vi "ADQUIRI_adq.vi"() -> ()   [LabVIEW 2019]
doc: "Programa que faz a leitura e a gravação em arquivo TXT de 13 canais provenientes da placa da National Instruments."
uses:
  <vilib>/Analysis/baseanly.llb/Mean (DBL).vi
  <vilib>/DAQmx/read.llb/DAQmx Read (Analog 2D DBL NChan NSamp).vi
  formato_aquisicao_global_adq.vi
  comunicacao.vi
  Aplicacao_atual_global_adq.vi
  <vilib>/DAQmx/configure/timing.llb/DAQmx Timing (Sample Clock).vi
  <vilib>/DAQmx/miscellaneous.llb/DAQmx Fill In Error Info.vi
  <vilib>/Utility/file.llb/Read Delimited Spreadsheet (string).vi
  <vilib>/Utility/file.llb/Write Delimited Spreadsheet (string).vi
  <vilib>/Analysis/NI_AALBase.lvlib
panel:
  in  "ValoresEnviados":cluster{"Pfundo[kPa]":dbl}
  out "SKS-NC-CV-006":bool
  out "comunica funcionando":bool
  in  "Valores":T1
  in  "Calibração":bool
  in  "COMUNICA":bool
  in  "data":dbl[][](array[numeric])
  out "DAQmx Task Name":refnum<k21>
  in  "Visualizar":bool
  out "led viewing":bool
  out "Configuração":string
  in  "Pontos No Gráfico":dbl(knob) scale=0.0..3000.0
  in  "Frequência":dbl=3000.0
  out "Ok":bool
  out "OK2":bool
  out "Ok R":bool
  out "OK2 R":bool
  out "P1-P2 RED":bool
  out "P2-P3 RED":bool
  out "P3-P4 RED":bool
  out "P34/L [Pa/m]":dbl
  out "P23/L [Pa/m]":dbl
  out "P12/L [Pa/m]":dbl
  out "Valor Teórico[Pa/m]":dbl
  out "P3-P4 VERDE":bool
  out "P2-P3 VERDE":bool
  out "P1-P2 VERDE":bool
  out "SKM-AI-KF-COR":dbl
  out "SKM-FI-WF":dbl format="%#.2g"
  out "SKM-FIC-KF-COR":dbl format="%#.2g"
  out "Valvulas":T2
  out "VALORES UDP":string[](array[string])
  in  "SAIR":bool
  out "reference out":refnum<vi>
  out "JG(m/s)":dbl
  in  "TempoAquisicao":dbl
  out "JW(m/s)":dbl format="%#.6g"
  out "JK(m/s)":dbl format="%#.6g"
  out "Timer":i32 caption="Elapsed Time (s)"
  in  "STOP":bool
  in  "COMEÇAR":bool
  out "Quantidade de\narquivos adquiridos":i64
  out "LED adquiri":bool
  out "Aquisição Automática":bool
  out "Linha de Teste":bool
  out "Matriz 2":dbl[][](array[numeric])
  out "error out":errorcluster
  in  "SKM-AI-KF_CORIOLI [kg/m³]":dbl
  in  "SKM-FIC-KF_CORIOLI [kg/s]":dbl
  in  "SIW-CV-001":bool
  in  "SIK-CV-001":bool
  in  "Entrada - SKM-FI-WF [CLP]":dbl
  in  "Escala de Calibracao - SKM-FI-WF":cluster{"Escala Max":dbl, "Escala Min":dbl}
  in  "Tab Control":enum32{"Gráfico", "Matriz"}(tab)
  out "Aplicação":string
  in  "Help":bool
  out "Gráfico":dbl[][](graph)
  in  "formato de aquisicao":bool
  out "C1-M corrente":dbl format="%#_4g"
  out "C1-J corrente":dbl format="%#_4g"
  out "C2-M corrente":dbl format="%#_4g"
  out "C2-J corrente":dbl format="%#_4g"
  out "C3-M corrente":dbl format="%#_4g"
  out "C3-J corrente":dbl format="%#_4g"
  out "C4-M corrente":dbl format="%#_4g"
  out "C4-J corrente":dbl format="%#_4g"
  out "P1 corrente":dbl format="%#_4g"
  out "P2 corrente":dbl format="%#_4g"
  out "P3 corrente":dbl format="%#_4g"
  out "P4 corrente":dbl format="%#_4g"
  out "Pfundo corrente":dbl format="%#_4g"
  out "P4(kPa)":dbl format="%#.2g"
  out "P3(kPa)":dbl format="%#.2g"
  out "P2(kPa)":dbl format="%#.2g"
  out "P1(kPa)":dbl format="%#.2g"
  out "Pfundo(kPa)":dbl format="%#.2g"
  out "P4":dbl format="%#_2g"
  out "C4-J":dbl format="%#_2g"
  out "C4-M":dbl format="%#_2g"
  out "C3-J":dbl format="%#_2g"
  out "P3":dbl format="%#_2g"
  out "C3-M":dbl format="%#_2g"
  out "Pfundo":dbl format="%#_2g"
  out "C2-J":dbl format="%#_2g"
  out "P2":dbl format="%#_2g"
  out "C2-M":dbl format="%#_2g"
  out "P1":dbl format="%#_2g"
  out "C1-M":dbl format="%#_2g"
  out "C1-J":dbl format="%#_2g"
  out "Matriz":dbl[][](array[numeric])
  # "[Hz]"
  # "Aquisição"
  # "[s]"
  # "m/s"
  # "m³/s"
  # "CHECK-UP"
  # "m/s"
  # "kg/s"
  # "P1, P3 & P4"
  # "[s]"
  # "m/s"
  # "kg/m³"
  # "P2"
  # "MIN"
  # "MAX"
  # "P1"
  # "kPa"
  # "P2"
  # "kPa"
  # "P3"
  # "kPa"
  # "P4"
  # "kPa"
  # "Pfundo"
  # "kPa"
  # "Variáveis Selecionadas Para Aquisição"
  # "[mA]"
  # "[V]"
  # "[mA]"
  # "[V]"
  # "[mA]"
  # "[V]"
  # "[kPa]"
  # "[mA]"
  # "[V]"
  # "[mA]"
  # "[V]"
  # "[mA]"
  # "[V]"
  # "[kPa]"
  # "[mA]"
  # "[V]"
  # "[mA]"
  # "[V]"
  # "[mA]"
  # "[V]"
  # "[kPa]"
  # "[mA]"
  # "[V]"
  # "[mA]"
  # "[V]"
  # "[mA]"
  # "[V]"
  # "[kPa]"
  # "[mA]"
  # "[V]"
  # "[kPa]"
  # "WIRELESS"
  # "NATIONAL"
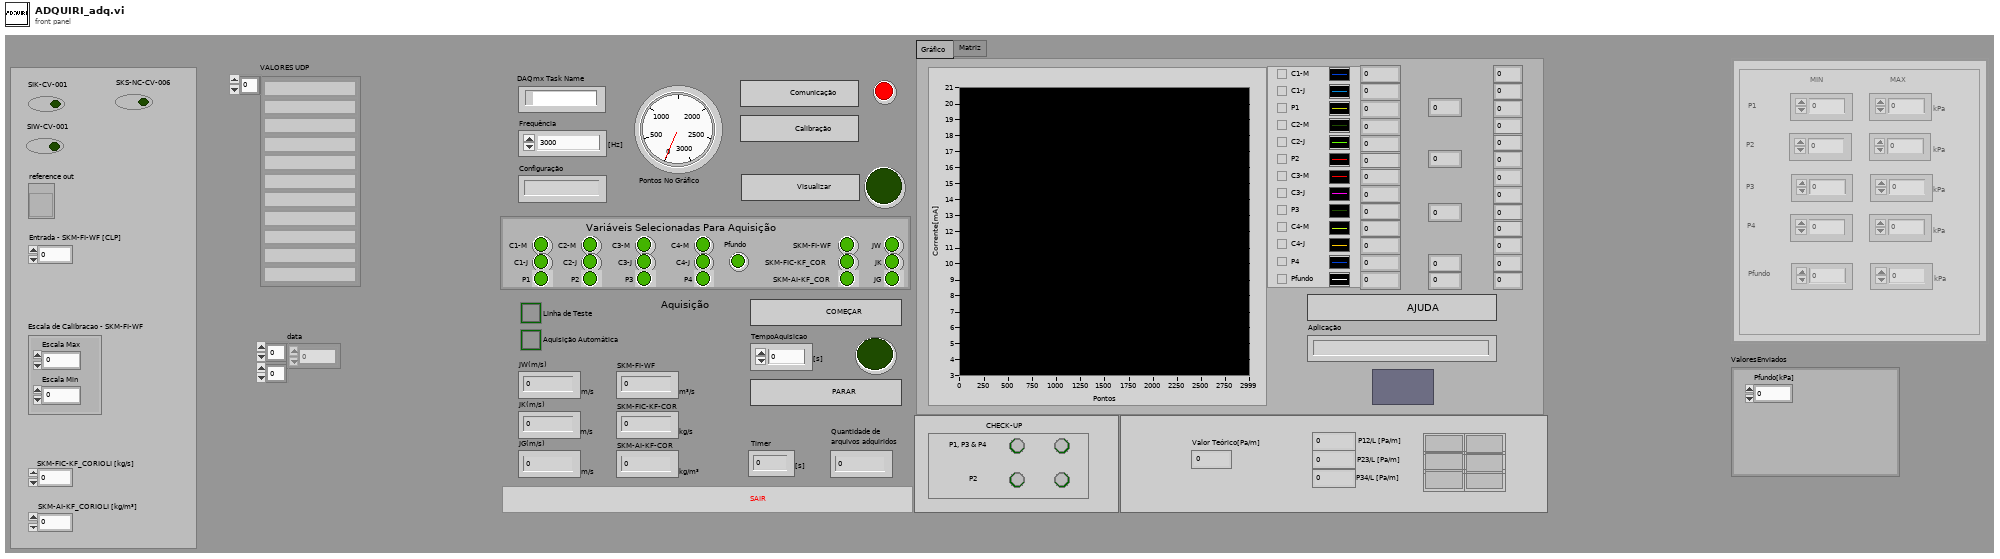
[diagram p1: front panel]
types:
  T1 = cluster{"P1 MIN":i32, "P1 MAX":i32, "P2 MIN":i32, "P2 MAX":i32, "P3 MIN":i32, "P3 MAX":i32, "P4 MIN":i32, "P4 MAX":i32, "Pfu MIN":i32, "Pfu MAX":i32}
  T2 = cluster{"C1-M":bool, "C1-J":bool, "P1":bool, "C2-M":bool, "C2-J":bool, "P2":bool, "C3-M":bool, "C3-J":bool, "P3":bool, "C4-M":bool, "C4-J":bool, "P4":bool, "Pfundo":bool, "JW":bool, "JK":bool, "JG":bool, "SKM-FI-WF":bool, "SKM-FIC-KF_COR":bool, "SKM-AI-KF_COR":bool}
  T3 = enum8{"Enabled", "Disabled", "Disabled and Grayed Out"}
  T4 = enum32{"Invalid", "Standard", "Closed", "Hidden", "Minimized", "Maximized"}
  T5 = enum32{"Bad", "Idle", "Run top level", "Running"}
  T6 = typedef "NI_Matrix.lvlib/RealMatrix.ctl" = dbl[][]
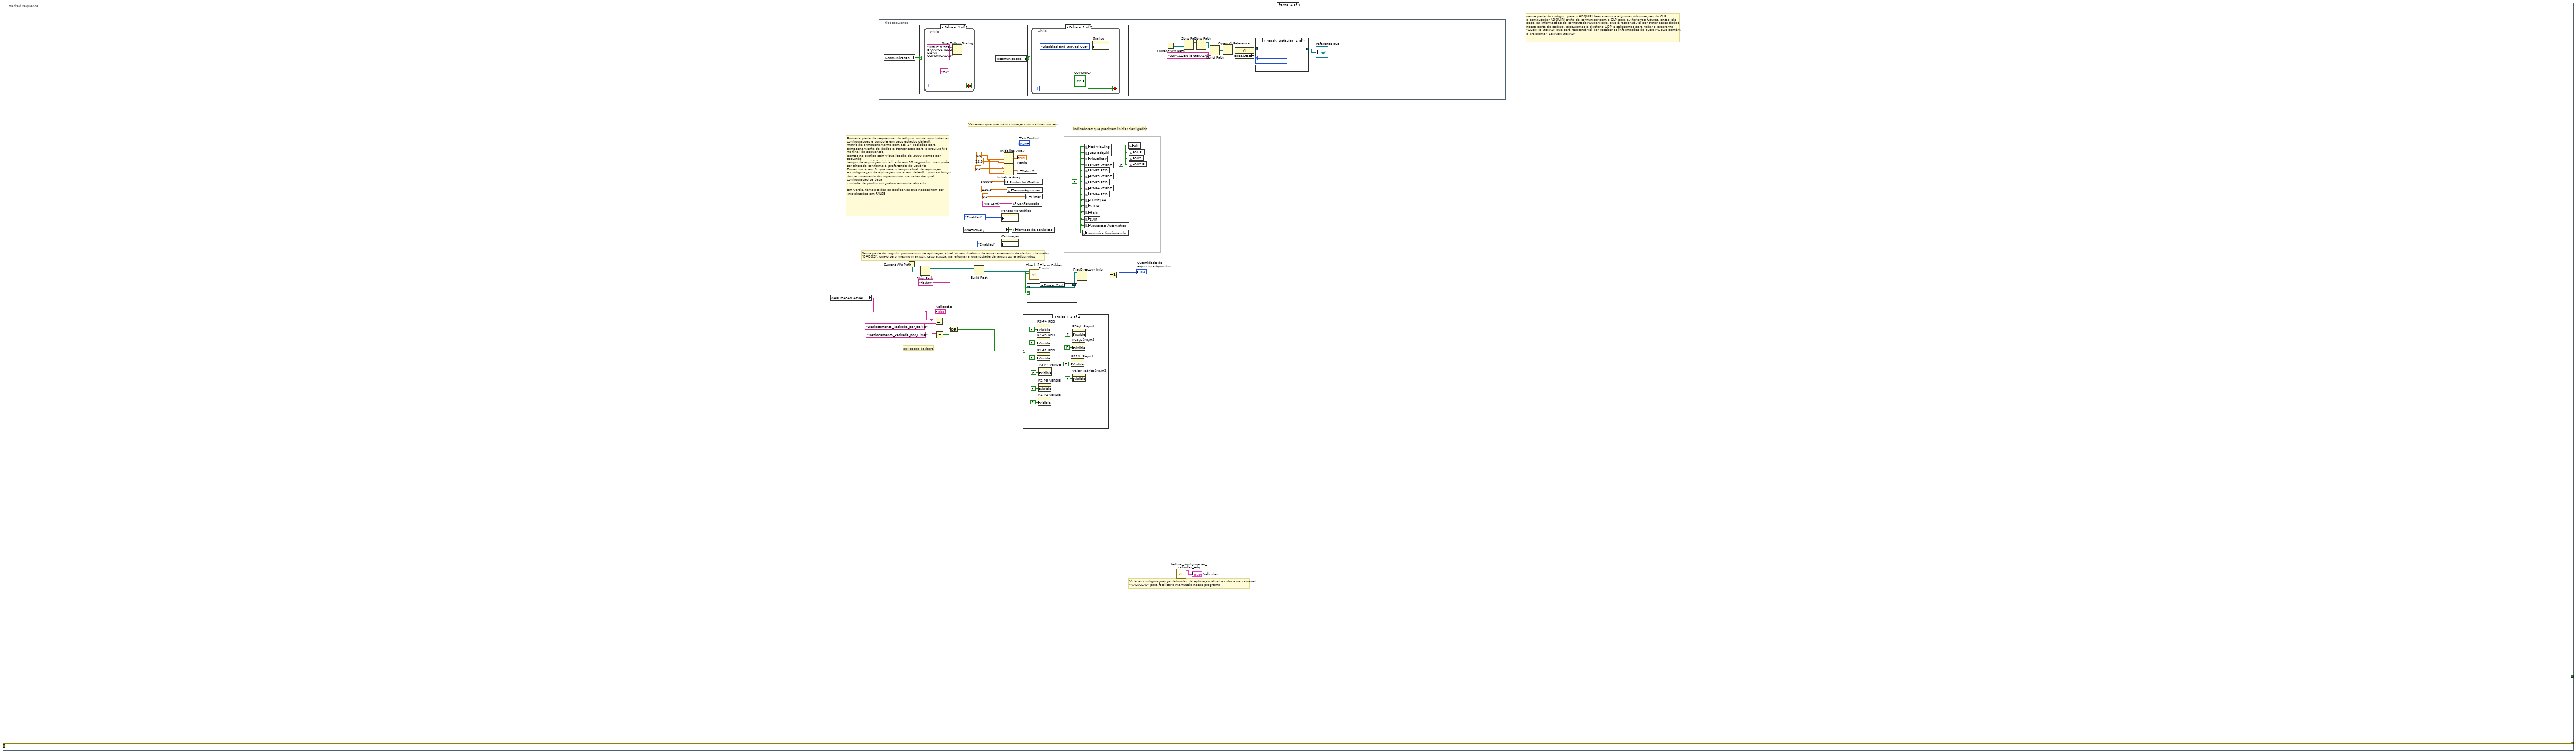
[diagram p2: hidden frame]
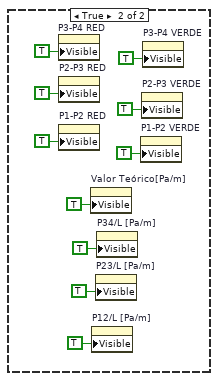
[diagram p3: hidden frame]
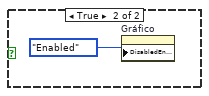
[diagram p5: hidden frame]
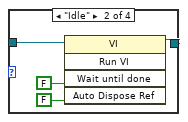
[diagram p6: hidden frame]
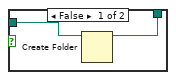
[diagram p9: hidden frame]
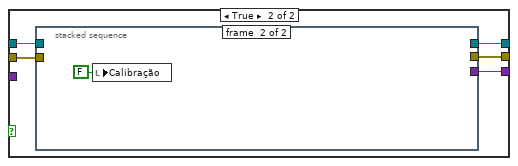
[diagram p10: hidden frame]
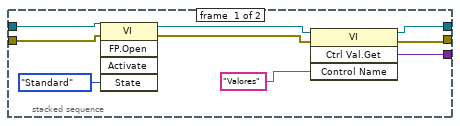
[diagram p11: hidden frame]
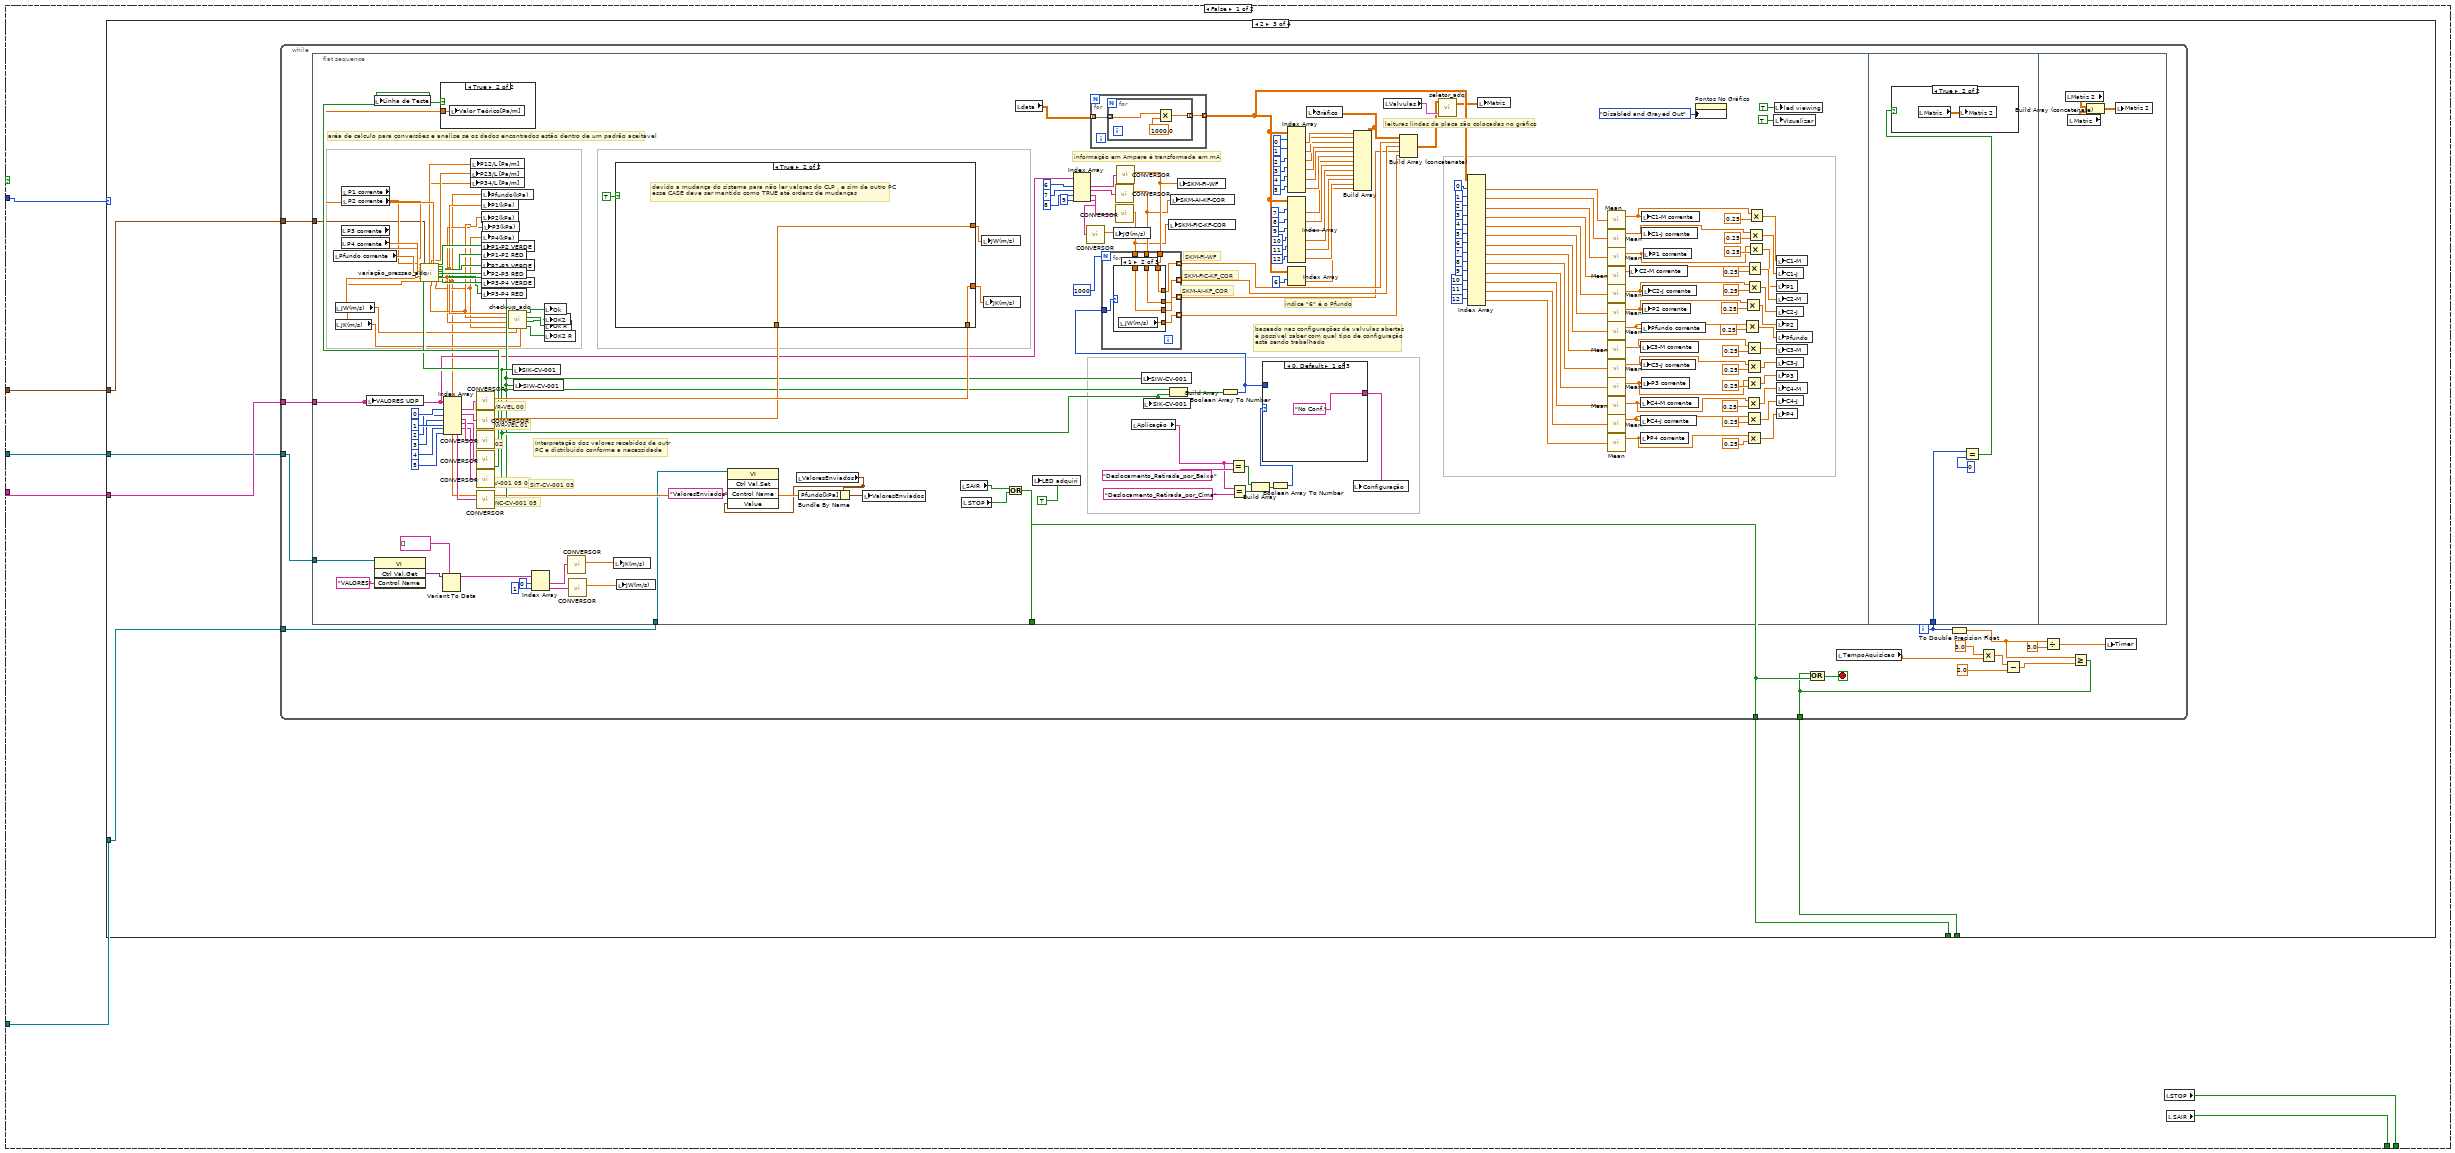
[diagram p12: hidden frame]
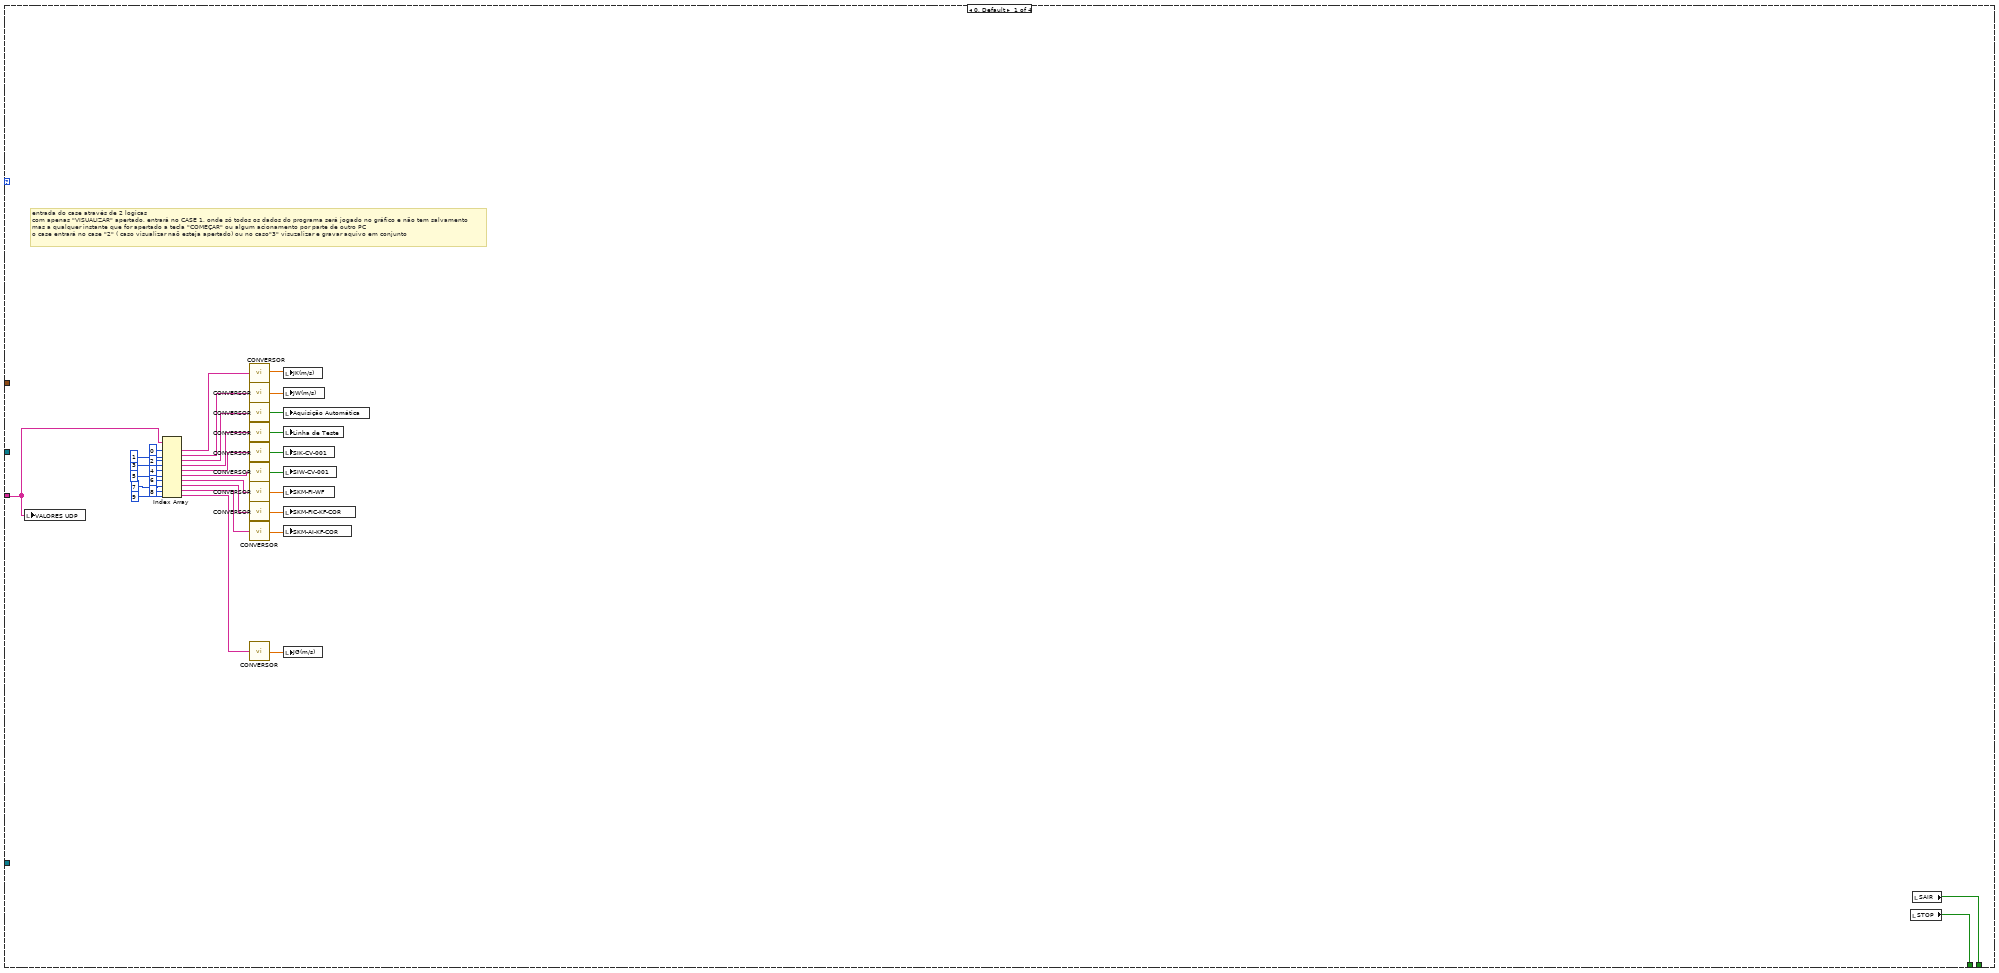
[diagram p13: hidden frame]
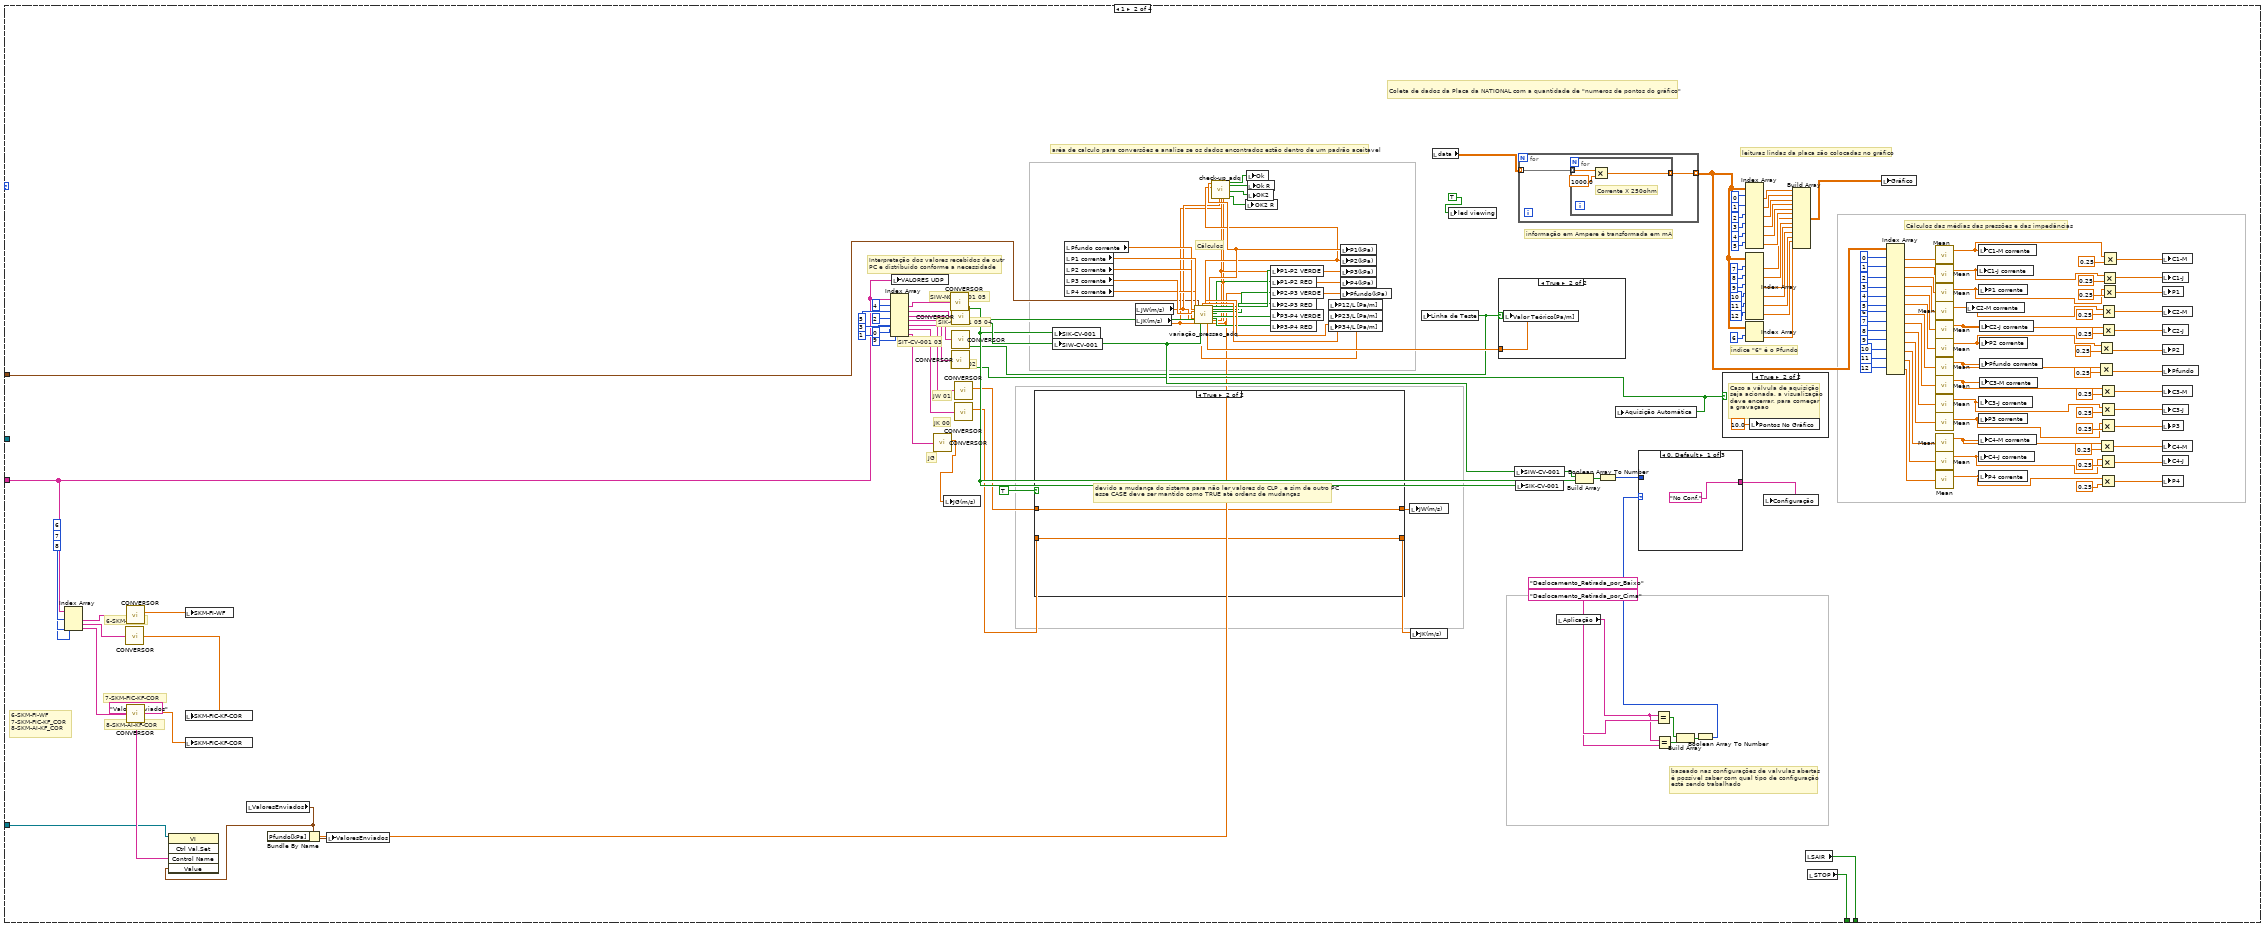
[diagram p14: hidden frame]
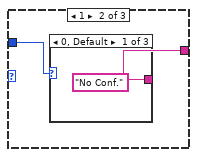
[diagram p15: hidden frame]
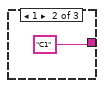
[diagram p16: hidden frame]
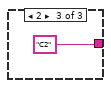
[diagram p17: hidden frame]
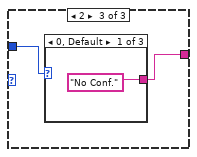
[diagram p18: hidden frame]
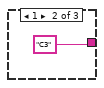
[diagram p19: hidden frame]
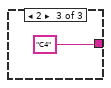
[diagram p20: hidden frame]
diagram:
  # "Abre a VI"
  n1 = property class="VI"("Front Panel.Open"=TRUE ("Front Panel Window:Open")) -> (error out=w1:errorcluster)  [unwired: 2 in, 1 out]
  n2 = flat-sequence {
    tunnel: [w5] -> w3
    tunnel: w1 -> [w4]
    tunnel: w3 -> [w1971]
    frame #0 {
      n3 = while {
        shift-right: [w8] -> w5
        shift-left: w4 -> [w7]
        stop <- w6 stop-if-true
        # "Loop responsável\npor manter o \nadquiri rodando\n\nmesmo após uma \naquisição ou \nvisualização dos \ndados\no adquiri não irá\nfechar, e irá \naguardar um novo\ncomando"
        n4 = stacked-sequence {
          tunnel: [w30 _ _ _] -> w8
          tunnel: w7 -> [w30 _ _ _]
          tunnel: [_ _ _ w1964] -> w6
          frame #0 {
            w20 = FALSE ("Visualisa")
            w36 = 0.0 ("element")
            w13 = FALSE ("Visualisa")
            w31 = 16.0 ("element")
            w37 = 0.0 ("element")
            # "aplicação barbara"
            # "Nessa parte do cógido, procuramos na aplicação atual, o seu diretório de armazenamento de dados, chamado\n\"DADOS\", cria-o se o mesmo n existir, caso exista, irá retornar a quantidade de arquivos ja adquiridos"
            # "Vi lê as configurações já definidas da aplicação atual e coloca na vairável\n\"VALVULAS\" para facilitar o manuzeio nesse programa"
            # "nessa parte do código , para o ADQUIRI teer acesso a algumas informações do CLP\no computador ADQUIRI evita de comunicar com o CLP para evitar erros futuros, então ele\npega as informações do computador SuperTorre, que é responsável por tratar esses dados\nnessa parte do código, procuramos o diretório UDP e colocamos para rodar o programa\n\"CLIENTE GERAL\" que será responsável por receber as informações do outro PC que contém\no programa\" SERVER GERAL\""
            # "Primeria parte da sequencia  do adquiri, inicia com todas as \nconfigurações e controle em seus estados default\nmatriz de armazenamento com até 17 posições para \narmazenamento de dados e transcrissão para o arquivo txt \nno final da sequencia\npontos no grafico com visualização de 3000 pontos por \nsegundo\ntempo de aquisição inicializado em 30 segundos, mas pode \nser alterado conforme a preferÊncia do usuário\nTimer inicia em 0, que será o tempo atual de aquisição\na configuração da aplicação inicia em default , pois ao longo \ndos acionamento do supervisório, irá saber de qual \nconfiguração se trata\ncontrole de pontos no gráfico encontra ativado\n\nem verde, temos todos os booleanos que necessitam ser\ninicializados em FALSE"
            # "Variáveis que precisam começar com valores iniciais"
            # "indicadores que precisam iniciar desligados"
            n5 = global read "Aplicacao_atual_global_adq.vi" "APLICACAO ATUAL"() -> (w9:string)
            "Aplicação" <- w9
            n6 = flat-sequence {
              frame #0 {
                n7 = global read "comunicacao.vi" "comunicacao"() -> (w60:bool)
                n8 = case shown="False" w60 {
                  frame False {
                    n9 = while {
                      stop <- w61 stop-if-true
                      n10 = One Button Dialog(message="LIGUE O SERVER E \nAPÓS ISSO,\n LIGAR COMUNICAÇÃO", button name ("OK")="OK") -> (true=w61:bool)
                    }
                  }
                  frame True {
                  }
                }
              }
              frame #1 {
                n11 = global read "comunicacao.vi" "comunicacao"() -> (w64:bool)
                n12 = case shown="False" w64 {
                  frame False {
                    n13 = while {
                      stop <- "COMUNICA" stop-if-true
                      n14 = property on="Gráfico" class="WFGraph (strict)"("DisabledEnum"=T3."Disabled and Grayed Out" ("Disabled")) -> ()  [unwired: 2 in, 2 out]
                    }
                  }
                  frame True {
                    n15 = property on="Gráfico" class="WFGraph (strict)"("DisabledEnum"=T3."Enabled" ("Disabled")) -> ()  [unwired: 2 in, 2 out]
                  }
                }
              }
              frame #2 {
                n16 = Current VI's Path() -> (path=w73:path)
                n17 = Strip Path(path=w73) -> (stripped path=w74:path)  [unwired: 1 out]
                n18 = Strip Path(path=w74) -> (stripped path=w75:path)  [unwired: 1 out]
                n19 = Build Path(base path=w75, name or relative path="UDP\\CLIENTE GERAL.vi") -> (appended path=w76:path)
                n20 = Open VI Reference(vi path=w76) -> (vi reference=w69:refnum<vi>)  [unwired: 5 in, 1 out]
                n21 = property class="VI"(reference=w69) -> (reference out=w70:refnum<vi>, "Exec.State"=w71:T5)  [unwired: 1 in, 1 out]
                n22 = case shown="\"Bad\", Default" w71 {
                  tunnel: w70 -> [w77 w79 w82 w83]
                  tunnel: [w77 w78 w82 w83] -> w68
                  frame "Bad", Default {
                  }
                  frame "Idle" {
                    n23 = invoke class="VI" method="Run VI"(reference=w79, "Wait until done"=FALSE ("Wait Until Done"), "Auto Dispose Ref"=FALSE ("Auto Dispose Reference")) -> (reference out=w78:refnum<vi>)  [unwired: 2 in, 4 out]
                  }
                  frame "Run top level" {
                  }
                  frame "Running" {
                  }
                }
                "reference out" <- w68
              }
            }
            n24 = Current VI's Path() -> (path=w29:path)
            n25 = Strip Path(path=w29) -> (stripped path=w28:path)  [unwired: 1 out]
            n26 = Equal?(x=w9, y="Deslocamento_Retirada_por_Baixo") -> (x = y?=w17:bool)
            n27 = Equal?(x=w9, y="Deslocamento_Retirada_por_Cima") -> (x = y?=w16:bool)
            n28 = Or(x=w17, y=w16) -> (x .or. y?=w15:bool)
            n29 = global read "formato_aquisicao_global_adq.vi" "NATIONAL/\nWIRELESS"() -> (w21:bool)
            n30 = Build Path(base path=w28, name or relative path="dados") -> (appended path=w24:path)
            n31 = property on="Pontos No Gráfico" class="Knob (strict)"("DisabledEnum"=T3."Enabled" ("Disabled")) -> ()  [unwired: 2 in, 2 out]
            n32 = property on="Calibração" class="Bool (strict)"("DisabledEnum"=T3."Enabled" ("Disabled")) -> ()  [unwired: 2 in, 2 out]
            n33 = Initialize Array(w37, w37, w31) -> (→"Matriz":dbl[][])
            n34 = Initialize Array(w36, w36, w31) -> (w35:dbl[][])
            n35 = local write "Pontos No Gráfico"(3000.0 ("Pontos no gráfico")) -> ()
            n36 = local write "TempoAquisicao"(120.0 ("Acquisition time")) -> ()
            n37 = local write "Configuração"("No Conf." ("Configuration")) -> ()
            n38 = local write "formato de aquisicao"(w21) -> ()
            n39 = local write "Matriz 2"(w35) -> ()
            n40 = case shown="False" w15 {
              frame False {
                n41 = property on="P3-P4 RED" class="Bool (strict)"("Visible"=FALSE) -> ()  [unwired: 2 in, 2 out]
                n42 = property on="P2-P3 RED" class="Bool (strict)"("Visible"=FALSE) -> ()  [unwired: 2 in, 2 out]
                n43 = property on="P1-P2 RED" class="Bool (strict)"("Visible"=FALSE) -> ()  [unwired: 2 in, 2 out]
                n44 = property on="P1-P2 VERDE" class="Bool (strict)"("Visible"=FALSE) -> ()  [unwired: 2 in, 2 out]
                n45 = property on="P2-P3 VERDE" class="Bool (strict)"("Visible"=FALSE) -> ()  [unwired: 2 in, 2 out]
                n46 = property on="P3-P4 VERDE" class="Bool (strict)"("Visible"=FALSE) -> ()  [unwired: 2 in, 2 out]
                n47 = property on="P12/L [Pa/m]" class="DigNum (strict)"("Visible"=FALSE) -> ()  [unwired: 2 in, 2 out]
                n48 = property on="P23/L [Pa/m]" class="DigNum (strict)"("Visible"=FALSE) -> ()  [unwired: 2 in, 2 out]
                n49 = property on="P34/L [Pa/m]" class="DigNum (strict)"("Visible"=FALSE) -> ()  [unwired: 2 in, 2 out]
                n50 = property on="Valor Teórico[Pa/m]" class="DigNum (strict)"("Visible"=FALSE) -> ()  [unwired: 2 in, 2 out]
              }
              frame True {
                n51 = property on="P3-P4 RED" class="Bool (strict)"("Visible"=TRUE) -> ()  [unwired: 2 in, 2 out]
                n52 = property on="P2-P3 RED" class="Bool (strict)"("Visible"=TRUE) -> ()  [unwired: 2 in, 2 out]
                n53 = property on="P1-P2 RED" class="Bool (strict)"("Visible"=TRUE) -> ()  [unwired: 2 in, 2 out]
                n54 = property on="Valor Teórico[Pa/m]" class="DigNum (strict)"("Visible"=TRUE) -> ()  [unwired: 2 in, 2 out]
                n55 = property on="P12/L [Pa/m]" class="DigNum (strict)"("Visible"=TRUE) -> ()  [unwired: 2 in, 2 out]
                n56 = property on="P23/L [Pa/m]" class="DigNum (strict)"("Visible"=TRUE) -> ()  [unwired: 2 in, 2 out]
                n57 = property on="P34/L [Pa/m]" class="DigNum (strict)"("Visible"=TRUE) -> ()  [unwired: 2 in, 2 out]
                n58 = property on="P1-P2 VERDE" class="Bool (strict)"("Visible"=TRUE) -> ()  [unwired: 2 in, 2 out]
                n59 = property on="P2-P3 VERDE" class="Bool (strict)"("Visible"=TRUE) -> ()  [unwired: 2 in, 2 out]
                n60 = property on="P3-P4 VERDE" class="Bool (strict)"("Visible"=TRUE) -> ()  [unwired: 2 in, 2 out]
              }
            }
            n61 = local write "Timer"(0.0 ("Timer")) -> ()
            n62 = call <vilib>:"Check if File or Folder Exists.vi"("path"=w24) -> ("file or folder exists?"=w27:bool, "dup path"=w26:path)  [unwired: 8 in, 1 out]
            n63 = case shown="True" w27 {
              tunnel: w26 -> [w85 w86]
              tunnel: [w84 w86] -> w25
              frame False {
                n64 = Create Folder(path (use dialog)=w85) -> (created path=w84:path)  [unwired: 2 in, 2 out]
              }
              frame True {
              }
            }
            n65 = File/Directory Info(path=w25) -> (size=w12:i64)  [unwired: 1 in, 6 out]
            n66 = local write "comunica funcionando"(w13) -> ()
            n67 = local write "led viewing"(w13) -> ()
            n68 = local write "LED adquiri"(w13) -> ()
            n69 = local write "Visualizar"(w13) -> ()
            n70 = local write "P1-P2 VERDE"(w13) -> ()
            n71 = local write "P1-P2 RED"(w13) -> ()
            n72 = local write "P2-P3 VERDE"(w13) -> ()
            n73 = local write "P2-P3 RED"(w13) -> ()
            n74 = local write "P3-P4 VERDE"(w13) -> ()
            n75 = local write "P3-P4 RED"(w13) -> ()
            n76 = local write "COMEÇAR"(w13) -> ()
            n77 = local write "STOP"(w13) -> ()
            n78 = local write "Help"(w13) -> ()
            n79 = local write "SAIR"(w13) -> ()
            n80 = local write "Aquisição Automática"(w13) -> ()
            n81 = Decrement(x=w12) -> (x-1=→"Quantidade de\narquivos adquiridos":i64)
            n82 = local write "Ok"(w20) -> ()
            n83 = local write "Ok R"(w20) -> ()
            n84 = local write "OK2"(w20) -> ()
            n85 = local write "OK2 R"(w20) -> ()
            n86 = call "leitura_configuracao_valvulas_adq.vi"() -> ("Valvulas"=→"Valvulas":T2)  [unwired: 6 in]
          }
          frame #1 {
            # "nessa etapa do programa, pegamos as referências dessas Vi\n\"LEITURA VALORES CLIENTE\" E \"CLIENTE GERAL\" que JÁ ESTÃO\nRODANDO EM OFF\ncom as refências em mãos, iremos jagá-las para dentro do loop"
            n87 = Current VI's Path() -> (path=w101:path)
            n88 = Current VI's Path() -> (path=w112:path)
            n89 = Strip Path(path=w112) -> (stripped path=w113:path)  [unwired: 1 out]
            n90 = Strip Path(path=w101) -> (stripped path=w95:path)  [unwired: 1 out]
            n91 = Strip Path(path=w113) -> (stripped path=w90:path)  [unwired: 1 out]
            n92 = Build Path(base path=w95, name or relative path="calibracao_adq.vi") -> (appended path=w99:path)
            n93 = Build Path(base path=w90, name or relative path="UDP\\ENVIA VALORES-CLIENTE.vi") -> (appended path=w89:path)
            n94 = Build Path(base path=w90, name or relative path="UDP\\LEITURA VALORES CLIENTE.vi") -> (appended path=w114:path)
            n95 = Build Path(base path=w90, name or relative path="UDP\\CLIENTE GERAL.vi") -> (appended path=w109:path)
            n96 = Open VI Reference(vi path=w89) -> (vi reference=w87:refnum<vi>)  [unwired: 5 in, 1 out]
            n97 = Open VI Reference(vi path=w99, error in (no error)=errorcluster {"status"=FALSE, "code"=0, "source"=""}) -> (vi reference=w98:refnum<vi>, error out=w97:errorcluster)  [unwired: 4 in]
            n98 = Open VI Reference(vi path=w114) -> (vi reference=w110:refnum<vi>)  [unwired: 5 in, 1 out]
            n99 = Open VI Reference(vi path=w109) -> (vi reference=w107:refnum<vi>)  [unwired: 5 in, 1 out]
            n100 = invoke class="VI" method="Run VI"(reference=w98, error in=w97, "Wait until done"=FALSE ("Wait Until Done"), "Auto Dispose Ref"=TRUE ("Auto Dispose Reference")) -> (reference out=w103:refnum<vi>, error out=w102:errorcluster)  [unwired: 1 in, 3 out]
            n101 = invoke class="VI" method="Ctrl Val.Get"(reference=w103, error in=w102, "Control Name"="Valores") -> (reference out=w93:refnum<vi>, error out=w92:errorcluster, "Get Control Value Variant"=w91:variant)  [unwired: 1 in, 1 out]
            n102 = while {
              tunnel: w110 -> [w115]
              tunnel: w107 -> [w141]
              shift-right: [w129] -> w94
              shift-left: w93 -> [w125]
              shift-right: [w128] -> _
              shift-left: w92 -> [w126]
              shift-right: [w124] -> _
              shift-left: w91 -> [w127]
              tunnel: w87 -> [w116]
              stop <- w156 stop-if-true
              w151 = FALSE ("visu led")
              # "10"
              # "national = TRUE"
              # "9"
              # "8"
              # "7"
              # "6"
              # "5"
              # "4"
              # "3"
              # "2"
              # "1"
              # "0"
              # "acionamento automático recebido de outro\nPC"
              # "Default dos botões"
              # "Caso as configurações não desejam\nincluir alguma velocidade na aquisição\na mesma será desabilitada"
              # "Coleta os valores das variáveis enviadas abaixo\nos valores são devolvidos na mesma ordem"
              # "Envia para o programa de comunicação com o outro computador\numa lista de nomes de variáveis que o ADQUIRE nessecita \nos nomes precisam ser enviados em array de STRING para o funcionamento\ndo programa de comunicação."
              # "ADQ 02"
              n103 = local read "Valvulas"() -> (w145:T2)
              n104 = local write "Ok R"(w151) -> ()
              n105 = local write "led viewing"(w151) -> ()
              n106 = local write "OK2"(w151) -> ()
              n107 = local write "OK2 R"(w151) -> ()
              n108 = local write "Ok"(w151) -> ()
              n109 = case shown="True" "Help" {
                frame False {
                  # "Botão Help destinado a abrir documentos e pesquisas relacionadas\nele também abre uma janela explicando sucintamente o objetivo do \nprograma ADQUIRE"
                }
                frame True {
                  n110 = stacked-sequence {
                    frame #0 {
                      n111 = Current VI's Path() -> (path=w1906:path)
                      n112 = Current VI's Path() -> (path=w1900:path)
                      n113 = Strip Path(path=w1906) -> (stripped path=w1905:path)  [unwired: 1 out]
                      n114 = Strip Path(path=w1900) -> (stripped path=w1899:path)  [unwired: 1 out]
                      n115 = Build Path(base path=w1905, name or relative path="Help_difinicao_adq.vi") -> (appended path=w1903:path)
                      n116 = Build Path(base path=w1899, name or relative path="help_pdfs_adq.vi") -> (appended path=w1897:path)
                      n117 = Open VI Reference(vi path=w1903) -> (vi reference=w1910:refnum<vi>, error out=w1909:errorcluster)  [unwired: 5 in]
                      n118 = Open VI Reference(vi path=w1897) -> (vi reference=w1908:refnum<vi>, error out=w1907:errorcluster)  [unwired: 5 in]
                      n119 = invoke class="VI" method="Run VI"(reference=w1910, error in=w1909, "Wait until done"=FALSE ("Wait Until Done"), "Auto Dispose Ref"=FALSE ("Auto Dispose Reference")) -> ()  [unwired: 1 in, 5 out]
                      n120 = invoke class="VI" method="Run VI"(reference=w1908, error in=w1907, "Wait until done"=FALSE ("Wait Until Done"), "Auto Dispose Ref"=FALSE ("Auto Dispose Reference")) -> ()  [unwired: 1 in, 5 out]
                    }
                    frame #1 {
                      n121 = local write "Help"(FALSE ("Help")) -> ()
                    }
                  }
                }
              }
              n122 = Unbundle By Name(w145) -> ("JW"=w146:bool, "JK"=w147:bool, "JG"=w148:bool)
              n123 = case shown="False" "Calibração" {
                tunnel: [w161 w169] -> w129
                tunnel: [w162 w168] -> w128
                tunnel: [w163 w167] -> w124
                tunnel: w125 -> [w160 w166]
                tunnel: w126 -> [w159 w165]
                tunnel: w127 -> [_ _]
                frame False {
                  n124 = invoke class="VI" method="Ctrl Val.Get"(reference=w160, error in=w159, "Control Name"="Valores") -> (reference out=w161:refnum<vi>, error out=w162:errorcluster, "Get Control Value Variant"=w163:variant)  [unwired: 1 in, 1 out]
                }
                frame True {
                  n125 = stacked-sequence {
                    tunnel: [w174 _] -> w169
                    tunnel: [w173 _] -> w168
                    tunnel: [w172 _] -> w167
                    tunnel: w166 -> [w171 _]
                    tunnel: w165 -> [w170 _]
                    frame #0 {
                      n126 = invoke class="VI" method="FP.Open"(reference=w171, error in=w170, "State"=T4."Standard") -> (reference out=w176:refnum<vi>, error out=w175:errorcluster)  [unwired: 2 in, 3 out]
                      n127 = invoke class="VI" method="Ctrl Val.Get"(reference=w176, error in=w175, "Control Name"="Valores") -> (reference out=w174:refnum<vi>, error out=w173:errorcluster, "Get Control Value Variant"=w172:variant)  [unwired: 1 in, 1 out]
                    }
                    frame #1 {
                      n128 = local write "Calibração"(FALSE ("Calibração")) -> ()
                    }
                  }
                }
              }
              n129 = case shown="True" w146 {
                frame False {
                  n130 = property on="JW(m/s)" class="DigNum (strict)"("DisabledEnum"=T3."Disabled and Grayed Out" ("Disabled")) -> ()  [unwired: 2 in, 2 out]
                }
                frame True {
                  n131 = property on="JW(m/s)" class="DigNum (strict)"("DisabledEnum"=T3."Enabled" ("Disabled")) -> ()  [unwired: 2 in, 2 out]
                }
              }
              n132 = case shown="True" w147 {
                frame False {
                  n133 = property on="JK(m/s)" class="DigNum (strict)"("DisabledEnum"=T3."Disabled and Grayed Out" ("Disabled")) -> ()  [unwired: 2 in, 2 out]
                }
                frame True {
                  n134 = property on="JK(m/s)" class="DigNum (strict)"("DisabledEnum"=T3."Enabled" ("Disabled")) -> ()  [unwired: 2 in, 2 out]
                }
              }
              n135 = case shown="True" w148 {
                frame False {
                  n136 = property on="JG(m/s)" class="DigNum (strict)"("DisabledEnum"=T3."Disabled and Grayed Out" ("Disabled")) -> ()  [unwired: 2 in, 2 out]
                }
                frame True {
                  n137 = property on="JG(m/s)" class="DigNum (strict)"("DisabledEnum"=T3."Enabled" ("Disabled")) -> ()  [unwired: 2 in, 2 out]
                }
              }
              n138 = invoke class="VI" method="Ctrl Val.Get"(reference=w115, "Control Name"="VALORES") -> ("Get Control Value Variant"=w144:variant)  [unwired: 2 in, 3 out]
              n139 = property on="Gráfico" class="WFGraph (strict)"("DisabledEnum"=T3."Enabled" ("Disabled")) -> ()  [unwired: 2 in, 2 out]
              n140 = Variant To Data(type=string[] [] ("Array"), Variant=w144) -> (data=w121:string[])  [unwired: 1 in, 1 out]
              n141 = To Variant(anything=string[] ["JK", "JW", "ADQ", "SIT-NC-CV-001", "SIK-NC-CV-001", "SIW-NC-CV-001", "SKM-FI-WF", "SKM-FIC-KF_COR", "SKM-AI-KF_COR", "JG", "SKS-NC-CV-006"] ("NOMES")) -> (Variant=w136:variant)
              n142 = invoke class="VI" method="Ctrl Val.Set"(reference=w141, "Control Name"="NOMES", "Value"=w136) -> ()  [unwired: 2 in, 5 out]
              n143 = Index Array(array=w121, index=2) -> (element=w139:string)
              n144 = call "CONVERSOR.vi"("String"=w139) -> ("boolean"=w138:bool)  [unwired: 6 in, 3 out]
              "Aquisição Automática" <- w138
              n145 = Not Equal?(x=w121, y="") -> (x != y?=w120:bool[])
              n146 = Get Variant Attribute(Variant=w124, name="Valores") -> ()  [unwired: 2 in, 4 out]
              n147 = Variant To Data(type="Valores", Variant=w124) -> (data=w122:T1)  [unwired: 1 in, 1 out]
              n148 = Index Array(array=w120, index=0) -> (element=→"comunica funcionando":bool)
              n149 = local write "Valores"(w122) -> ()
              n150 = global read "formato_aquisicao_global_adq.vi" "NATIONAL/\nWIRELESS"() -> (w135:bool)
              n151 = global write "formato_aquisicao_global_adq.vi" "NATIONAL/\nWIRELESS"("formato de aquisicao") -> ()
              n152 = Or(x="COMEÇAR", y=w138) -> (x .or. y?=w153:bool)
              n153 = Build Array("Visualizar", w153) -> (w158:bool[])
              n154 = Boolean Array To Number(Boolean array=w158) -> (number=w157:u32)
              n155 = case shown="True" w135 {
                tunnel: w157 -> [w183 w1004]
                tunnel: [w186 w1003] -> w155
                tunnel: [w185 w1002] -> w154
                tunnel: w121 -> [w184 w1001]
                tunnel: w122 -> [w182 w991]
                tunnel: w116 -> [w181 w990]
                tunnel: w115 -> [w180 w989]
                frame False {
                  n156 = case shown="2" w183 {
                    tunnel: [w219 w292 w438 w718] -> _
                    tunnel: [w218 w291 w437 w717] -> _
                    tunnel: w184 -> [w187 w316 w436 w716]
                    tunnel: w182 -> [_ w234 w435 w715]
                    tunnel: w181 -> [_ w222 w434 w714]
                    tunnel: w180 -> [_ _ w433 w713]
                    frame 0, Default {
                      # "entrada do case através de 2 logicas\ncom apenas \"VISUALIZAR\" apertado, entrará no CASE 1, onde só todos os dados do programa será jogado no gráfico e não tem salvamento\nmas a qualquer instante que for apertado a tecla \"COMEÇAR\" ou algum acionamento por parte de outro PC\no case entrará no case \"2\" ( caso visualizar naõ esteja apertado) ou no caso\"3\" visuzalizar e gravar aquivo em conjunto"
                      n157 = local write "VALORES UDP"(w187) -> ()
                      n158 = Index Array(array=w187, index #1=0 ("index"), index #2=1 ("index"), index #3=2 ("index"), index #4=3 ("index"), index #5=4 ("index"), index #6=5 ("index"), index #7=6 ("index"), index #8=7 ("index"), index #9=8 ("index"), index #10=9 ("index")) -> (element #1=w217:string, element #2=w216:string, element #3=w215:string, element #4=w214:string, element #5=w213:string, element #6=w212:string, element #7=w211:string, element #8=w210:string, element #9=w209:string, element #10=w208:string)
                      n159 = call "CONVERSOR.vi"("String"=w217) -> ("float"=w207:dbl)  [unwired: 6 in, 3 out]
                      n160 = call "CONVERSOR.vi"("String"=w216) -> ("float"=w206:dbl)  [unwired: 6 in, 3 out]
                      n161 = call "CONVERSOR.vi"("String"=w215) -> ("boolean"=w205:bool)  [unwired: 6 in, 3 out]
                      n162 = call "CONVERSOR.vi"("String"=w214) -> ("boolean"=w204:bool)  [unwired: 6 in, 3 out]
                      n163 = call "CONVERSOR.vi"("String"=w213) -> ("boolean"=w203:bool)  [unwired: 6 in, 3 out]
                      n164 = call "CONVERSOR.vi"("String"=w212) -> ("boolean"=w202:bool)  [unwired: 6 in, 3 out]
                      n165 = call "CONVERSOR.vi"("String"=w211) -> ("float"=w201:dbl)  [unwired: 6 in, 3 out]
                      n166 = call "CONVERSOR.vi"("String"=w210) -> ("float"=w200:dbl)  [unwired: 6 in, 3 out]
                      n167 = call "CONVERSOR.vi"("String"=w209) -> ("float"=w199:dbl)  [unwired: 6 in, 3 out]
                      n168 = call "CONVERSOR.vi"("String"=w208) -> ("float"=w198:dbl)  [unwired: 6 in, 3 out]
                      n169 = local write "JK(m/s)"(w207) -> ()
                      n170 = local write "JW(m/s)"(w206) -> ()
                      n171 = local write "Aquisição Automática"(w205) -> ()
                      n172 = local write "Linha de Teste"(w204) -> ()
                      n173 = local write "SIK-CV-001"(w203) -> ()
                      n174 = local write "SIW-CV-001"(w202) -> ()
                      n175 = local write "SKM-FI-WF"(w201) -> ()
                      n176 = local write "SKM-FIC-KF-COR"(w200) -> ()
                      n177 = local write "SKM-AI-KF-COR"(w199) -> ()
                      n178 = local write "JG(m/s)"(w198) -> ()
                      n179 = local read "STOP"() -> (w219:bool)
                      n180 = local read "SAIR"() -> (w218:bool)
                    }
                    frame 1 {
                      # "JG"
                      # "6-SKM-FI-WF"
                      # "7-SKM-FIC-KF-COR"
                      # "8-SKM-AI-KF-COR"
                      # "6-SKM-FI-WF\n7-SKM-FIC-KF_COR\n8-SKM-AI-KF_COR"
                      # "indice \"6\" é o Pfundo"
                      # "leituras lindas da placa são colocadas no gráfico"
                      # "baseado nas configurações de valvulas abertas\né possível saber com qual tipo de configuração \nestá sendo trabalhado"
                      # "aréa de calculo para conversões e analise se os dados encontrados estão dentro de um padrão aceitavel"
                      # "Interpretação dos valores recebidos de outr\nPC e distribuido conforme a necessidade"
                      # "informação em Ampere é transformada em mA"
                      # "Coleta de dados da Placa da NATIONAL com a quantidade de \"numeros de pontos do gráfico\""
                      # "ADQ 02"
                      # "SIW-NC-CV-001 05"
                      # "SIK-CV-001 05 04"
                      # "SIT-CV-001 03"
                      # "JW 01"
                      # "JK 00"
                      # "Cálculos das médias das pressões e das impedâncias"
                      # "Cálculos"
                      n181 = Index Array(array=w316, index #1=6 ("index"), index #2=7 ("index"), index #3=8 ("index")) -> (element #1=w312:string, element #2=w311:string, element #3=w310:string)
                      n182 = call "CONVERSOR.vi"("String"=w311) -> ("float"=w295:dbl)  [unwired: 6 in, 3 out]
                      n183 = call "CONVERSOR.vi"("String"=w312) -> ("float"=w296:dbl)  [unwired: 6 in, 3 out]
                      n184 = call "CONVERSOR.vi"("String"=w310) -> ("float"=w294:dbl)  [unwired: 6 in, 3 out]
                      n185 = local write "SKM-FI-WF"(w296) -> ()
                      n186 = local write "SKM-FIC-KF-COR"(w295) -> ()
                      n187 = local write "SKM-FIC-KF-COR"(w294) -> ()
                      n188 = local read "ValoresEnviados"() -> (w223:cluster{"Pfundo[kPa]":dbl})
                      n189 = invoke class="VI" method="Ctrl Val.Set"(reference=w222, "Control Name"="ValoresEnviados", "Value"=w223) -> ()  [unwired: 2 in, 5 out]
                      n190 = Index Array(array=w316, index #1=4 ("index"), index #2=5 ("index"), index #3=3 ("index"), index #4=2 ("index"), index #5=1 ("index"), index #6=0 ("index"), index #7=9 ("index")) -> (element #1=w332:string, element #2=w331:string, element #3=w328:string, element #4=w325:string, element #5=w321:string, element #6=w318:string, element #7=w308:string)
                      n191 = local write "VALORES UDP"(w316) -> ()
                      n192 = call "CONVERSOR.vi"("String"=w308) -> ("float"=w293:dbl)  [unwired: 6 in, 3 out]
                      n193 = local write "JG(m/s)"(w293) -> ()
                      n194 = call "CONVERSOR.vi"("String"=w332) -> ("boolean"=w327:bool)  [unwired: 6 in, 3 out]
                      n195 = call "CONVERSOR.vi"("String"=w325) -> ("boolean"=w324:bool)  [unwired: 6 in, 3 out]
                      n196 = call "CONVERSOR.vi"("String"=w331) -> ("boolean"=w330:bool)  [unwired: 6 in, 3 out]
                      n197 = call "CONVERSOR.vi"("String"=w328) -> ("boolean"=w306:bool)  [unwired: 6 in, 3 out]
                      n198 = call "CONVERSOR.vi"("String"=w321) -> ("float"=w320:dbl)  [unwired: 6 in, 3 out]
                      n199 = call "CONVERSOR.vi"("String"=w318) -> ("float"=w317:dbl)  [unwired: 6 in, 3 out]
                      n200 = case shown="True" TRUE {
                        tunnel: [w408 w423] -> w387
                        tunnel: [w407 w424] -> w386
                        tunnel: w320 -> [_ w424]
                        tunnel: w317 -> [_ w423]
                        frame False {
                          # "Cálculos de valores de velocidade utilizando informações do CLP"
                          # "área"
                          # "área"
                          n201 = local read "SKM-FIC-KF_CORIOLI [kg/s]"() -> (w404:dbl)
                          n202 = local read "SKM-AI-KF_CORIOLI [kg/m³]"() -> (w403:dbl)
                          n203 = local read "Escala de Calibracao - SKM-FI-WF"() -> (w406:cluster{"Escala Max":dbl, "Escala Min":dbl})
                          n204 = local read "Entrada - SKM-FI-WF [CLP]"() -> (w405:dbl)
                          n205 = local read "Escala de Calibracao - SKM-FI-WF"() -> (w414:cluster{"Escala Max":dbl, "Escala Min":dbl})
                          n206 = Unbundle By Name(w406) -> ("Escala Max"=w417:dbl, "Escala Min"=w416:dbl)
                          n207 = Bundle By Name(cluster=w414, "Escala Max"=0.001805556, "Escala Min"=0.0 ("Escala Max")) -> (w415:cluster{"Escala Max":dbl, "Escala Min":dbl})
                          n208 = Divide(x=w404, y=w403) -> (x/y=w422:dbl)
                          n209 = Divide(x=w422, y=0.0005107051557) -> (x/y=w408:dbl)
                          n210 = local write "Escala de Calibracao - SKM-FI-WF"(w415) -> ()
                          n211 = Subtract(x=w417, y=w416) -> (x-y=w418:dbl)
                          n212 = Divide(x=w418, y=4096.0) -> (x/y=w419:dbl)
                          n213 = Multiply(x=w419, y=w405) -> (x*y=w420:dbl)
                          n214 = Add(x=w420, y=w416) -> (x+y=w421:dbl)
                          n215 = Divide(x=w421, y=0.0005107051557) -> (x/y=w407:dbl)
                        }
                        frame True {
                          # "devido a mudança do sistema para não ler valores do CLP , e sim de outro PC\nesse CASE deve ser mantido como TRUE até ordens de mudanças"
                        }
                      }
                      n216 = local write "SIK-CV-001"(w327) -> ()
                      n217 = local write "SIW-CV-001"(w330) -> ()
                      n218 = local read "Pfundo corrente"() -> (w285:dbl)
                      n219 = local read "P1 corrente"() -> (w289:dbl)
                      n220 = local read "P2 corrente"() -> (w288:dbl)
                      n221 = local read "P3 corrente"() -> (w287:dbl)
                      n222 = local read "P4 corrente"() -> (w286:dbl)
                      n223 = local read "JW(m/s)"() -> (w236:dbl)
                      n224 = local read "JK(m/s)"() -> (w235:dbl)
                      n225 = call "variação_pressao_adq.vi"("P1(mA)"=w289, "P2(mA)"=w288, "P3(mA)"=w287, "P4(mA)"=w286, "PFUNDO(mA)"=w285, "JW(m/s)"=w236, "JK(m/s)"=w235, "Valores"=w234, "SIK-CV-001"=w327, "SIW-CV-001"=w330) -> ("P12/L12"=w305:dbl, "P34/L34"=w297:dbl, "P23/L23"=w304:dbl, "P2(kPa)"=w239:dbl, "VALOR TEORICO"=w389:dbl, "P3(kPa)"=w238:dbl, "P1(kPa)"=w240:dbl, "P4(kPa)"=w237:dbl, "P1-P2G"=w303:bool, "P2-P3R"=w302:bool, "P2-P3G"=w301:bool, "P1-P2R"=w300:bool, "P3-P4G"=w299:bool, "P3-P4R"=w298:bool, "PFUNDO(kPa)"=w221:dbl)  [unwired: 3 in]
                      n226 = Bundle By Name(cluster=w223, "Pfundo[kPa]"=w221) -> (w220:cluster{"Pfundo[kPa]":dbl})
                      n227 = local write "ValoresEnviados"(w220) -> ()
                      n228 = call "check-up_adq.vi"("JK(m/s)"=w235, "JW(m/s)"=w236, "P4(kPa)"=w237, "P3(kPa)"=w238, "P2(kPa)"=w239, "P1(kPa)"=w240) -> ("OK 2 R"=w241:bool, "OK 2 G"=w242:bool, "OK RED"=w243:bool, "OK G"=w244:bool)  [unwired: 2 in]
                      n229 = local write "OK2 R"(w241) -> ()
                      n230 = local write "Ok"(w244) -> ()
                      n231 = local write "Ok R"(w243) -> ()
                      n232 = local write "OK2"(w242) -> ()
                      n233 = local write "P1-P2 VERDE"(w303) -> ()
                      n234 = local write "P1-P2 RED"(w300) -> ()
                      n235 = local write "P2-P3 VERDE"(w301) -> ()
                      n236 = local write "P2-P3 RED"(w302) -> ()
                      n237 = local write "P3-P4 VERDE"(w299) -> ()
                      n238 = local write "P3-P4 RED"(w298) -> ()
                      n239 = local write "P12/L [Pa/m]"(w305) -> ()
                      n240 = local write "P23/L [Pa/m]"(w304) -> ()
                      n241 = local write "P34/L [Pa/m]"(w297) -> ()
                      n242 = local write "P1(kPa)"(w240) -> ()
                      n243 = local write "P2(kPa)"(w239) -> ()
                      n244 = local write "P3(kPa)"(w238) -> ()
                      n245 = local write "P4(kPa)"(w237) -> ()
                      n246 = local write "Pfundo(kPa)"(w221) -> ()
                      n247 = local write "JW(m/s)"(w386) -> ()
                      n248 = local write "JK(m/s)"(w387) -> ()
                      n249 = local write "Linha de Teste"(w306) -> ()
                      n250 = local read "data"() -> (w307:dbl[][])
                      n251 = local write "led viewing"(TRUE ("visu led")) -> ()
                      n252 = case shown="True" w306 {
                        tunnel: w389 -> [_ w427]
                        frame False {
                          n253 = local write "Valor Teórico[Pa/m]"(nan) -> ()
                        }
                        frame True {
                          n254 = local write "Valor Teórico[Pa/m]"(w427) -> ()
                        }
                      }
                      n255 = local write "SIW-CV-001"(w330) -> ()
                      n256 = local write "SIK-CV-001"(w327) -> ()
                      n257 = for {
                        tunnel: w307 -> [w428] mode=indexing
                        tunnel: [w429] -> w361 mode=indexing
                        n258 = for {
                          tunnel: w428 -> [w432] mode=indexing
                          tunnel: [w430] -> w429 mode=indexing
                          # "Corrente X 250ohm"
                          n259 = Multiply(x=w432, y=1000.0) -> (x*y=w430:dbl)
                        }
                      }
                      n260 = local read "Aplicação"() -> (w228:string)
                      n261 = Build Array(w330, w327) -> (w388:bool[])
                      n262 = Boolean Array To Number(Boolean array=w388) -> (number=w225:u32)
                      n263 = local write "Aquisição Automática"(w324) -> ()
                      n264 = Equal?(x=w228, y="Deslocamento_Retirada_por_Baixo") -> (x = y?=w230:bool)
                      n265 = Equal?(x=w228, y="Deslocamento_Retirada_por_Cima") -> (x = y?=w229:bool)
                      n266 = Build Array(w230, w229) -> (w231:bool[])
                      n267 = Boolean Array To Number(Boolean array=w231) -> (number=w226:u32)
                      n268 = case shown="0, Default" w226 {
                        tunnel: ["No Conf." w394 w399] -> w227
                        tunnel: w225 -> [_ w393 w398]
                        frame 0, Default {
                        }
                        frame 1 {
                          n269 = case shown="0, Default" w393 {
                            tunnel: ["No Conf." "C1" "C2"] -> w394
                            frame 0, Default {
                            }
                            frame 1 {
                            }
                            frame 2 {
                            }
                          }
                        }
                        frame 2 {
                          n270 = case shown="0, Default" w398 {
                            tunnel: ["No Conf." "C3" "C4"] -> w399
                            frame 0, Default {
                            }
                            frame 1 {
                            }
                            frame 2 {
                            }
                          }
                        }
                      }
                      n271 = case shown="True" w324 {
                        frame False {
                        }
                        frame True {
                          # "Caso a válvula de aquisição\nseja acionada, a visualização \ndeve encerrar, para começar\na gravaçaao"
                          n272 = local write "Pontos No Gráfico"(10.0 ("POINTS IN GRAPH")) -> ()
                        }
                      }
                      n273 = Index Array(array=w361, index (row) #1=0 ("index (row)"), index (row) #2=1 ("index (row)"), index (row) #3=2 ("index (row)"), index (row) #4=3 ("index (row)"), index (row) #5=4 ("index (row)"), index (row) #6=5 ("index (row)")) -> (element #1=w354:dbl[], element #2=w353:dbl[], element #3=w352:dbl[], element #4=w351:dbl[], element #5=w350:dbl[], element #6=w349:dbl[])  [unwired: 6 in]
                      n274 = Index Array(array=w361, index (row) #1=7 ("index (row)"), index (row) #2=8 ("index (row)"), index (row) #3=9 ("index (row)"), index (row) #4=10 ("index (row)"), index (row) #5=11 ("index (row)"), index (row) #6=12 ("index (row)")) -> (element #1=w342:dbl[], element #2=w341:dbl[], element #3=w340:dbl[], element #4=w339:dbl[], element #5=w338:dbl[], element #6=w337:dbl[])  [unwired: 6 in]
                      n275 = Index Array(array=w361, index (row)=6) -> (element=w335:dbl[])  [unwired: 1 in]
                      n276 = local write "Configuração"(w227) -> ()
                      n277 = Build Array(w354, w353, w352, w351, w350, w349, w342, w341, w340, w339, w338, w337, w335) -> (w290:dbl[][])
                      n278 = local read "SAIR"() -> (w291:bool)
                      n279 = local read "STOP"() -> (w292:bool)
                      n280 = local write "Gráfico"(w290) -> ()
                      n281 = Index Array(array=w361, index (row) #1=0 ("index (row)"), index (row) #2=1 ("index (row)"), index (row) #3=2 ("index (row)"), index (row) #4=3 ("index (row)"), index (row) #5=4 ("index (row)"), index (row) #6=5 ("index (row)"), index (row) #7=6 ("index (row)"), index (row) #8=7 ("index (row)"), index (row) #9=8 ("index (row)"), index (row) #10=9 ("index (row)"), index (row) #11=10 ("index (row)"), index (row) #12=11 ("index (row)"), index (row) #13=12 ("index (row)")) -> (element #1=w391:dbl[], element #2=w384:dbl[], element #3=w372:dbl[], element #4=w371:dbl[], element #5=w370:dbl[], element #6=w369:dbl[], element #7=w368:dbl[], element #8=w367:dbl[], element #9=w366:dbl[], element #10=w365:dbl[], element #11=w364:dbl[], element #12=w363:dbl[], element #13=w362:dbl[])  [unwired: 13 in]
                      n282 = call-poly <vilib>:"Mean.vi"("X"=w391) -> ("mean"=w270:dbl)  [unwired: 1 out]
                      n283 = call-poly <vilib>:"Mean.vi"("X"=w384) -> ("mean"=w269:dbl)  [unwired: 1 out]
                      n284 = call-poly <vilib>:"Mean.vi"("X"=w372) -> ("mean"=w268:dbl)  [unwired: 1 out]
                      n285 = call-poly <vilib>:"Mean.vi"("X"=w371) -> ("mean"=w267:dbl)  [unwired: 1 out]
                      n286 = call-poly <vilib>:"Mean.vi"("X"=w370) -> ("mean"=w266:dbl)  [unwired: 1 out]
                      n287 = call-poly <vilib>:"Mean.vi"("X"=w369) -> ("mean"=w265:dbl)  [unwired: 1 out]
                      n288 = call-poly <vilib>:"Mean.vi"("X"=w368) -> ("mean"=w264:dbl)  [unwired: 1 out]
                      n289 = call-poly <vilib>:"Mean.vi"("X"=w367) -> ("mean"=w263:dbl)  [unwired: 1 out]
                      n290 = call-poly <vilib>:"Mean.vi"("X"=w366) -> ("mean"=w262:dbl)  [unwired: 1 out]
                      n291 = call-poly <vilib>:"Mean.vi"("X"=w365) -> ("mean"=w261:dbl)  [unwired: 1 out]
                      n292 = call-poly <vilib>:"Mean.vi"("X"=w364) -> ("mean"=w260:dbl)  [unwired: 1 out]
                      n293 = call-poly <vilib>:"Mean.vi"("X"=w363) -> ("mean"=w259:dbl)  [unwired: 1 out]
                      n294 = call-poly <vilib>:"Mean.vi"("X"=w362) -> ("mean"=w258:dbl)  [unwired: 1 out]
                      n295 = local write "C2-M corrente"(w267) -> ()
                      n296 = local write "C1-J corrente"(w269) -> ()
                      n297 = local write "C1-M corrente"(w270) -> ()
                      n298 = local write "C4-J corrente"(w259) -> ()
                      n299 = local write "P1 corrente"(w268) -> ()
                      n300 = local write "C3-J corrente"(w262) -> ()
                      n301 = local write "P3 corrente"(w261) -> ()
                      n302 = local write "C4-M corrente"(w260) -> ()
                      n303 = local write "P4 corrente"(w258) -> ()
                      n304 = local write "C2-J corrente"(w266) -> ()
                      n305 = local write "P2 corrente"(w265) -> ()
                      n306 = local write "Pfundo corrente"(w264) -> ()
                      n307 = local write "C3-M corrente"(w263) -> ()
                      n308 = Multiply(x=w264, y=0.25) -> (x*y=w248:dbl)
                      n309 = Multiply(x=w265, y=0.25) -> (x*y=w249:dbl)
                      n310 = Multiply(x=w260, y=0.25) -> (x*y=w255:dbl)
                      n311 = Multiply(x=w263, y=0.25) -> (x*y=w247:dbl)
                      n312 = Multiply(x=w262, y=0.25) -> (x*y=w246:dbl)
                      n313 = Multiply(x=w261, y=0.25) -> (x*y=w245:dbl)
                      n314 = Multiply(x=w259, y=0.25) -> (x*y=w256:dbl)
                      n315 = Multiply(x=w258, y=0.25) -> (x*y=w257:dbl)
                      n316 = Multiply(x=w267, y=0.25) -> (x*y=w251:dbl)
                      n317 = Multiply(x=w266, y=0.25) -> (x*y=w250:dbl)
                      n318 = Multiply(x=w269, y=0.25) -> (x*y=w253:dbl)
                      n319 = Multiply(x=w268, y=0.25) -> (x*y=w252:dbl)
                      n320 = Multiply(x=w270, y=0.25) -> (x*y=w254:dbl)
                      n321 = local write "C1-M"(w254) -> ()
                      n322 = local write "C1-J"(w253) -> ()
                      n323 = local write "P1"(w252) -> ()
                      n324 = local write "C2-M"(w251) -> ()
                      n325 = local write "C2-J"(w250) -> ()
                      n326 = local write "P2"(w249) -> ()
                      n327 = local write "Pfundo"(w248) -> ()
                      n328 = local write "C3-M"(w247) -> ()
                      n329 = local write "C3-J"(w246) -> ()
                      n330 = local write "P3"(w245) -> ()
                      n331 = local write "C4-M"(w255) -> ()
                      n332 = local write "C4-J"(w256) -> ()
                      n333 = local write "P4"(w257) -> ()
                    }
                    frame 2 {
                      n334 = while {
                        tunnel: [w454] -> w438
                        tunnel: [w443] -> w437
                        tunnel: w436 -> [w452]
                        tunnel: w435 -> [w441]
                        tunnel: w434 -> [w440]
                        tunnel: w433 -> [w439]
                        i -> [w445]
                        stop <- w453 stop-if-true
                        n335 = flat-sequence {
                          tunnel: [w617] -> w454
                          tunnel: w452 -> [w570]
                          tunnel: w441 -> [w480]
                          tunnel: w440 -> [w467]
                          tunnel: w439 -> [w456]
                          tunnel: w445 -> [w708]
                          frame #0 {
                            # "Interpretação dos valores recebidos de outr\nPC e distribuido conforme a necessidade"
                            # "aréa de calculo para conversões e analise se os dados encontrados estão dentro de um padrão aceitavel"
                            # "baseado nas configurações de valvulas abertas\né possível saber com qual tipo de configuração \nestá sendo trabalhado"
                            # "informação em Ampere é transformada em mA"
                            # "indice \"6\" é o Pfundo"
                            # "leituras lindas da placa são colocadas no gráfico"
                            # "SIW-NC-CV-001 05"
                            # "SIK-CV-001 05 04"
                            # "SIT-CV-001 03"
                            # "ADQ 02"
                            # "SPW-WR-VEL 01"
                            # "SPK-WR-VEL 00"
                            # "SKM-FI-WF"
                            # "SKM-FIC-KF_COR"
                            # "SKM-AI-KF_COR"
                            n336 = local read "Pfundo corrente"() -> (w537:dbl)
                            n337 = local read "JW(m/s)"() -> (w482:dbl)
                            n338 = local read "JK(m/s)"() -> (w481:dbl)
                            n339 = local read "P3 corrente"() -> (w535:dbl)
                            n340 = local read "P4 corrente"() -> (w536:dbl)
                            n341 = local read "P1 corrente"() -> (w533:dbl)
                            n342 = local read "P2 corrente"() -> (w534:dbl)
                            n343 = local write "VALORES UDP"(w570) -> ()
                            n344 = invoke class="VI" method="Ctrl Val.Get"(reference=w456, "Control Name"="VALORES") -> ("Get Control Value Variant"=w460:variant)  [unwired: 2 in, 3 out]
                            n345 = Variant To Data(type=string[] [] ("Array"), Variant=w460) -> (data=w461:string[])  [unwired: 1 in, 1 out]
                            n346 = Index Array(array=w570, index #1=0 ("index"), index #2=1 ("index"), index #3=2 ("index"), index #4=3 ("index"), index #5=4 ("index"), index #6=5 ("index")) -> (element #1=w582:string, element #2=w581:string, element #3=w580:string, element #4=w579:string, element #5=w578:string, element #6=w577:string)
                            n347 = call "CONVERSOR.vi"("String"=w581) -> ("float"=w574:dbl)  [unwired: 6 in, 3 out]
                            n348 = call "CONVERSOR.vi"("String"=w580) -> ()  [unwired: 6 in, 4 out]
                            n349 = call "CONVERSOR.vi"("String"=w578) -> ("boolean"=w572:bool)  [unwired: 6 in, 3 out]
                            n350 = call "CONVERSOR.vi"("String"=w577) -> ("boolean"=w571:bool)  [unwired: 6 in, 3 out]
                            n351 = call "variação_pressao_adq.vi"("P1(mA)"=w533, "P2(mA)"=w534, "P3(mA)"=w535, "P4(mA)"=w536, "PFUNDO(mA)"=w537, "JW(m/s)"=w482, "JK(m/s)"=w481, "Valores"=w480, "SIK-CV-001"=w572, "SIW-CV-001"=w571) -> ("P12/L12"=w540:dbl, "P34/L34"=w538:dbl, "P23/L23"=w539:dbl, "P2(kPa)"=w485:dbl, "VALOR TEORICO"=w547:dbl, "P3(kPa)"=w484:dbl, "P1(kPa)"=w486:dbl, "P4(kPa)"=w483:dbl, "P1-P2G"=w546:bool, "P2-P3R"=w545:bool, "P2-P3G"=w544:bool, "P1-P2R"=w543:bool, "P3-P4G"=w542:bool, "P3-P4R"=w541:bool, "PFUNDO(kPa)"=w469:dbl)  [unwired: 3 in]
                            n352 = local write "P23/L [Pa/m]"(w539) -> ()
                            n353 = local write "P34/L [Pa/m]"(w538) -> ()
                            n354 = local write "P12/L [Pa/m]"(w540) -> ()
                            n355 = call "CONVERSOR.vi"("String"=w582) -> ("float"=w575:dbl)  [unwired: 6 in, 3 out]
                            n356 = call "CONVERSOR.vi"("String"=w579) -> ("boolean"=w573:bool)  [unwired: 6 in, 3 out]
                            n357 = local write "Linha de Teste"(w573) -> ()
                            n358 = case shown="True" w573 {
                              tunnel: w547 -> [_ w683]
                              frame False {
                                n359 = local write "Valor Teórico[Pa/m]"(nan) -> ()
                              }
                              frame True {
                                n360 = local write "Valor Teórico[Pa/m]"(w683) -> ()
                              }
                            }
                            n361 = local write "P1-P2 VERDE"(w546) -> ()
                            n362 = local write "P1-P2 RED"(w543) -> ()
                            n363 = local write "P2-P3 VERDE"(w544) -> ()
                            n364 = local write "P2-P3 RED"(w545) -> ()
                            n365 = local write "P3-P4 VERDE"(w542) -> ()
                            n366 = local write "P3-P4 RED"(w541) -> ()
                            n367 = local write "Pfundo(kPa)"(w469) -> ()
                            n368 = local write "P1(kPa)"(w486) -> ()
                            n369 = local write "P2(kPa)"(w485) -> ()
                            n370 = local write "P4(kPa)"(w483) -> ()
                            n371 = local write "P3(kPa)"(w484) -> ()
                            n372 = call "check-up_adq.vi"("JK(m/s)"=w481, "JW(m/s)"=w482, "P4(kPa)"=w483, "P3(kPa)"=w484, "P2(kPa)"=w485, "P1(kPa)"=w486) -> ("OK 2 R"=w487:bool, "OK 2 G"=w488:bool, "OK RED"=w489:bool, "OK G"=w490:bool)  [unwired: 2 in]
                            n373 = local write "SIK-CV-001"(w572) -> ()
                            n374 = local write "SIW-CV-001"(w571) -> ()
                            n375 = Index Array(array=w461, index #1=0 ("index"), index #2=1 ("index")) -> (element #1=w462:string, element #2=w463:string)
                            n376 = local write "Ok"(w490) -> ()
                            n377 = local write "OK2"(w488) -> ()
                            n378 = local write "Ok R"(w489) -> ()
                            n379 = local write "OK2 R"(w487) -> ()
                            n380 = call "CONVERSOR.vi"("String"=w462) -> ("float"=w464:dbl)  [unwired: 6 in, 3 out]
                            n381 = call "CONVERSOR.vi"("String"=w463) -> ("float"=w465:dbl)  [unwired: 6 in, 3 out]
                            n382 = local write "JK(m/s)"(w464) -> ()
                            n383 = case shown="True" TRUE {
                              tunnel: [w679 w681] -> w530
                              tunnel: [w672 w680] -> w531
                              tunnel: w575 -> [_ w681]
                              tunnel: w574 -> [_ w680]
                              frame False {
                                n384 = local read "Escala de Calibracao - SKM-FI-WF"() -> (w668:cluster{"Escala Max":dbl, "Escala Min":dbl})
                                n385 = local read "Entrada - SKM-FI-WF [CLP]"() -> (w666:dbl)
                                n386 = local read "Escala de Calibracao - SKM-FI-WF"() -> (w673:cluster{"Escala Max":dbl, "Escala Min":dbl})
                                n387 = Bundle By Name(cluster=w673, "Escala Max"=0.001805556, "Escala Min"=0.0 ("Escala Max")) -> (w674:cluster{"Escala Max":dbl, "Escala Min":dbl})
                                n388 = local write "Escala de Calibracao - SKM-FI-WF"(w674) -> ()
                                n389 = Unbundle By Name(w668) -> ("Escala Max"=w662:dbl, "Escala Min"=w667:dbl)
                                n390 = local read "SKM-AI-KF_CORIOLI [kg/m³]"() -> (w676:dbl)
                                n391 = local read "SKM-FIC-KF_CORIOLI [kg/s]"() -> (w677:dbl)
                                n392 = Subtract(x=w662, y=w667) -> (x-y=w660:dbl)
                                n393 = Divide(x=w660, y=4096.0) -> (x/y=w669:dbl)
                                n394 = Multiply(x=w669, y=w666) -> (x*y=w670:dbl)
                                n395 = Add(x=w670, y=w667) -> (x+y=w671:dbl)
                                n396 = Divide(x=w677, y=w676) -> (x/y=w678:dbl)
                                n397 = Divide(x=w671, y=0.0005107051557) -> (x/y=w672:dbl)
                                n398 = Divide(x=w678, y=0.0005107051557) -> (x/y=w679:dbl)
                              }
                              frame True {
                                # "devido a mudança do sistema para não ler valores do CLP , e sim de outro PC\nesse CASE deve ser mantido como TRUE até ordens de mudanças"
                              }
                            }
                            n399 = local write "JW(m/s)"(w465) -> ()
                            n400 = local read "ValoresEnviados"() -> (w468:cluster{"Pfundo[kPa]":dbl})
                            n401 = invoke class="VI" method="Ctrl Val.Set"(reference=w467, "Control Name"="ValoresEnviados", "Value"=w468) -> ()  [unwired: 2 in, 5 out]
                            n402 = Bundle By Name(cluster=w468, "Pfundo[kPa]"=w469) -> (w466:cluster{"Pfundo[kPa]":dbl})
                            n403 = local write "ValoresEnviados"(w466) -> ()
                            n404 = local read "SAIR"() -> (w615:bool)
                            n405 = local read "STOP"() -> (w616:bool)
                            n406 = local write "JW(m/s)"(w531) -> ()
                            n407 = local write "JK(m/s)"(w530) -> ()
                            n408 = Or(x=w615, y=w616) -> (x .or. y?=w617:bool)
                            n409 = local read "data"() -> (w549:dbl[][])
                            n410 = local write "LED adquiri"(TRUE ("Adquire")) -> ()
                            n411 = Index Array(array=w570, index #1=6 ("index"), index #2=7 ("index"), index #3=8 ("index"), index #4=9 ("index")) -> (element #1=w566:string, element #2=w565:string, element #3=w564:string, element #4=w551:string)
                            n412 = call "CONVERSOR.vi"("String"=w551) -> ("float"=w550:dbl)  [unwired: 6 in, 3 out]
                            n413 = for {
                              tunnel: [w702] -> w618 mode=indexing
                              tunnel: w549 -> [w701] mode=indexing
                              n414 = for {
                                tunnel: w701 -> [w705] mode=indexing
                                tunnel: [w703] -> w702 mode=indexing
                                n415 = Multiply(x=w705, y=1000.0) -> (x*y=w703:dbl)
                              }
                            }
                            n416 = local write "JG(m/s)"(w550) -> ()
                            n417 = call "CONVERSOR.vi"("String"=w565) -> ("float"=w554:dbl)  [unwired: 6 in, 3 out]
                            n418 = call "CONVERSOR.vi"("String"=w564) -> ("float"=w553:dbl)  [unwired: 6 in, 3 out]
                            n419 = call "CONVERSOR.vi"("String"=w566) -> ("float"=w555:dbl)  [unwired: 6 in, 3 out]
                            n420 = local read "Aplicação"() -> (w474:string)
                            n421 = local write "SIW-CV-001"(w571) -> ()
                            n422 = local write "SIK-CV-001"(w572) -> ()
                            n423 = local write "SKM-FIC-KF-COR"(w553) -> ()
                            n424 = Build Array(w571, w572) -> (w646:bool[])
                            n425 = local write "SKM-AI-KF-COR"(w554) -> ()
                            n426 = local write "SKM-FI-WF"(w555) -> ()
                            n427 = Boolean Array To Number(Boolean array=w646) -> (number=w471:u32)
                            n428 = for {
                              N: 1000 -> [_]
                              tunnel: [w690] -> w557 mode=indexing
                              tunnel: w471 -> [w691]
                              tunnel: w553 -> [w686]
                              tunnel: w554 -> [w685]
                              tunnel: w555 -> [w684]
                              tunnel: [w689] -> w558 mode=indexing
                              tunnel: [w688] -> w559 mode=indexing
                              tunnel: [w687] -> w560 mode=indexing
                              n429 = case shown="1" w691 {
                                tunnel: [w692 w696 w700] -> w690
                                tunnel: [w692 w695 w699] -> w689
                                tunnel: [w692 w694 w698] -> w688
                                tunnel: [w692 w693 w697] -> w687
                                tunnel: w686 -> [_ w695 w699]
                                tunnel: w685 -> [_ w694 w698]
                                tunnel: w684 -> [_ w693 w697]
                                frame 0, Default {
                                w692 = nan
                                }
                                frame 1 {
                                n430 = local read "JW(m/s)"() -> (w696:dbl)
                                }
                                frame 2 {
                                n431 = local read "JK(m/s)"() -> (w700:dbl)
                                }
                              }
                            }
                            n432 = Equal?(x=w474, y="Deslocamento_Retirada_por_Baixo") -> (x = y?=w476:bool)
                            n433 = Equal?(x=w474, y="Deslocamento_Retirada_por_Cima") -> (x = y?=w475:bool)
                            n434 = Build Array(w476, w475) -> (w477:bool[])
                            n435 = Boolean Array To Number(Boolean array=w477) -> (number=w473:u32)
                            n436 = case shown="0, Default" w473 {
                              tunnel: ["No Conf." w651 w656] -> w472
                              tunnel: w471 -> [_ w650 w655]
                              frame 0, Default {
                              }
                              frame 1 {
                                n437 = case shown="0, Default" w650 {
                                tunnel: ["No Conf." "C1" "C2"] -> w651
                                frame 0, Default {
                                }
                                frame 1 {
                                }
                                frame 2 {
                                }
                                }
                              }
                              frame 2 {
                                n438 = case shown="0, Default" w655 {
                                tunnel: ["No Conf." "C3" "C4"] -> w656
                                frame 0, Default {
                                }
                                frame 1 {
                                }
                                frame 2 {
                                }
                                }
                              }
                            }
                            n439 = Index Array(array=w618, index (row) #1=0 ("index (row)"), index (row) #2=1 ("index (row)"), index (row) #3=2 ("index (row)"), index (row) #4=3 ("index (row)"), index (row) #5=4 ("index (row)"), index (row) #6=5 ("index (row)")) -> (element #1=w608:dbl[], element #2=w607:dbl[], element #3=w606:dbl[], element #4=w605:dbl[], element #5=w604:dbl[], element #6=w603:dbl[])  [unwired: 6 in]
                            n440 = Index Array(array=w618, index (row) #1=7 ("index (row)"), index (row) #2=8 ("index (row)"), index (row) #3=9 ("index (row)"), index (row) #4=10 ("index (row)"), index (row) #5=11 ("index (row)"), index (row) #6=12 ("index (row)")) -> (element #1=w596:dbl[], element #2=w595:dbl[], element #3=w594:dbl[], element #4=w593:dbl[], element #5=w592:dbl[], element #6=w591:dbl[])  [unwired: 6 in]
                            n441 = Index Array(array=w618, index (row)=6) -> (element=w589:dbl[])  [unwired: 1 in]
                            n442 = local write "Configuração"(w472) -> ()
                            n443 = Build Array(w608, w607, w606, w605, w604, w603, w596, w595, w594, w593, w592, w591, w589) -> (w561:dbl[][])
                            n444 = local write "Gráfico"(w561) -> ()
                            n445 = local read "Valvulas"() -> (w563:T2)
                            n446 = Build Array (concatenate)(w561, w560, w559, w558, w557) -> (w556:dbl[][])
                            n447 = call "seletor_adq.vi"("Valvulas"=w563, "Matriz entrada"=w556) -> ("matriz saída"=w562:dbl[][])  [unwired: 3 in]
                            n448 = Index Array(array=w618, index (row) #1=0 ("index (row)"), index (row) #2=1 ("index (row)"), index (row) #3=2 ("index (row)"), index (row) #4=3 ("index (row)"), index (row) #5=4 ("index (row)"), index (row) #6=5 ("index (row)"), index (row) #7=6 ("index (row)"), index (row) #8=7 ("index (row)"), index (row) #9=8 ("index (row)"), index (row) #10=9 ("index (row)"), index (row) #11=10 ("index (row)"), index (row) #12=11 ("index (row)"), index (row) #13=12 ("index (row)")) -> (element #1=w647:dbl[], element #2=w632:dbl[], element #3=w631:dbl[], element #4=w630:dbl[], element #5=w629:dbl[], element #6=w628:dbl[], element #7=w627:dbl[], element #8=w626:dbl[], element #9=w625:dbl[], element #10=w624:dbl[], element #11=w623:dbl[], element #12=w622:dbl[], element #13=w621:dbl[])  [unwired: 13 in]
                            n449 = local write "Matriz"(w562) -> ()
                            n450 = call-poly <vilib>:"Mean.vi"("X"=w647) -> ("mean"=w516:dbl)  [unwired: 1 out]
                            n451 = call-poly <vilib>:"Mean.vi"("X"=w632) -> ("mean"=w515:dbl)  [unwired: 1 out]
                            n452 = call-poly <vilib>:"Mean.vi"("X"=w631) -> ("mean"=w514:dbl)  [unwired: 1 out]
                            n453 = call-poly <vilib>:"Mean.vi"("X"=w630) -> ("mean"=w513:dbl)  [unwired: 1 out]
                            n454 = call-poly <vilib>:"Mean.vi"("X"=w629) -> ("mean"=w512:dbl)  [unwired: 1 out]
                            n455 = call-poly <vilib>:"Mean.vi"("X"=w628) -> ("mean"=w511:dbl)  [unwired: 1 out]
                            n456 = call-poly <vilib>:"Mean.vi"("X"=w627) -> ("mean"=w510:dbl)  [unwired: 1 out]
                            n457 = call-poly <vilib>:"Mean.vi"("X"=w626) -> ("mean"=w509:dbl)  [unwired: 1 out]
                            n458 = call-poly <vilib>:"Mean.vi"("X"=w625) -> ("mean"=w508:dbl)  [unwired: 1 out]
                            n459 = call-poly <vilib>:"Mean.vi"("X"=w624) -> ("mean"=w507:dbl)  [unwired: 1 out]
                            n460 = call-poly <vilib>:"Mean.vi"("X"=w623) -> ("mean"=w506:dbl)  [unwired: 1 out]
                            n461 = call-poly <vilib>:"Mean.vi"("X"=w622) -> ("mean"=w505:dbl)  [unwired: 1 out]
                            n462 = call-poly <vilib>:"Mean.vi"("X"=w621) -> ("mean"=w504:dbl)  [unwired: 1 out]
                            n463 = local write "C2-M corrente"(w513) -> ()
                            n464 = local write "C3-M corrente"(w509) -> ()
                            n465 = local write "C4-M corrente"(w506) -> ()
                            n466 = local write "C4-J corrente"(w505) -> ()
                            n467 = local write "P4 corrente"(w504) -> ()
                            n468 = local write "C1-M corrente"(w516) -> ()
                            n469 = local write "C3-J corrente"(w508) -> ()
                            n470 = local write "P3 corrente"(w507) -> ()
                            n471 = local write "C1-J corrente"(w515) -> ()
                            n472 = local write "Pfundo corrente"(w510) -> ()
                            n473 = local write "C2-J corrente"(w512) -> ()
                            n474 = local write "P2 corrente"(w511) -> ()
                            n475 = local write "P1 corrente"(w514) -> ()
                            n476 = property on="Pontos No Gráfico" class="Knob (strict)"("DisabledEnum"=T3."Disabled and Grayed Out" ("Disabled")) -> ()  [unwired: 2 in, 2 out]
                            n477 = Multiply(x=w510, y=0.25) -> (x*y=w497:dbl)
                            n478 = Multiply(x=w511, y=0.25) -> (x*y=w496:dbl)
                            n479 = Multiply(x=w506, y=0.25) -> (x*y=w501:dbl)
                            n480 = Multiply(x=w509, y=0.25) -> (x*y=w498:dbl)
                            n481 = Multiply(x=w508, y=0.25) -> (x*y=w499:dbl)
                            n482 = Multiply(x=w507, y=0.25) -> (x*y=w500:dbl)
                            n483 = Multiply(x=w505, y=0.25) -> (x*y=w502:dbl)
                            n484 = Multiply(x=w504, y=0.25) -> (x*y=w503:dbl)
                            n485 = Multiply(x=w513, y=0.25) -> (x*y=w494:dbl)
                            n486 = Multiply(x=w512, y=0.25) -> (x*y=w495:dbl)
                            n487 = Multiply(x=w515, y=0.25) -> (x*y=w492:dbl)
                            n488 = Multiply(x=w514, y=0.25) -> (x*y=w493:dbl)
                            n489 = Multiply(x=w516, y=0.25) -> (x*y=w491:dbl)
                            n490 = local write "Visualizar"(TRUE ("VIEW")) -> ()
                            n491 = local write "led viewing"(TRUE ("visu led")) -> ()
                            n492 = local write "C1-M"(w491) -> ()
                            n493 = local write "C1-J"(w492) -> ()
                            n494 = local write "P1"(w493) -> ()
                            n495 = local write "C2-M"(w494) -> ()
                            n496 = local write "C2-J"(w495) -> ()
                            n497 = local write "P2"(w496) -> ()
                            n498 = local write "Pfundo"(w497) -> ()
                            n499 = local write "C3-M"(w498) -> ()
                            n500 = local write "C3-J"(w499) -> ()
                            n501 = local write "P3"(w500) -> ()
                            n502 = local write "C4-M"(w501) -> ()
                            n503 = local write "C4-J"(w502) -> ()
                            n504 = local write "P4"(w503) -> ()
                          }
                          frame #1 {
                            n505 = Equal?(x=w708, y=0) -> (x = y?=w706:bool)
                            n506 = case shown="True" w706 {
                              frame False {
                              }
                              frame True {
                                n507 = local read "Matriz"() -> (w709:dbl[][])
                                n508 = local write "Matriz 2"(w709) -> ()
                              }
                            }
                          }
                          frame #2 {
                            n509 = local read "Matriz 2"() -> (w711:dbl[][])
                            n510 = local read "Matriz"() -> (w712:dbl[][])
                            n511 = Build Array (concatenate)(w711, w712) -> (w710:T6)
                            n512 = local write "Matriz 2"(w710) -> ()
                          }
                        }
                        n513 = local read "TempoAquisicao"() -> (w444:dbl)
                        n514 = To Double Precision Float(number=w445) -> (double precision float=w449:dbl)
                        n515 = Multiply(x=3.0 ("y"), y=w444) -> (x*y=w447:dbl)
                        n516 = Subtract(x=w447, y=2.0) -> (x-y=w446:dbl)
                        n517 = Divide(x=w449, y=3.0) -> (x/y=w442:dbl)
                        n518 = Greater Or Equal?(x=w449, y=w446) -> (x >= y?=w443:bool)
                        n519 = Compound Arithmetic op=OR(w443, w454) -> (w453:bool)
                        n520 = local write "Timer"(w442) -> ()
                      }
                    }
                    frame 3 {
                      n521 = while {
                        tunnel: [w735] -> w718
                        tunnel: [w722] -> w717
                        tunnel: w716 -> [w734]
                        tunnel: w715 -> [w721]
                        tunnel: w714 -> [w720]
                        tunnel: w713 -> [w719]
                        i -> [w726]
                        stop <- w736 stop-if-true
                        n522 = flat-sequence {
                          tunnel: w734 -> [w824]
                          tunnel: w721 -> [w763]
                          tunnel: w720 -> [w752]
                          tunnel: w719 -> [w738]
                          tunnel: w725 -> [w983]
                          frame #0 {
                            # "0-C1-M\n1-C1-J\n2-P1\n3-C2-M\n4-C2-J\n5-P2\n6-C3-M\n7-C3-J\n8-P3\n9-C4-M\n10-C4-J\n11-P4\n12-Pfundo\n13-SKM-WF\n14-FIC-COR\n15-AI-COR\n16-VEL"
                            # "aréa de calculo para conversões e analise se os dados encontrados estão dentro de um padrão aceitavel"
                            # "Interpretação dos valores recebidos de outr\nPC e distribuido conforme a necessidade"
                            # "baseado nas configurações de valvulas abertas\né possível saber com qual tipo de configuração \nestá sendo trabalhado"
                            # "informação em Ampere para mA"
                            # "indice \"6\" é o Pfundo"
                            # "leituras lindas da placa são colocadas no gráfico"
                            # "SIW-NC-CV-001 05"
                            # "SIK-CV-001 05 04"
                            # "SIT-CV-001 03"
                            # "ADQ 02"
                            # "SPW-WR-VEL 01"
                            # "SPK-WR-VEL 00"
                            n523 = local write "VALORES UDP"(w824) -> ()
                            n524 = Index Array(array=w824, index #1=0 ("index"), index #2=1 ("index"), index #3=2 ("index"), index #4=3 ("index"), index #5=4 ("index"), index #6=5 ("index")) -> (element #1=w853:string, element #2=w852:string, element #3=w851:string, element #4=w850:string, element #5=w849:string, element #6=w848:string)
                            n525 = local read "P2 corrente"() -> (w897:dbl)
                            n526 = local read "P3 corrente"() -> (w896:dbl)
                            n527 = local read "P1 corrente"() -> (w898:dbl)
                            n528 = local read "P4 corrente"() -> (w895:dbl)
                            n529 = local read "Pfundo corrente"() -> (w893:dbl)
                            n530 = invoke class="VI" method="Ctrl Val.Get"(reference=w738, "Control Name"="VALORES") -> ("Get Control Value Variant"=w748:variant)  [unwired: 2 in, 3 out]
                            n531 = call "CONVERSOR.vi"("String"=w853) -> ("float"=w764:dbl)  [unwired: 6 in, 3 out]
                            n532 = local write "JK(m/s)"(w764) -> ()
                            n533 = call "CONVERSOR.vi"("String"=w852) -> ("float"=w765:dbl)  [unwired: 6 in, 3 out]
                            n534 = local write "JW(m/s)"(w765) -> ()
                            n535 = call "CONVERSOR.vi"("String"=w851) -> ()  [unwired: 6 in, 4 out]
                            n536 = call "CONVERSOR.vi"("String"=w850) -> ("boolean"=w814:bool)  [unwired: 6 in, 3 out]
                            n537 = call "CONVERSOR.vi"("String"=w849) -> ("boolean"=w846:bool)  [unwired: 6 in, 3 out]
                            n538 = local write "SIK-CV-001"(w846) -> ()
                            n539 = call "CONVERSOR.vi"("String"=w848) -> ("boolean"=w845:bool)  [unwired: 6 in, 3 out]
                            n540 = local write "SIW-CV-001"(w845) -> ()
                            n541 = Variant To Data(type=string[] [] ("Array"), Variant=w748) -> (data=w747:string[])  [unwired: 1 in, 1 out]
                            n542 = call "variação_pressao_adq.vi"("P1(mA)"=w898, "P2(mA)"=w897, "P3(mA)"=w896, "P4(mA)"=w895, "PFUNDO(mA)"=w893, "JW(m/s)"=w765, "JK(m/s)"=w764, "Valores"=w763, "SIK-CV-001"=w846, "SIW-CV-001"=w845) -> ("P12/L12"=w815:dbl, "P34/L34"=w817:dbl, "P23/L23"=w816:dbl, "P2(kPa)"=w768:dbl, "VALOR TEORICO"=w899:dbl, "P3(kPa)"=w767:dbl, "P1(kPa)"=w769:dbl, "P4(kPa)"=w766:dbl, "P1-P2G"=w818:bool, "P2-P3R"=w821:bool, "P2-P3G"=w820:bool, "P1-P2R"=w819:bool, "P3-P4G"=w822:bool, "P3-P4R"=w823:bool, "PFUNDO(kPa)"=w750:dbl)  [unwired: 3 in]
                            n543 = Index Array(array=w747, index #1=0 ("index"), index #2=1 ("index")) -> (element #1=w746:string, element #2=w745:string)
                            n544 = call "CONVERSOR.vi"("String"=w746) -> ("float"=w740:dbl)  [unwired: 6 in, 3 out]
                            n545 = call "CONVERSOR.vi"("String"=w745) -> ("float"=w739:dbl)  [unwired: 6 in, 3 out]
                            n546 = local write "P23/L [Pa/m]"(w816) -> ()
                            n547 = local write "P34/L [Pa/m]"(w817) -> ()
                            n548 = local write "P12/L [Pa/m]"(w815) -> ()
                            n549 = local write "P3-P4 RED"(w823) -> ()
                            n550 = local write "P1-P2 VERDE"(w818) -> ()
                            n551 = local write "P1-P2 RED"(w819) -> ()
                            n552 = local write "P2-P3 VERDE"(w820) -> ()
                            n553 = local write "P2-P3 RED"(w821) -> ()
                            n554 = local write "P3-P4 VERDE"(w822) -> ()
                            n555 = local write "Pfundo(kPa)"(w750) -> ()
                            n556 = local write "P1(kPa)"(w769) -> ()
                            n557 = local write "P2(kPa)"(w768) -> ()
                            n558 = local write "P4(kPa)"(w766) -> ()
                            n559 = local write "P3(kPa)"(w767) -> ()
                            n560 = local read "ValoresEnviados"() -> (w751:cluster{"Pfundo[kPa]":dbl})
                            n561 = invoke class="VI" method="Ctrl Val.Set"(reference=w752, "Control Name"="ValoresEnviados", "Value"=w751) -> ()  [unwired: 2 in, 5 out]
                            n562 = Bundle By Name(cluster=w751, "Pfundo[kPa]"=w750) -> (w749:cluster{"Pfundo[kPa]":dbl})
                            n563 = local write "JK(m/s)"(w740) -> ()
                            n564 = local write "JW(m/s)"(w739) -> ()
                            n565 = local write "Linha de Teste"(w814) -> ()
                            n566 = call "check-up_adq.vi"("JK(m/s)"=w764, "JW(m/s)"=w765, "P4(kPa)"=w766, "P3(kPa)"=w767, "P2(kPa)"=w768, "P1(kPa)"=w769) -> ("OK 2 R"=w770:bool, "OK 2 G"=w771:bool, "OK RED"=w772:bool, "OK G"=w773:bool)  [unwired: 2 in]
                            n567 = case shown="False" w814 {
                              tunnel: w899 -> [_ w959]
                              frame False {
                                n568 = local write "Valor Teórico[Pa/m]"(nan) -> ()
                              }
                              frame True {
                                n569 = local write "Valor Teórico[Pa/m]"(w959) -> ()
                              }
                            }
                            n570 = local write "ValoresEnviados"(w749) -> ()
                            n571 = local write "Ok"(w773) -> ()
                            n572 = local write "OK2"(w771) -> ()
                            n573 = local write "Ok R"(w772) -> ()
                            n574 = local write "OK2 R"(w770) -> ()
                            n575 = case shown="True" TRUE {
                              tunnel: [w955 w957] -> w889
                              tunnel: [w940 w956] -> w888
                              tunnel: w765 -> [_ w957]
                              tunnel: w764 -> [_ w956]
                              frame False {
                                n576 = local read "Escala de Calibracao - SKM-FI-WF"() -> (w949:cluster{"Escala Max":dbl, "Escala Min":dbl})
                                n577 = local read "Entrada - SKM-FI-WF [CLP]"() -> (w947:dbl)
                                n578 = local read "SKM-FIC-KF_CORIOLI [kg/s]"() -> (w938:dbl)
                                n579 = local read "SKM-AI-KF_CORIOLI [kg/m³]"() -> (w937:dbl)
                                n580 = local read "Escala de Calibracao - SKM-FI-WF"() -> (w943:cluster{"Escala Max":dbl, "Escala Min":dbl})
                                n581 = Bundle By Name(cluster=w943, "Escala Max"=0.001805556, "Escala Min"=0.0 ("Escala Max")) -> (w944:cluster{"Escala Max":dbl, "Escala Min":dbl})
                                n582 = local write "Escala de Calibracao - SKM-FI-WF"(w944) -> ()
                                n583 = Unbundle By Name(w949) -> ("Escala Max"=w950:dbl, "Escala Min"=w948:dbl)
                                n584 = Divide(x=w938, y=w937) -> (x/y=w939:dbl)
                                n585 = Divide(x=w939, y=0.0005107051557) -> (x/y=w940:dbl)
                                n586 = Subtract(x=w950, y=w948) -> (x-y=w951:dbl)
                                n587 = Divide(x=w951, y=4096.0) -> (x/y=w952:dbl)
                                n588 = Multiply(x=w952, y=w947) -> (x*y=w953:dbl)
                                n589 = Add(x=w953, y=w948) -> (x+y=w954:dbl)
                                n590 = Divide(x=w954, y=0.0005107051557) -> (x/y=w955:dbl)
                              }
                              frame True {
                                # "devido a mudança do sistema para não ler valores do CLP , e sim de outro PC\nesse CASE deve ser mantido como TRUE até ordens de mudanças"
                              }
                            }
                            n591 = local write "SIW-CV-001"(w845) -> ()
                            n592 = local write "SIK-CV-001"(w846) -> ()
                            n593 = Build Array(w845, w846) -> (w892:bool[])
                            n594 = local read "Aplicação"() -> (w759:string)
                            n595 = Boolean Array To Number(Boolean array=w892) -> (number=w754:u32)
                            n596 = Equal?(x=w759, y="Deslocamento_Retirada_por_Baixo") -> (x = y?=w761:bool)
                            n597 = Equal?(x=w759, y="Deslocamento_Retirada_por_Cima") -> (x = y?=w760:bool)
                            n598 = local write "JW(m/s)"(w889) -> ()
                            n599 = local write "JK(m/s)"(w888) -> ()
                            n600 = Build Array(w761, w760) -> (w762:bool[])
                            n601 = Boolean Array To Number(Boolean array=w762) -> (number=w755:u32)
                            n602 = case shown="0, Default" w755 {
                              tunnel: ["No Conf." w927 w932] -> w756
                              tunnel: w754 -> [_ w926 w931]
                              frame 0, Default {
                              }
                              frame 1 {
                                n603 = case shown="0, Default" w926 {
                                tunnel: ["No Conf." "C1" "C2"] -> w927
                                frame 0, Default {
                                }
                                frame 1 {
                                }
                                frame 2 {
                                }
                                }
                              }
                              frame 2 {
                                n604 = case shown="0, Default" w931 {
                                tunnel: ["No Conf." "C3" "C4"] -> w932
                                frame 0, Default {
                                }
                                frame 1 {
                                }
                                frame 2 {
                                }
                                }
                              }
                            }
                            n605 = Index Array(array=w824, index #1=6 ("index"), index #2=7 ("index"), index #3=8 ("index"), index #4=9 ("index")) -> (element #1=w841:string, element #2=w840:string, element #3=w839:string, element #4=w827:string)
                            n606 = call "CONVERSOR.vi"("String"=w841) -> ("float"=w829:dbl)  [unwired: 6 in, 3 out]
                            n607 = call "CONVERSOR.vi"("String"=w840) -> ("float"=w830:dbl)  [unwired: 6 in, 3 out]
                            n608 = call "CONVERSOR.vi"("String"=w839) -> ("float"=w831:dbl)  [unwired: 6 in, 3 out]
                            n609 = call "CONVERSOR.vi"("String"=w827) -> ("float"=w826:dbl)  [unwired: 6 in, 3 out]
                            n610 = for {
                              N: 1000 -> [_]
                              tunnel: [w966] -> w838 mode=indexing
                              tunnel: w754 -> [w967]
                              tunnel: w829 -> [w962]
                              tunnel: w830 -> [w961]
                              tunnel: w831 -> [w960]
                              tunnel: [w965] -> w837 mode=indexing
                              tunnel: [w964] -> w836 mode=indexing
                              tunnel: [w963] -> w835 mode=indexing
                              n611 = case shown="1" w967 {
                                tunnel: [w968 w972 w976] -> w966
                                tunnel: [w968 w971 w975] -> w965
                                tunnel: [w968 w970 w974] -> w964
                                tunnel: [w968 w969 w973] -> w963
                                tunnel: w962 -> [_ w971 w975]
                                tunnel: w961 -> [_ w970 w974]
                                tunnel: w960 -> [_ w969 w973]
                                frame 0, Default {
                                w968 = nan
                                }
                                frame 1 {
                                n612 = local read "JW(m/s)"() -> (w972:dbl)
                                }
                                frame 2 {
                                n613 = local read "JK(m/s)"() -> (w976:dbl)
                                }
                              }
                            }
                            n614 = local write "JG(m/s)"(w826) -> ()
                            n615 = local write "Configuração"(w756) -> ()
                            n616 = local write "SKM-FIC-KF-COR"(w830) -> ()
                            n617 = local write "SKM-AI-KF-COR"(w831) -> ()
                            n618 = local write "SKM-FI-WF"(w829) -> ()
                            n619 = for {
                              tunnel: "data" -> [w978] mode=indexing
                              tunnel: [w977] -> w887 mode=indexing
                              n620 = for {
                                tunnel: w978 -> [w981] mode=indexing
                                tunnel: [w979] -> w977 mode=indexing
                                n621 = Multiply(x=w981, y=1000.0) -> (x*y=w979:dbl)
                              }
                            }
                            n622 = Index Array(array=w887, index (row)=0) -> (element=w918:dbl[])  [unwired: 1 in]
                            n623 = Index Array(array=w887, index (row)=1) -> (element=w924:dbl[])  [unwired: 1 in]
                            n624 = Index Array(array=w887, index (row)=2) -> (element=w923:dbl[])  [unwired: 1 in]
                            n625 = Index Array(array=w887, index (row)=3) -> (element=w922:dbl[])  [unwired: 1 in]
                            n626 = Index Array(array=w887, index (row)=4) -> (element=w921:dbl[])  [unwired: 1 in]
                            n627 = Index Array(array=w887, index (row)=5) -> (element=w920:dbl[])  [unwired: 1 in]
                            n628 = Index Array(array=w887, index (row)=6) -> (element=w919:dbl[])  [unwired: 1 in]
                            n629 = Index Array(array=w887, index (row)=7) -> (element=w917:dbl[])  [unwired: 1 in]
                            n630 = Index Array(array=w887, index (row)=8) -> (element=w916:dbl[])  [unwired: 1 in]
                            n631 = Index Array(array=w887, index (row)=9) -> (element=w915:dbl[])  [unwired: 1 in]
                            n632 = Index Array(array=w887, index (row)=10) -> (element=w914:dbl[])  [unwired: 1 in]
                            n633 = Index Array(array=w887, index (row)=11) -> (element=w913:dbl[])  [unwired: 1 in]
                            n634 = Index Array(array=w887, index (row)=12) -> (element=w912:dbl[])  [unwired: 1 in]
                            n635 = call-poly <vilib>:"Mean.vi"("X"=w918) -> ("mean"=w799:dbl)  [unwired: 1 out]
                            n636 = call-poly <vilib>:"Mean.vi"("X"=w924) -> ("mean"=w798:dbl)  [unwired: 1 out]
                            n637 = call-poly <vilib>:"Mean.vi"("X"=w923) -> ("mean"=w797:dbl)  [unwired: 1 out]
                            n638 = call-poly <vilib>:"Mean.vi"("X"=w922) -> ("mean"=w796:dbl)  [unwired: 1 out]
                            n639 = call-poly <vilib>:"Mean.vi"("X"=w921) -> ("mean"=w795:dbl)  [unwired: 1 out]
                            n640 = call-poly <vilib>:"Mean.vi"("X"=w920) -> ("mean"=w794:dbl)  [unwired: 1 out]
                            n641 = call-poly <vilib>:"Mean.vi"("X"=w919) -> ("mean"=w793:dbl)  [unwired: 1 out]
                            n642 = call-poly <vilib>:"Mean.vi"("X"=w917) -> ("mean"=w792:dbl)  [unwired: 1 out]
                            n643 = call-poly <vilib>:"Mean.vi"("X"=w916) -> ("mean"=w791:dbl)  [unwired: 1 out]
                            n644 = call-poly <vilib>:"Mean.vi"("X"=w915) -> ("mean"=w790:dbl)  [unwired: 1 out]
                            n645 = call-poly <vilib>:"Mean.vi"("X"=w914) -> ("mean"=w789:dbl)  [unwired: 1 out]
                            n646 = call-poly <vilib>:"Mean.vi"("X"=w913) -> ("mean"=w788:dbl)  [unwired: 1 out]
                            n647 = call-poly <vilib>:"Mean.vi"("X"=w912) -> ("mean"=w787:dbl)  [unwired: 1 out]
                            n648 = local write "C1-M corrente"(w799) -> ()
                            n649 = local write "C1-J corrente"(w798) -> ()
                            n650 = local write "C2-M corrente"(w796) -> ()
                            n651 = local write "C3-J corrente"(w791) -> ()
                            n652 = local write "P3 corrente"(w790) -> ()
                            n653 = local write "P2 corrente"(w794) -> ()
                            n654 = local write "Pfundo corrente"(w793) -> ()
                            n655 = local write "C3-M corrente"(w792) -> ()
                            n656 = local write "C4-M corrente"(w789) -> ()
                            n657 = local write "C4-J corrente"(w788) -> ()
                            n658 = local write "P1 corrente"(w797) -> ()
                            n659 = local write "C2-J corrente"(w795) -> ()
                            n660 = local write "P4 corrente"(w787) -> ()
                            n661 = Multiply(x=w793, y=0.25) -> (x*y=w780:dbl)
                            n662 = Multiply(x=w794, y=0.25) -> (x*y=w779:dbl)
                            n663 = Multiply(x=w789, y=0.25) -> (x*y=w784:dbl)
                            n664 = Multiply(x=w792, y=0.25) -> (x*y=w781:dbl)
                            n665 = Multiply(x=w791, y=0.25) -> (x*y=w782:dbl)
                            n666 = Multiply(x=w790, y=0.25) -> (x*y=w783:dbl)
                            n667 = Multiply(x=w788, y=0.25) -> (x*y=w785:dbl)
                            n668 = Multiply(x=w787, y=0.25) -> (x*y=w786:dbl)
                            n669 = Multiply(x=w796, y=0.25) -> (x*y=w777:dbl)
                            n670 = Multiply(x=w795, y=0.25) -> (x*y=w778:dbl)
                            n671 = Multiply(x=w798, y=0.25) -> (x*y=w775:dbl)
                            n672 = Multiply(x=w797, y=0.25) -> (x*y=w776:dbl)
                            n673 = Multiply(x=w799, y=0.25) -> (x*y=w774:dbl)
                            n674 = local write "C1-M"(w774) -> ()
                            n675 = local write "C1-J"(w775) -> ()
                            n676 = local write "P1"(w776) -> ()
                            n677 = local write "C2-M"(w777) -> ()
                            n678 = local write "C2-J"(w778) -> ()
                            n679 = local write "P2"(w779) -> ()
                            n680 = local write "Pfundo"(w780) -> ()
                            n681 = local write "C3-M"(w781) -> ()
                            n682 = local write "C3-J"(w782) -> ()
                            n683 = local write "P3"(w783) -> ()
                            n684 = local write "C4-M"(w784) -> ()
                            n685 = local write "C4-J"(w785) -> ()
                            n686 = local write "P4"(w786) -> ()
                            n687 = Index Array(array=w887, index (row) #1=0 ("index (row)"), index (row) #2=1 ("index (row)"), index (row) #3=2 ("index (row)"), index (row) #4=3 ("index (row)"), index (row) #5=4 ("index (row)"), index (row) #6=5 ("index (row)")) -> (element #1=w879:dbl[], element #2=w878:dbl[], element #3=w877:dbl[], element #4=w876:dbl[], element #5=w875:dbl[], element #6=w874:dbl[])  [unwired: 6 in]
                            n688 = Index Array(array=w887, index (row) #1=7 ("index (row)"), index (row) #2=8 ("index (row)"), index (row) #3=9 ("index (row)"), index (row) #4=10 ("index (row)"), index (row) #5=11 ("index (row)"), index (row) #6=12 ("index (row)")) -> (element #1=w867:dbl[], element #2=w866:dbl[], element #3=w865:dbl[], element #4=w864:dbl[], element #5=w863:dbl[], element #6=w862:dbl[])  [unwired: 6 in]
                            n689 = Index Array(array=w887, index (row)=6) -> (element=w860:dbl[])  [unwired: 1 in]
                            n690 = local read "Valvulas"() -> (w886:T2)
                            n691 = property on="Pontos No Gráfico" class="Knob (strict)"("DisabledEnum"=T3."Disabled and Grayed Out" ("Disabled")) -> ()  [unwired: 2 in, 2 out]
                            n692 = Build Array(w879, w878, w877, w876, w875, w874, w867, w866, w865, w864, w863, w862, w860) -> (w832:dbl[][])
                            n693 = local write "led viewing"(TRUE ("visu led")) -> ()
                            n694 = Build Array (concatenate)(w832, w837, w836, w835, w838) -> (w833:dbl[][])
                            n695 = call "seletor_adq.vi"("Valvulas"=w886, "Matriz entrada"=w833) -> ("matriz saída"=w834:dbl[][])  [unwired: 3 in]
                            n696 = local write "Gráfico"(w832) -> ()
                            n697 = local write "Matriz"(w834) -> ()
                          }
                          frame #1 {
                            n698 = Equal?(x=w983, y=0.0) -> (x = y?=w982:bool)
                            n699 = case shown="True" w982 {
                              frame False {
                              }
                              frame True {
                                n700 = local read "Matriz"() -> (w985:dbl[][])
                                n701 = local write "Matriz 2"(w985) -> ()
                              }
                            }
                          }
                          frame #2 {
                            n702 = local read "Matriz 2"() -> (w988:dbl[][])
                            n703 = local read "Matriz"() -> (w987:dbl[][])
                            n704 = Build Array (concatenate)(w988, w987) -> (w986:T6)
                            n705 = local write "Matriz 2"(w986) -> ()
                          }
                        }
                        n706 = local read "STOP"() -> (w732:bool)
                        n707 = local read "SAIR"() -> (w733:bool)
                        n708 = Or(x=w733, y=w732) -> (x .or. y?=w735:bool)
                        n709 = local read "TempoAquisicao"() -> (w723:dbl)
                        n710 = To Double Precision Float(number=w726) -> (double precision float=w725:dbl)
                        n711 = Multiply(x=3.0 ("y"), y=w723) -> (x*y=w728:dbl)
                        n712 = Subtract(x=w728, y=2.0) -> (x-y=w727:dbl)
                        n713 = Divide(x=w725, y=3.0) -> (x/y=w724:dbl)
                        n714 = local write "Timer"(w724) -> ()
                        n715 = Greater Or Equal?(x=w725, y=w727) -> (x >= y?=w722:bool)
                        n716 = local write "LED adquiri"(TRUE ("adq")) -> ()
                        n717 = Compound Arithmetic op=OR(w722, w735) -> (w736:bool)
                      }
                    }
                  }
                  n718 = local read "STOP"() -> (w185:bool)
                  n719 = local read "SAIR"() -> (w186:bool)
                }
                frame True {
                  w1000 = refnum<k21> "ADQUIRE" ("DAQmx Task Name")
                  w999 = 10123 items=["Finite Samples"=10178, "Continuous Samples"=10123, "Hardware Timed Single Point"=12522] ("sample mode")
                  # "Parte de comunicação com a placa da NATIONAL\nINSTRUMENTS\nno módulo de comunicação chamado DAQmx\nselecionamos o tipo \"continuous SAMPLES\" para a\ncoleta de amostras contínuas\ntambém entramos com o nome de TASK chamado\nADQUIRE, que já contém informações de leitura \njá pré programadas\nFrequência padrão de 3000Hz"
                  n720 = call-poly <vilib>:"DAQmx Timing.vi"("task/channels in"=w1000, "sample mode"=w999, "rate"="Frequência", "source"=tag "OnboardClock") -> ("task out"=w997:refnum<k21>, "error out"=w996:errorcluster)  [unwired: 10 in]
                  n721 = case shown="2" w1004 {
                    tunnel: [w1041 w1171 w1277 w1591] -> w1003
                    tunnel: [w1042 w1170 w1276 w1590] -> w1002
                    tunnel: w1001 -> [w1038 w1124 w1275 w1589]
                    tunnel: w997 -> [w1040 w1114 w1274 w1588]
                    tunnel: w996 -> [w1039 w1113 w1273 w1587]
                    tunnel: [w1040 w1112 w1272 w1586] -> w994
                    tunnel: [w1039 w1111 w1271 w1585] -> w993
                    tunnel: w991 -> [_ w1058 w1270 w1584]
                    tunnel: w990 -> [_ w1045 w1269 w1583]
                    tunnel: w989 -> [_ _ w1268 w1582]
                    frame 0, Default {
                      # "entrada do case através de 2 logicas\ncom apenas \"VISUALIZAR\" apertado, entrará no CASE 1, onde só todos os dados do programa será jogado no gráfico e não tem salvamento\nmas a qualquer instante que for apertado a tecla \"COMEÇAR\" ou algum acionamento por parte de outro PC\no case entrará no case \"2\" ( caso visualizar naõ esteja apertado) ou no caso\"3\" visuzalizar e gravar aquivo em conjunto"
                      n722 = Index Array(array=w1038, index #1=0 ("index"), index #2=1 ("index"), index #3=2 ("index"), index #4=3 ("index"), index #5=4 ("index"), index #6=5 ("index"), index #7=6 ("index"), index #8=7 ("index"), index #9=8 ("index"), index #10=9 ("index"), index #11=10 ("index")) -> (element #1=w1027:string, element #2=w1026:string, element #3=w1025:string, element #4=w1024:string, element #5=w1023:string, element #6=w1022:string, element #7=w1021:string, element #8=w1020:string, element #9=w1019:string, element #10=w1018:string, element #11=w1007:string)
                      n723 = call "CONVERSOR.vi"("String"=w1027) -> ("float"=w1017:dbl)  [unwired: 6 in, 3 out]
                      n724 = call "CONVERSOR.vi"("String"=w1026) -> ("float"=w1016:dbl)  [unwired: 6 in, 3 out]
                      n725 = call "CONVERSOR.vi"("String"=w1025) -> ("boolean"=w1015:bool)  [unwired: 6 in, 3 out]
                      n726 = call "CONVERSOR.vi"("String"=w1024) -> ("boolean"=w1014:bool)  [unwired: 6 in, 3 out]
                      n727 = call "CONVERSOR.vi"("String"=w1023) -> ("boolean"=w1013:bool)  [unwired: 6 in, 3 out]
                      n728 = call "CONVERSOR.vi"("String"=w1022) -> ("boolean"=w1012:bool)  [unwired: 6 in, 3 out]
                      n729 = call "CONVERSOR.vi"("String"=w1021) -> ("float"=w1011:dbl)  [unwired: 6 in, 3 out]
                      n730 = call "CONVERSOR.vi"("String"=w1020) -> ("float"=w1010:dbl)  [unwired: 6 in, 3 out]
                      n731 = call "CONVERSOR.vi"("String"=w1019) -> ("float"=w1009:dbl)  [unwired: 6 in, 3 out]
                      n732 = call "CONVERSOR.vi"("String"=w1018) -> ("float"=w1008:dbl)  [unwired: 6 in, 3 out]
                      n733 = call "CONVERSOR.vi"("String"=w1007) -> ("boolean"=→"SKS-NC-CV-006":bool)  [unwired: 6 in, 3 out]
                      n734 = local write "Aquisição Automática"(w1015) -> ()
                      n735 = local write "SKM-AI-KF-COR"(w1009) -> ()
                      n736 = local write "Linha de Teste"(w1014) -> ()
                      n737 = local write "SKM-FI-WF"(w1011) -> ()
                      n738 = local write "SIK-CV-001"(w1013) -> ()
                      n739 = local write "SIW-CV-001"(w1012) -> ()
                      n740 = local write "SKM-FIC-KF-COR"(w1010) -> ()
                      n741 = local write "JW(m/s)"(w1016) -> ()
                      n742 = local write "JG(m/s)"(w1008) -> ()
                      n743 = local write "JK(m/s)"(w1017) -> ()
                      n744 = local read "STOP"() -> (w1042:bool)
                      n745 = local read "SAIR"() -> (w1041:bool)
                      "VALORES UDP" <- w1038
                    }
                    frame 1 {
                      # "aplicação barbara"
                      # "JG_AR"
                      # "6-SKM-FI-WF"
                      # "7-SKM-FIC-KF-COR"
                      # "8-SKM-AI-KF-COR"
                      # "6-SKM-FI-WF\n7-SKM-FIC-KF_COR\n8-SKM-AI-KF_COR"
                      # "indice \"6\" é o Pfundo"
                      # "leituras lindas da placa são colocadas no gráfico"
                      # "baseado nas configurações de valvulas abertas\né possível saber com qual tipo de configuração \nestá sendo trabalhado"
                      # "aréa de calculo para conversões e analise se os dados encontrados estão dentro de um padrão aceitavel"
                      # "Interpretação dos valores recebidos de outr\nPC e distribuido conforme a necessidade"
                      # "informação em Ampere é transformada em mA"
                      # "Coleta de dados da Placa da NATIONAL com a quantidade de \"numeros de pontos do gráfico\""
                      # "ADQ 02"
                      # "SIW-NC-CV-001 05"
                      # "SIK-CV-001 05 04"
                      # "SIT-CV-001 03"
                      # "SPW-WR-VEL 01"
                      # "SPK-WR-VEL 00"
                      # "Cálculos das médias das pressões e das impedâncias"
                      # "Cálculos"
                      n746 = invoke class="VI" method="Ctrl Val.Set"(reference=w1045, "Control Name"="ValoresEnviados", "Value"="ValoresEnviados") -> ()  [unwired: 2 in, 5 out]
                      n747 = Index Array(array=w1124, index #1=6 ("index"), index #2=7 ("index"), index #3=8 ("index"), index #4=10 ("index")) -> (element #1=w1120:string, element #2=w1119:string, element #3=w1118:string, element #4=w1056:string)
                      n748 = call "CONVERSOR.vi"("String"=w1056) -> ("boolean"=w1055:bool)  [unwired: 6 in, 3 out]
                      n749 = call "CONVERSOR.vi"("String"=w1119) -> ("float"=→"SKM-FIC-KF-COR":dbl)  [unwired: 6 in, 3 out]
                      n750 = call "CONVERSOR.vi"("String"=w1120) -> ("float"=→"SKM-FI-WF":dbl)  [unwired: 6 in, 3 out]
                      n751 = call "CONVERSOR.vi"("String"=w1118) -> ("float"=→"SKM-AI-KF-COR":dbl)  [unwired: 6 in, 3 out]
                      n752 = local write "SKS-NC-CV-006"(w1055) -> ()
                      n753 = Index Array(array=w1124, index #1=4 ("index"), index #2=5 ("index"), index #3=3 ("index"), index #4=2 ("index"), index #5=1 ("index"), index #6=0 ("index"), index #7=9 ("index")) -> (element #1=w1141:string, element #2=w1140:string, element #3=w1137:string, element #4=w1133:string, element #5=w1129:string, element #6=w1126:string, element #7=w1109:string)
                      n754 = local write "VALORES UDP"(w1124) -> ()
                      n755 = call "CONVERSOR.vi"("String"=w1109) -> ("float"=→"JG(m/s)":dbl)  [unwired: 6 in, 3 out]
                      n756 = call "CONVERSOR.vi"("String"=w1141) -> ("boolean"=w1135:bool)  [unwired: 6 in, 3 out]
                      n757 = call "CONVERSOR.vi"("String"=w1133) -> ("boolean"=w1132:bool)  [unwired: 6 in, 3 out]
                      n758 = call "CONVERSOR.vi"("String"=w1140) -> ("boolean"=w1139:bool)  [unwired: 6 in, 3 out]
                      n759 = call "CONVERSOR.vi"("String"=w1137) -> ("boolean"=w1136:bool)  [unwired: 6 in, 3 out]
                      n760 = call "CONVERSOR.vi"("String"=w1129) -> ("float"=w1128:dbl)  [unwired: 6 in, 3 out]
                      n761 = call "CONVERSOR.vi"("String"=w1126) -> ("float"=w1125:dbl)  [unwired: 6 in, 3 out]
                      n762 = local write "SIK-CV-001"(w1135) -> ()
                      n763 = local write "SIW-CV-001"(w1139) -> ()
                      n764 = case shown="True" TRUE {
                        tunnel: [w1239 w1258] -> w1201
                        tunnel: [w1238 w1259] -> w1200
                        tunnel: w1128 -> [_ w1259]
                        tunnel: w1125 -> [_ w1258]
                        frame False {
                          # "Cálculos de valores de velocidade utilizando informações do CLP"
                          # "área"
                          # "área"
                          n765 = local read "Escala de Calibracao - SKM-FI-WF"() -> (w1245:cluster{"Escala Max":dbl, "Escala Min":dbl})
                          n766 = Unbundle By Name("Escala de Calibracao - SKM-FI-WF") -> ("Escala Max"=w1248:dbl, "Escala Min"=w1247:dbl)
                          n767 = Bundle By Name(cluster=w1245, "Escala Max"=0.001805556, "Escala Min"=0.0 ("Escala Max")) -> (w1246:cluster{"Escala Max":dbl, "Escala Min":dbl})
                          n768 = Divide(x="SKM-FIC-KF_CORIOLI [kg/s]", y="SKM-AI-KF_CORIOLI [kg/m³]") -> (x/y=w1257:dbl)
                          n769 = Divide(x=w1257, y=0.0005107051557) -> (x/y=w1239:dbl)
                          n770 = local write "Escala de Calibracao - SKM-FI-WF"(w1246) -> ()
                          n771 = Subtract(x=w1248, y=w1247) -> (x-y=w1249:dbl)
                          n772 = Divide(x=w1249, y=4096.0) -> (x/y=w1250:dbl)
                          n773 = Multiply(x=w1250, y="Entrada - SKM-FI-WF [CLP]") -> (x*y=w1251:dbl)
                          n774 = Add(x=w1251, y=w1247) -> (x+y=w1254:dbl)
                          n775 = Divide(x=w1254, y=0.0005107051557) -> (x/y=w1238:dbl)
                        }
                        frame True {
                          # "devido a mudança do sistema para não ler valores do CLP , e sim de outro PC\nesse CASE deve ser mantido como TRUE até ordens de mudanças"
                        }
                      }
                      n776 = local read "Pfundo corrente"() -> (w1205:dbl)
                      n777 = local read "P1 corrente"() -> (w1219:dbl)
                      n778 = local read "P2 corrente"() -> (w1218:dbl)
                      n779 = local read "P3 corrente"() -> (w1217:dbl)
                      n780 = local read "P4 corrente"() -> (w1209:dbl)
                      n781 = local read "JW(m/s)"() -> (w1060:dbl)
                      n782 = local read "JK(m/s)"() -> (w1059:dbl)
                      n783 = call "variação_pressao_adq.vi"("P1(mA)"=w1219, "P2(mA)"=w1218, "P3(mA)"=w1217, "P4(mA)"=w1209, "PFUNDO(mA)"=w1205, "JW(m/s)"=w1060, "JK(m/s)"=w1059, "Valores"=w1058, "SIK-CV-001"=w1135, "SIW-CV-001"=w1139) -> ("P12/L12"=w1210:dbl, "P34/L34"=w1212:dbl, "P23/L23"=w1211:dbl, "P2(kPa)"=w1063:dbl, "VALOR TEORICO"=w1213:dbl, "P3(kPa)"=w1062:dbl, "P1(kPa)"=w1064:dbl, "P4(kPa)"=w1061:dbl, "P1-P2G"=w1216:bool, "P2-P3R"=w1206:bool, "P2-P3G"=w1215:bool, "P1-P2R"=w1208:bool, "P3-P4G"=w1214:bool, "P3-P4R"=w1207:bool, "PFUNDO(kPa)"=w1046:dbl)  [unwired: 3 in]
                      n784 = Bundle By Name(cluster="ValoresEnviados", "Pfundo[kPa]"=w1046) -> (w1047:cluster{"Pfundo[kPa]":dbl})
                      n785 = local write "ValoresEnviados"(w1047) -> ()
                      n786 = local write "P1-P2 VERDE"(w1216) -> ()
                      n787 = local write "P1-P2 RED"(w1208) -> ()
                      n788 = local write "P2-P3 VERDE"(w1215) -> ()
                      n789 = local write "P2-P3 RED"(w1206) -> ()
                      n790 = local write "P3-P4 VERDE"(w1214) -> ()
                      n791 = local write "P3-P4 RED"(w1207) -> ()
                      n792 = local write "Pfundo(kPa)"(w1046) -> ()
                      n793 = local write "P12/L [Pa/m]"(w1210) -> ()
                      n794 = local write "P23/L [Pa/m]"(w1211) -> ()
                      n795 = local write "P34/L [Pa/m]"(w1212) -> ()
                      n796 = local write "P1(kPa)"(w1064) -> ()
                      n797 = local write "P2(kPa)"(w1063) -> ()
                      n798 = local write "P3(kPa)"(w1062) -> ()
                      n799 = local write "P4(kPa)"(w1061) -> ()
                      n800 = call "check-up_adq.vi"("JK(m/s)"=w1059, "JW(m/s)"=w1060, "P4(kPa)"=w1061, "P3(kPa)"=w1062, "P2(kPa)"=w1063, "P1(kPa)"=w1064) -> ("OK 2 R"=w1065:bool, "OK 2 G"=w1066:bool, "OK RED"=w1067:bool, "OK G"=w1068:bool)  [unwired: 2 in]
                      n801 = local write "OK2 R"(w1065) -> ()
                      n802 = local write "Ok"(w1068) -> ()
                      n803 = local write "Ok R"(w1067) -> ()
                      n804 = local write "OK2"(w1066) -> ()
                      n805 = call <vilib>:"DAQmx Start Task.vi"("task/channels in"=w1114, "error in"=w1113) -> ("task out"=w1226:refnum<k21>, "error out"=w1225:errorcluster)  [unwired: 12 in]
                      n806 = local write "JW(m/s)"(w1200) -> ()
                      n807 = local write "JK(m/s)"(w1201) -> ()
                      n808 = local write "Linha de Teste"(w1136) -> ()
                      n809 = call-poly <vilib>:"DAQmx Read.vi"("task/channels in"=w1226, "number of samples per channel"="Pontos No Gráfico", "error in"=w1225) -> ("task out"=w1224:refnum<k21>, "data"=w1222:dbl[][], "error out"=w1223:errorcluster)  [unwired: 10 in]
                      n810 = case shown="True" w1136 {
                        tunnel: w1213 -> [_ w1262]
                        frame False {
                          n811 = local write "Valor Teórico[Pa/m]"(nan) -> ()
                        }
                        frame True {
                          n812 = local write "Valor Teórico[Pa/m]"(w1262) -> ()
                        }
                      }
                      n813 = call <vilib>:"DAQmx Stop Task.vi"("task/channels in"=w1224, "error in"=w1223) -> ("task out"=w1112:refnum<k21>, "error out"=w1111:errorcluster)  [unwired: 12 in]
                      n814 = for {
                        tunnel: w1222 -> [w1263] mode=indexing
                        tunnel: [w1264] -> w1173 mode=indexing
                        n815 = for {
                          tunnel: w1263 -> [w1267] mode=indexing
                          tunnel: [w1265] -> w1264 mode=indexing
                          n816 = Multiply(x=w1267, y=1000.0) -> (x*y=w1265:dbl)
                        }
                      }
                      n817 = local write "SIW-CV-001"(w1139) -> ()
                      n818 = local write "SIK-CV-001"(w1135) -> ()
                      n819 = local read "Aplicação"() -> (w1054:string)
                      n820 = Build Array(w1139, w1135) -> (w1202:bool[])
                      n821 = Boolean Array To Number(Boolean array=w1202) -> (number=w1204:u32)
                      n822 = local write "Aquisição Automática"(w1132) -> ()
                      n823 = Equal?(x=w1054, y="Deslocamento_Retirada_por_Baixo") -> (x = y?=w1050:bool)
                      n824 = Equal?(x=w1054, y="Deslocamento_Retirada_por_Cima") -> (x = y?=w1049:bool)
                      n825 = Build Array(w1050, w1049) -> (w1051:bool[])
                      n826 = Boolean Array To Number(Boolean array=w1051) -> (number=w1048:u32)
                      n827 = case shown="0, Default" w1048 {
                        tunnel: w1204 -> [_ w1228 w1234]
                        tunnel: ["No Conf." w1229 w1233] -> w1203
                        frame 0, Default {
                        }
                        frame 1 {
                          n828 = case shown="0, Default" w1228 {
                            tunnel: ["No Conf." "C1" "C2"] -> w1229
                            frame 0, Default {
                            }
                            frame 1 {
                            }
                            frame 2 {
                            }
                          }
                        }
                        frame 2 {
                          n829 = case shown="0, Default" w1234 {
                            tunnel: ["No Conf." "C3" "C4"] -> w1233
                            frame 0, Default {
                            }
                            frame 1 {
                            }
                            frame 2 {
                            }
                          }
                        }
                      }
                      "Configuração" <- w1203
                      n830 = case shown="True" w1132 {
                        frame False {
                        }
                        frame True {
                          # "Caso a válvula de aquisição\nseja acionada, a visualização \ndeve encerrar, para começar\na gravaçaao"
                          n831 = local write "Pontos No Gráfico"(10.0 ("POINTS IN GRAPH")) -> ()
                        }
                      }
                      n832 = Index Array(array=w1173, index (row) #1=0 ("index (row)"), index (row) #2=1 ("index (row)"), index (row) #3=2 ("index (row)"), index (row) #4=3 ("index (row)"), index (row) #5=4 ("index (row)"), index (row) #6=5 ("index (row)")) -> (element #1=w1163:dbl[], element #2=w1162:dbl[], element #3=w1161:dbl[], element #4=w1160:dbl[], element #5=w1159:dbl[], element #6=w1158:dbl[])  [unwired: 6 in]
                      n833 = Index Array(array=w1173, index (row) #1=7 ("index (row)"), index (row) #2=8 ("index (row)"), index (row) #3=9 ("index (row)"), index (row) #4=10 ("index (row)"), index (row) #5=11 ("index (row)"), index (row) #6=12 ("index (row)")) -> (element #1=w1151:dbl[], element #2=w1150:dbl[], element #3=w1149:dbl[], element #4=w1148:dbl[], element #5=w1147:dbl[], element #6=w1146:dbl[])  [unwired: 6 in]
                      n834 = Index Array(array=w1173, index (row)=6) -> (element=w1144:dbl[])  [unwired: 1 in]
                      n835 = Build Array(w1163, w1162, w1161, w1160, w1159, w1158, w1151, w1150, w1149, w1148, w1147, w1146, w1144) -> (→"Gráfico":dbl[][])
                      n836 = local read "SAIR"() -> (w1170:bool)
                      n837 = local read "STOP"() -> (w1171:bool)
                      n838 = Index Array(array=w1173, index (row) #1=0 ("index (row)"), index (row) #2=1 ("index (row)"), index (row) #3=2 ("index (row)"), index (row) #4=3 ("index (row)"), index (row) #5=4 ("index (row)"), index (row) #6=5 ("index (row)"), index (row) #7=6 ("index (row)"), index (row) #8=7 ("index (row)"), index (row) #9=8 ("index (row)"), index (row) #10=9 ("index (row)"), index (row) #11=10 ("index (row)"), index (row) #12=11 ("index (row)"), index (row) #13=12 ("index (row)")) -> (element #1=w1221:dbl[], element #2=w1197:dbl[], element #3=w1185:dbl[], element #4=w1184:dbl[], element #5=w1183:dbl[], element #6=w1182:dbl[], element #7=w1181:dbl[], element #8=w1180:dbl[], element #9=w1179:dbl[], element #10=w1178:dbl[], element #11=w1177:dbl[], element #12=w1176:dbl[], element #13=w1175:dbl[])  [unwired: 13 in]
                      n839 = call-poly <vilib>:"Mean.vi"("X"=w1221) -> ("mean"=w1069:dbl)  [unwired: 1 out]
                      n840 = call-poly <vilib>:"Mean.vi"("X"=w1197) -> ("mean"=w1070:dbl)  [unwired: 1 out]
                      n841 = call-poly <vilib>:"Mean.vi"("X"=w1185) -> ("mean"=w1071:dbl)  [unwired: 1 out]
                      n842 = call-poly <vilib>:"Mean.vi"("X"=w1184) -> ("mean"=w1072:dbl)  [unwired: 1 out]
                      n843 = call-poly <vilib>:"Mean.vi"("X"=w1183) -> ("mean"=w1073:dbl)  [unwired: 1 out]
                      n844 = call-poly <vilib>:"Mean.vi"("X"=w1182) -> ("mean"=w1074:dbl)  [unwired: 1 out]
                      n845 = call-poly <vilib>:"Mean.vi"("X"=w1181) -> ("mean"=w1075:dbl)  [unwired: 1 out]
                      n846 = call-poly <vilib>:"Mean.vi"("X"=w1180) -> ("mean"=w1076:dbl)  [unwired: 1 out]
                      n847 = call-poly <vilib>:"Mean.vi"("X"=w1179) -> ("mean"=w1077:dbl)  [unwired: 1 out]
                      n848 = call-poly <vilib>:"Mean.vi"("X"=w1178) -> ("mean"=w1078:dbl)  [unwired: 1 out]
                      n849 = call-poly <vilib>:"Mean.vi"("X"=w1177) -> ("mean"=w1079:dbl)  [unwired: 1 out]
                      n850 = call-poly <vilib>:"Mean.vi"("X"=w1176) -> ("mean"=w1080:dbl)  [unwired: 1 out]
                      n851 = call-poly <vilib>:"Mean.vi"("X"=w1175) -> ("mean"=w1081:dbl)  [unwired: 1 out]
                      n852 = local write "C2-M corrente"(w1072) -> ()
                      n853 = local write "C1-M corrente"(w1069) -> ()
                      n854 = local write "C1-J corrente"(w1070) -> ()
                      n855 = local write "P1 corrente"(w1071) -> ()
                      n856 = local write "C2-J corrente"(w1073) -> ()
                      n857 = local write "P2 corrente"(w1074) -> ()
                      n858 = local write "Pfundo corrente"(w1075) -> ()
                      n859 = local write "C3-M corrente"(w1076) -> ()
                      n860 = local write "C3-J corrente"(w1077) -> ()
                      n861 = local write "P3 corrente"(w1078) -> ()
                      n862 = local write "C4-M corrente"(w1079) -> ()
                      n863 = local write "C4-J corrente"(w1080) -> ()
                      n864 = local write "P4 corrente"(w1081) -> ()
                      n865 = Multiply(x=w1075, y=0.25) -> (x*y=w1088:dbl)
                      n866 = Multiply(x=w1074, y=0.25) -> (x*y=w1089:dbl)
                      n867 = Multiply(x=w1079, y=0.25) -> (x*y=w1084:dbl)
                      n868 = Multiply(x=w1076, y=0.25) -> (x*y=w1087:dbl)
                      n869 = Multiply(x=w1077, y=0.25) -> (x*y=w1086:dbl)
                      n870 = Multiply(x=w1078, y=0.25) -> (x*y=w1085:dbl)
                      n871 = Multiply(x=w1080, y=0.25) -> (x*y=w1083:dbl)
                      n872 = Multiply(x=w1081, y=0.25) -> (x*y=w1082:dbl)
                      n873 = Multiply(x=w1072, y=0.25) -> (x*y=w1091:dbl)
                      n874 = Multiply(x=w1073, y=0.25) -> (x*y=w1090:dbl)
                      n875 = Multiply(x=w1070, y=0.25) -> (x*y=w1093:dbl)
                      n876 = Multiply(x=w1071, y=0.25) -> (x*y=w1092:dbl)
                      n877 = Multiply(x=w1069, y=0.25) -> (x*y=w1094:dbl)
                      n878 = local write "C1-M"(w1094) -> ()
                      n879 = local write "C1-J"(w1093) -> ()
                      n880 = local write "P1"(w1092) -> ()
                      n881 = local write "C2-M"(w1091) -> ()
                      n882 = local write "C2-J"(w1090) -> ()
                      n883 = local write "P2"(w1089) -> ()
                      n884 = local write "Pfundo"(w1088) -> ()
                      n885 = local write "C3-M"(w1087) -> ()
                      n886 = local write "C3-J"(w1086) -> ()
                      n887 = local write "P3"(w1085) -> ()
                      n888 = local write "C4-M"(w1084) -> ()
                      n889 = local write "C4-J"(w1083) -> ()
                      n890 = local write "P4"(w1082) -> ()
                      "led viewing" <- TRUE ("visu led")
                    }
                    frame 2 {
                      n891 = while {
                        tunnel: [w1289] -> w1277
                        shift-right: [w1294] -> w1272
                        shift-left: w1274 -> [w1296]
                        shift-right: [w1295] -> w1271
                        shift-left: w1273 -> [w1297]
                        tunnel: [w1287] -> w1276
                        tunnel: w1275 -> [w1286]
                        tunnel: w1270 -> [w1280]
                        tunnel: w1269 -> [w1279]
                        tunnel: w1268 -> [w1278]
                        i -> [w1285]
                        stop <- w1288 stop-if-true
                        n892 = flat-sequence {
                          tunnel: w1297 -> [w1509]
                          tunnel: w1296 -> [w1508]
                          tunnel: [w1457] -> w1289
                          tunnel: [w1507] -> w1293
                          tunnel: [w1506] -> w1292
                          tunnel: w1286 -> [w1344]
                          tunnel: w1280 -> [w1345]
                          tunnel: w1279 -> [w1330]
                          tunnel: w1278 -> [w1314]
                          tunnel: w1293 -> [w1575]
                          tunnel: w1292 -> [w1574]
                          tunnel: [w1575] -> w1291
                          tunnel: [w1574] -> w1290
                          tunnel: w1282 -> [w1573]
                          tunnel: w1291 -> [w1581]
                          tunnel: w1290 -> [w1580]
                          tunnel: [w1581] -> w1295
                          tunnel: [w1580] -> w1294
                          frame #0 {
                            # "Interpretação dos valores recebidos de outr\nPC e distribuido conforme a necessidade"
                            # "aréa de calculo para conversões e analise se os dados encontrados estão dentro de um padrão aceitavel"
                            # "baseado nas configurações de valvulas abertas\né possível saber com qual tipo de configuração \nestá sendo trabalhado"
                            # "informação em Ampere é transformada em mA"
                            # "indice \"6\" é o Pfundo"
                            # "Coleta de dados da Placa da NATIONAL"
                            # "leituras lindas da placa são colocadas no gráfico"
                            # "SIW-NC-CV-001 05"
                            # "SIK-CV-001 05 04"
                            # "SIT-CV-001 03"
                            # "ADQ 02"
                            # "JW 01"
                            # "JK 00"
                            n893 = local read "JW(m/s)"() -> (w1347:dbl)
                            n894 = local read "JK(m/s)"() -> (w1346:dbl)
                            n895 = local read "Pfundo corrente"() -> (w1489:dbl)
                            n896 = local read "P1 corrente"() -> (w1503:dbl)
                            n897 = local read "P2 corrente"() -> (w1502:dbl)
                            n898 = local read "P3 corrente"() -> (w1501:dbl)
                            n899 = local read "P4 corrente"() -> (w1500:dbl)
                            n900 = local write "VALORES UDP"(w1344) -> ()
                            n901 = Index Array(array=w1344, index #1=0 ("index"), index #2=1 ("index"), index #3=2 ("index"), index #4=3 ("index"), index #5=4 ("index"), index #6=5 ("index")) -> (element #1=w1422:string, element #2=w1421:string, element #3=w1420:string, element #4=w1419:string, element #5=w1418:string, element #6=w1417:string)
                            n902 = call "CONVERSOR.vi"("String"=w1421) -> ("float"=w1414:dbl)  [unwired: 6 in, 3 out]
                            n903 = call "CONVERSOR.vi"("String"=w1420) -> ()  [unwired: 6 in, 4 out]
                            n904 = call "CONVERSOR.vi"("String"=w1418) -> ("boolean"=w1412:bool)  [unwired: 6 in, 3 out]
                            n905 = call "CONVERSOR.vi"("String"=w1417) -> ("boolean"=w1411:bool)  [unwired: 6 in, 3 out]
                            n906 = call "variação_pressao_adq.vi"("P1(mA)"=w1503, "P2(mA)"=w1502, "P3(mA)"=w1501, "P4(mA)"=w1500, "PFUNDO(mA)"=w1489, "JW(m/s)"=w1347, "JK(m/s)"=w1346, "Valores"=w1345, "SIK-CV-001"=w1412, "SIW-CV-001"=w1411) -> ("P12/L12"=w1497:dbl, "P34/L34"=w1499:dbl, "P23/L23"=w1498:dbl, "P2(kPa)"=w1350:dbl, "VALOR TEORICO"=w1496:dbl, "P3(kPa)"=w1349:dbl, "P1(kPa)"=w1351:dbl, "P4(kPa)"=w1348:dbl, "P1-P2G"=w1495:bool, "P2-P3R"=w1491:bool, "P2-P3G"=w1494:bool, "P1-P2R"=w1492:bool, "P3-P4G"=w1493:bool, "P3-P4R"=w1490:bool, "PFUNDO(kPa)"=w1328:dbl)  [unwired: 3 in]
                            n907 = local write "P12/L [Pa/m]"(w1497) -> ()
                            n908 = local write "P23/L [Pa/m]"(w1498) -> ()
                            n909 = local write "P34/L [Pa/m]"(w1499) -> ()
                            n910 = local write "P1-P2 VERDE"(w1495) -> ()
                            n911 = local write "P1-P2 RED"(w1492) -> ()
                            n912 = local write "P2-P3 VERDE"(w1494) -> ()
                            n913 = local write "P2-P3 RED"(w1491) -> ()
                            n914 = local write "P3-P4 VERDE"(w1493) -> ()
                            n915 = local write "P3-P4 RED"(w1490) -> ()
                            n916 = call "CONVERSOR.vi"("String"=w1422) -> ("float"=w1415:dbl)  [unwired: 6 in, 3 out]
                            n917 = call "CONVERSOR.vi"("String"=w1419) -> ("boolean"=w1413:bool)  [unwired: 6 in, 3 out]
                            n918 = local write "Linha de Teste"(w1413) -> ()
                            n919 = case shown="False" w1413 {
                              tunnel: w1496 -> [_ w1548]
                              frame False {
                                n920 = local write "Valor Teórico[Pa/m]"(nan) -> ()
                              }
                              frame True {
                                n921 = local write "Valor Teórico[Pa/m]"(w1548) -> ()
                              }
                            }
                            n922 = invoke class="VI" method="Ctrl Val.Get"(reference=w1314, "Control Name"="VALORES") -> ("Get Control Value Variant"=w1320:variant)  [unwired: 2 in, 3 out]
                            n923 = local write "SIK-CV-001"(w1412) -> ()
                            n924 = local write "SIW-CV-001"(w1411) -> ()
                            n925 = call "check-up_adq.vi"("JK(m/s)"=w1346, "JW(m/s)"=w1347, "P4(kPa)"=w1348, "P3(kPa)"=w1349, "P2(kPa)"=w1350, "P1(kPa)"=w1351) -> ("OK 2 R"=w1352:bool, "OK 2 G"=w1353:bool, "OK RED"=w1354:bool, "OK G"=w1355:bool)  [unwired: 2 in]
                            n926 = local write "P2(kPa)"(w1350) -> ()
                            n927 = local write "P3(kPa)"(w1349) -> ()
                            n928 = local write "P1(kPa)"(w1351) -> ()
                            n929 = local write "P4(kPa)"(w1348) -> ()
                            n930 = local write "Pfundo(kPa)"(w1328) -> ()
                            n931 = local write "OK2 R"(w1352) -> ()
                            n932 = local write "Ok R"(w1354) -> ()
                            n933 = local write "OK2"(w1353) -> ()
                            n934 = local write "Ok"(w1355) -> ()
                            n935 = Variant To Data(type=string[] [] ("Array"), Variant=w1320) -> (data=w1321:string[])  [unwired: 1 in, 1 out]
                            n936 = Index Array(array=w1321, index=1) -> (element=w1322:string)
                            n937 = case shown="True" TRUE {
                              tunnel: [w1544 w1546] -> w1486
                              tunnel: [w1537 w1545] -> w1485
                              tunnel: w1415 -> [_ w1546]
                              tunnel: w1414 -> [_ w1545]
                              frame False {
                                n938 = local read "Escala de Calibracao - SKM-FI-WF"() -> (w1533:cluster{"Escala Max":dbl, "Escala Min":dbl})
                                n939 = local read "Entrada - SKM-FI-WF [CLP]"() -> (w1531:dbl)
                                n940 = local read "Escala de Calibracao - SKM-FI-WF"() -> (w1538:cluster{"Escala Max":dbl, "Escala Min":dbl})
                                n941 = Bundle By Name(cluster=w1538, "Escala Max"=0.001805556, "Escala Min"=0.0 ("Escala Max")) -> (w1539:cluster{"Escala Max":dbl, "Escala Min":dbl})
                                n942 = local write "Escala de Calibracao - SKM-FI-WF"(w1539) -> ()
                                n943 = Unbundle By Name(w1533) -> ("Escala Max"=w1527:dbl, "Escala Min"=w1532:dbl)
                                n944 = local read "SKM-AI-KF_CORIOLI [kg/m³]"() -> (w1541:dbl)
                                n945 = local read "SKM-FIC-KF_CORIOLI [kg/s]"() -> (w1542:dbl)
                                n946 = Subtract(x=w1527, y=w1532) -> (x-y=w1525:dbl)
                                n947 = Divide(x=w1525, y=4096.0) -> (x/y=w1534:dbl)
                                n948 = Multiply(x=w1534, y=w1531) -> (x*y=w1535:dbl)
                                n949 = Add(x=w1535, y=w1532) -> (x+y=w1536:dbl)
                                n950 = Divide(x=w1542, y=w1541) -> (x/y=w1543:dbl)
                                n951 = Divide(x=w1536, y=0.0005107051557) -> (x/y=w1537:dbl)
                                n952 = Divide(x=w1543, y=0.0005107051557) -> (x/y=w1544:dbl)
                              }
                              frame True {
                                # "devido a mudança do sistema para não ler valores do CLP , e sim de outro PC\nesse CASE deve ser mantido como TRUE até ordens de mudanças"
                              }
                            }
                            "JK(m/s)" <- w1486
                            "JW(m/s)" <- w1485
                            n953 = call "CONVERSOR.vi"("String"=w1322) -> ("float"=w1315:dbl)  [unwired: 6 in, 3 out]
                            n954 = local write "JW(m/s)"(w1315) -> ()
                            n955 = call-poly <vilib>:"DAQmx Read.vi"("task/channels in"=w1508, "number of samples per channel"=3000, "timeout"=10.0, "error in"=w1509) -> ("task out"=w1506:refnum<k21>, "data"=w1513:dbl[][], "error out"=w1507:errorcluster)  [unwired: 9 in]
                            n956 = local read "ValoresEnviados"() -> (w1327:cluster{"Pfundo[kPa]":dbl})
                            n957 = invoke class="VI" method="Ctrl Val.Set"(reference=w1330, "Control Name"="ValoresEnviados", "Value"=w1327) -> ()  [unwired: 2 in, 5 out]
                            n958 = Bundle By Name(cluster=w1327, "Pfundo[kPa]"=w1328) -> (w1331:cluster{"Pfundo[kPa]":dbl})
                            n959 = Index Array(array=w1344, index=10) -> (element=w1342:string)
                            n960 = call "CONVERSOR.vi"("String"=w1342) -> ("boolean"=w1341:bool)  [unwired: 6 in, 3 out]
                            n961 = local write "ValoresEnviados"(w1331) -> ()
                            n962 = local write "SKS-NC-CV-006"(w1341) -> ()
                            n963 = local read "Aplicação"() -> (w1334:string)
                            n964 = Index Array(array=w1344, index #1=6 ("index"), index #2=7 ("index"), index #3=8 ("index"), index #4=9 ("index")) -> (element #1=w1407:string, element #2=w1406:string, element #3=w1405:string, element #4=w1396:string)
                            n965 = local write "SIW-CV-001"(w1411) -> ()
                            n966 = local write "SIK-CV-001"(w1412) -> ()
                            n967 = call "CONVERSOR.vi"("String"=w1396) -> ("float"=w1395:dbl)  [unwired: 6 in, 3 out]
                            n968 = Build Array(w1411, w1412) -> (w1488:bool[])
                            n969 = local write "JG(m/s)"(w1395) -> ()
                            n970 = call "CONVERSOR.vi"("String"=w1406) -> ("float"=w1325:dbl)  [unwired: 6 in, 3 out]
                            n971 = call "CONVERSOR.vi"("String"=w1405) -> ("float"=w1398:dbl)  [unwired: 6 in, 3 out]
                            n972 = call "CONVERSOR.vi"("String"=w1407) -> ("float"=w1326:dbl)  [unwired: 6 in, 3 out]
                            n973 = Equal?(x=w1334, y="Deslocamento_Retirada_por_Cima") -> (x = y?=w1336:bool)
                            n974 = for {
                              tunnel: w1513 -> [w1567] mode=indexing
                              tunnel: [w1566] -> w1458 mode=indexing
                              n975 = for {
                                tunnel: w1567 -> [w1570] mode=indexing
                                tunnel: [w1568] -> w1566 mode=indexing
                                n976 = Multiply(x=w1570, y=1000.0) -> (x*y=w1568:dbl)
                              }
                            }
                            n977 = Equal?(x=w1334, y="Deslocamento_Retirada_por_Baixo") -> (x = y?=w1337:bool)
                            n978 = Build Array(w1337, w1336) -> (w1338:bool[])
                            n979 = Boolean Array To Number(Boolean array=w1488) -> (number=w1332:u32)
                            n980 = for {
                              N: 3000 -> [_]
                              tunnel: w1332 -> [w1556]
                              tunnel: w1398 -> [w1554]
                              tunnel: [w1555] -> w1401 mode=indexing
                              tunnel: w1326 -> [w1553]
                              tunnel: w1325 -> [w1552]
                              tunnel: [w1551] -> w1324 mode=indexing
                              tunnel: [w1550] -> w1323 mode=indexing
                              tunnel: [w1549] -> w1316 mode=indexing
                              # "SKM-FI-WF"
                              # "SKM-FIC-KF_COR"
                              # "SKM-AI-KF_COR"
                              n981 = case shown="2" w1556 {
                                tunnel: [w1557 w1561 w1565] -> w1555
                                tunnel: [w1557 w1560 w1564] -> w1550
                                tunnel: [w1557 w1559 w1563] -> w1551
                                tunnel: w1554 -> [_ w1561 w1565]
                                tunnel: w1552 -> [_ w1560 w1564]
                                tunnel: w1553 -> [_ w1559 w1563]
                                tunnel: [w1557 w1558 w1562] -> w1549
                                frame 0, Default {
                                w1557 = nan
                                }
                                frame 1 {
                                n982 = local read "JW(m/s)"() -> (w1558:dbl)
                                }
                                frame 2 {
                                n983 = local read "JK(m/s)"() -> (w1562:dbl)
                                }
                              }
                            }
                            n984 = Boolean Array To Number(Boolean array=w1338) -> (number=w1333:u32)
                            n985 = local write "SKM-FIC-KF-COR"(w1398) -> ()
                            n986 = local write "SKM-AI-KF-COR"(w1325) -> ()
                            n987 = local write "SKM-FI-WF"(w1326) -> ()
                            n988 = case shown="0, Default" w1333 {
                              tunnel: ["No Conf." w1516 w1521] -> w1335
                              tunnel: w1332 -> [_ w1515 w1520]
                              frame 0, Default {
                              }
                              frame 1 {
                                n989 = case shown="0, Default" w1515 {
                                tunnel: ["No Conf." "C1" "C2"] -> w1516
                                frame 0, Default {
                                }
                                frame 1 {
                                }
                                frame 2 {
                                }
                                }
                              }
                              frame 2 {
                                n990 = case shown="0, Default" w1520 {
                                tunnel: ["No Conf." "C3" "C4"] -> w1521
                                frame 0, Default {
                                }
                                frame 1 {
                                }
                                frame 2 {
                                }
                                }
                              }
                            }
                            n991 = Index Array(array=w1458, index (row) #1=0 ("index (row)"), index (row) #2=1 ("index (row)"), index (row) #3=2 ("index (row)"), index (row) #4=3 ("index (row)"), index (row) #5=4 ("index (row)"), index (row) #6=5 ("index (row)")) -> (element #1=w1448:dbl[], element #2=w1447:dbl[], element #3=w1446:dbl[], element #4=w1445:dbl[], element #5=w1444:dbl[], element #6=w1443:dbl[])  [unwired: 6 in]
                            n992 = Index Array(array=w1458, index (row) #1=7 ("index (row)"), index (row) #2=8 ("index (row)"), index (row) #3=9 ("index (row)"), index (row) #4=10 ("index (row)"), index (row) #5=11 ("index (row)"), index (row) #6=12 ("index (row)")) -> (element #1=w1436:dbl[], element #2=w1435:dbl[], element #3=w1434:dbl[], element #4=w1433:dbl[], element #5=w1432:dbl[], element #6=w1431:dbl[])  [unwired: 6 in]
                            n993 = Index Array(array=w1458, index (row)=6) -> (element=w1429:dbl[])  [unwired: 1 in]
                            n994 = local write "Configuração"(w1335) -> ()
                            n995 = Build Array(w1448, w1447, w1446, w1445, w1444, w1443, w1436, w1435, w1434, w1433, w1432, w1431, w1429) -> (w1402:dbl[][])
                            n996 = local write "Gráfico"(w1402) -> ()
                            n997 = local read "Valvulas"() -> (w1404:T2)
                            n998 = Build Array (concatenate)(w1402, w1324, w1323, w1401, w1316) -> (w1400:dbl[][])
                            n999 = call "seletor_adq.vi"("Valvulas"=w1404, "Matriz entrada"=w1400) -> ("matriz saída"=w1403:dbl[][])  [unwired: 3 in]
                            n1000 = Index Array(array=w1458, index (row) #1=0 ("index (row)"), index (row) #2=1 ("index (row)"), index (row) #3=2 ("index (row)"), index (row) #4=3 ("index (row)"), index (row) #5=4 ("index (row)"), index (row) #6=5 ("index (row)"), index (row) #7=6 ("index (row)"), index (row) #8=7 ("index (row)"), index (row) #9=8 ("index (row)"), index (row) #10=9 ("index (row)"), index (row) #11=10 ("index (row)"), index (row) #12=11 ("index (row)"), index (row) #13=12 ("index (row)")) -> (element #1=w1510:dbl[], element #2=w1472:dbl[], element #3=w1471:dbl[], element #4=w1470:dbl[], element #5=w1469:dbl[], element #6=w1468:dbl[], element #7=w1467:dbl[], element #8=w1466:dbl[], element #9=w1465:dbl[], element #10=w1464:dbl[], element #11=w1463:dbl[], element #12=w1462:dbl[], element #13=w1461:dbl[])  [unwired: 13 in]
                            n1001 = local write "Matriz"(w1403) -> ()
                            n1002 = call-poly <vilib>:"Mean.vi"("X"=w1510) -> ("mean"=w1381:dbl)  [unwired: 1 out]
                            n1003 = call-poly <vilib>:"Mean.vi"("X"=w1472) -> ("mean"=w1380:dbl)  [unwired: 1 out]
                            n1004 = call-poly <vilib>:"Mean.vi"("X"=w1471) -> ("mean"=w1379:dbl)  [unwired: 1 out]
                            n1005 = call-poly <vilib>:"Mean.vi"("X"=w1470) -> ("mean"=w1378:dbl)  [unwired: 1 out]
                            n1006 = call-poly <vilib>:"Mean.vi"("X"=w1469) -> ("mean"=w1377:dbl)  [unwired: 1 out]
                            n1007 = call-poly <vilib>:"Mean.vi"("X"=w1468) -> ("mean"=w1376:dbl)  [unwired: 1 out]
                            n1008 = call-poly <vilib>:"Mean.vi"("X"=w1467) -> ("mean"=w1375:dbl)  [unwired: 1 out]
                            n1009 = call-poly <vilib>:"Mean.vi"("X"=w1466) -> ("mean"=w1374:dbl)  [unwired: 1 out]
                            n1010 = call-poly <vilib>:"Mean.vi"("X"=w1465) -> ("mean"=w1373:dbl)  [unwired: 1 out]
                            n1011 = call-poly <vilib>:"Mean.vi"("X"=w1464) -> ("mean"=w1372:dbl)  [unwired: 1 out]
                            n1012 = call-poly <vilib>:"Mean.vi"("X"=w1463) -> ("mean"=w1371:dbl)  [unwired: 1 out]
                            n1013 = call-poly <vilib>:"Mean.vi"("X"=w1462) -> ("mean"=w1370:dbl)  [unwired: 1 out]
                            n1014 = call-poly <vilib>:"Mean.vi"("X"=w1461) -> ("mean"=w1369:dbl)  [unwired: 1 out]
                            n1015 = local write "C2-M corrente"(w1378) -> ()
                            n1016 = local write "C1-M corrente"(w1381) -> ()
                            n1017 = local write "C1-J corrente"(w1380) -> ()
                            n1018 = local write "P1 corrente"(w1379) -> ()
                            n1019 = local write "C2-J corrente"(w1377) -> ()
                            n1020 = local write "P2 corrente"(w1376) -> ()
                            n1021 = local write "Pfundo corrente"(w1375) -> ()
                            n1022 = local write "C3-M corrente"(w1374) -> ()
                            n1023 = local write "C3-J corrente"(w1373) -> ()
                            n1024 = local write "P3 corrente"(w1372) -> ()
                            n1025 = local write "C4-M corrente"(w1371) -> ()
                            n1026 = local write "C4-J corrente"(w1370) -> ()
                            n1027 = local write "P4 corrente"(w1369) -> ()
                            n1028 = local read "SAIR"() -> (w1455:bool)
                            n1029 = local read "STOP"() -> (w1456:bool)
                            n1030 = property on="Pontos No Gráfico" class="Knob (strict)"("DisabledEnum"=T3."Disabled and Grayed Out" ("Disabled")) -> ()  [unwired: 2 in, 2 out]
                            n1031 = Or(x=w1455, y=w1456) -> (x .or. y?=w1457:bool)
                            n1032 = Multiply(x=w1375, y=0.25) -> (x*y=w1362:dbl)
                            n1033 = Multiply(x=w1376, y=0.25) -> (x*y=w1363:dbl)
                            n1034 = Multiply(x=w1371, y=0.25) -> (x*y=w1358:dbl)
                            n1035 = Multiply(x=w1374, y=0.25) -> (x*y=w1361:dbl)
                            n1036 = Multiply(x=w1373, y=0.25) -> (x*y=w1360:dbl)
                            n1037 = Multiply(x=w1372, y=0.25) -> (x*y=w1359:dbl)
                            n1038 = Multiply(x=w1370, y=0.25) -> (x*y=w1357:dbl)
                            n1039 = Multiply(x=w1369, y=0.25) -> (x*y=w1356:dbl)
                            n1040 = Multiply(x=w1378, y=0.25) -> (x*y=w1365:dbl)
                            n1041 = Multiply(x=w1377, y=0.25) -> (x*y=w1364:dbl)
                            n1042 = Multiply(x=w1380, y=0.25) -> (x*y=w1367:dbl)
                            n1043 = Multiply(x=w1379, y=0.25) -> (x*y=w1366:dbl)
                            n1044 = Multiply(x=w1381, y=0.25) -> (x*y=w1368:dbl)
                            n1045 = local write "Visualizar"(TRUE ("VIEW")) -> ()
                            n1046 = local write "led viewing"(TRUE ("visu led")) -> ()
                            n1047 = local write "C1-M"(w1368) -> ()
                            n1048 = local write "C1-J"(w1367) -> ()
                            n1049 = local write "P1"(w1366) -> ()
                            n1050 = local write "C2-M"(w1365) -> ()
                            n1051 = local write "C2-J"(w1364) -> ()
                            n1052 = local write "P2"(w1363) -> ()
                            n1053 = local write "Pfundo"(w1362) -> ()
                            n1054 = local write "C3-M"(w1361) -> ()
                            n1055 = local write "C3-J"(w1360) -> ()
                            n1056 = local write "P3"(w1359) -> ()
                            n1057 = local write "C4-M"(w1358) -> ()
                            n1058 = local write "C4-J"(w1357) -> ()
                            n1059 = local write "P4"(w1356) -> ()
                            "LED adquiri" <- TRUE ("Adquire")
                          }
                          frame #1 {
                            n1060 = Equal?(x=w1573, y=0.0) -> (x = y?=w1572:bool)
                            n1061 = case shown="True" w1572 {
                              frame False {
                              }
                              frame True {
                                n1062 = local read "Matriz"() -> (w1576:dbl[][])
                                n1063 = local write "Matriz 2"(w1576) -> ()
                              }
                            }
                          }
                          frame #2 {
                            n1064 = local read "Matriz 2"() -> (w1578:dbl[][])
                            n1065 = local read "Matriz"() -> (w1579:dbl[][])
                            n1066 = Build Array (concatenate)(w1578, w1579) -> (→"Matriz 2":T6)
                          }
                        }
                        n1067 = local read "TempoAquisicao"() -> (w1283:dbl)
                        n1068 = To Double Precision Float(number=w1285) -> (double precision float=w1282:dbl)
                        n1069 = case shown="True" FALSE {
                          tunnel: [w1303 w1313] -> w1287
                          tunnel: [w1298 w1312] -> w1284
                          tunnel: w1283 -> [w1304 w1311]
                          tunnel: w1282 -> [w1300 w1308]
                          frame False {
                            n1070 = Add(x=w1300, y=2.0) -> (x+y=w1301:dbl)
                            n1071 = Greater Or Equal?(x=w1301, y=w1304) -> (x >= y?=w1303:bool)
                            n1072 = Add(x=w1300, y=1.0) -> (x+y=w1298:dbl)
                          }
                          frame True {
                            n1073 = Multiply(x=3.0 ("y"), y=w1311) -> (x*y=w1306:dbl)
                            n1074 = Subtract(x=w1306, y=2.0) -> (x-y=w1305:dbl)
                            n1075 = Divide(x=w1308, y=3.0) -> (x/y=w1312:dbl)
                            n1076 = Greater Or Equal?(x=w1308, y=w1305) -> (x >= y?=w1313:bool)
                          }
                        }
                        "Timer" <- w1284
                        n1077 = Compound Arithmetic op=OR(w1287, w1289) -> (w1288:bool)
                      }
                    }
                    frame 3 {
                      n1078 = while {
                        tunnel: [w1603] -> w1591
                        shift-right: [w1611] -> w1586
                        shift-left: w1588 -> [w1614]
                        shift-right: [w1612] -> w1585
                        shift-left: w1587 -> [w1613]
                        tunnel: [w1604] -> w1590
                        tunnel: w1589 -> [w1600]
                        tunnel: w1584 -> [w1594]
                        tunnel: w1583 -> [w1593]
                        tunnel: w1582 -> [w1592]
                        i -> [w1598]
                        stop <- w1605 stop-if-true
                        n1079 = flat-sequence {
                          tunnel: w1614 -> [w1820]
                          tunnel: w1613 -> [w1819]
                          tunnel: [w1780] -> w1609
                          tunnel: [w1782] -> w1606
                          tunnel: w1600 -> [w1719]
                          tunnel: w1594 -> [w1652]
                          tunnel: w1593 -> [w1637]
                          tunnel: w1592 -> [w1632]
                          tunnel: w1609 -> [w1882]
                          tunnel: w1596 -> [w1879]
                          tunnel: [w1882] -> w1608
                          tunnel: [w1881] -> w1607
                          tunnel: w1606 -> [w1881]
                          tunnel: [w1887] -> w1611
                          tunnel: [w1888] -> w1612
                          tunnel: w1608 -> [w1888]
                          tunnel: w1607 -> [w1887]
                          frame #0 {
                            # "0-C1-M\n1-C1-J\n2-P1\n3-C2-M\n4-C2-J\n5-P2\n6-C3-M\n7-C3-J\n8-P3\n9-C4-M\n10-C4-J\n11-P4\n12-Pfundo\n13-SKM-WF\n14-FIC-COR\n15-AI-COR\n16-VEL"
                            # "aréa de calculo para conversões e analise se os dados encontrados estão dentro de um padrão aceitavel"
                            # "Interpretação dos valores recebidos de outr\nPC e distribuido conforme a necessidade"
                            # "baseado nas configurações de valvulas abertas\né possível saber com qual tipo de configuração \nestá sendo trabalhado"
                            # "informação em mA é transformada em Tensão"
                            # "indice \"6\" é o Pfundo"
                            # "Coleta de dados da Placa da NATIONAL"
                            # "leituras lindas da placa são colocadas no gráfico"
                            # "SIW-NC-CV-001 05"
                            # "SIK-CV-001 05 04"
                            # "SIT-CV-001 03"
                            # "ADQ 02"
                            # "SPW-WR-VEL 01"
                            # "SPK-WR-VEL 00"
                            n1080 = local write "VALORES UDP"(w1719) -> ()
                            n1081 = Index Array(array=w1719, index #1=0 ("index"), index #2=1 ("index"), index #3=2 ("index"), index #4=3 ("index"), index #5=4 ("index"), index #6=5 ("index"), index #7=10 ("index")) -> (element #1=w1729:string, element #2=w1728:string, element #3=w1727:string, element #4=w1726:string, element #5=w1725:string, element #6=w1724:string, element #7=w1650:string)
                            n1082 = local read "Pfundo corrente"() -> (w1775:dbl)
                            n1083 = local read "P1 corrente"() -> (w1790:dbl)
                            n1084 = local read "P2 corrente"() -> (w1789:dbl)
                            n1085 = local read "P3 corrente"() -> (w1788:dbl)
                            n1086 = local read "P4 corrente"() -> (w1778:dbl)
                            n1087 = call "CONVERSOR.vi"("String"=w1729) -> ("float"=w1653:dbl)  [unwired: 6 in, 3 out]
                            n1088 = local write "JK(m/s)"(w1653) -> ()
                            n1089 = call "CONVERSOR.vi"("String"=w1728) -> ("float"=w1654:dbl)  [unwired: 6 in, 3 out]
                            n1090 = local write "JW(m/s)"(w1654) -> ()
                            n1091 = call "CONVERSOR.vi"("String"=w1727) -> ()  [unwired: 6 in, 4 out]
                            n1092 = call "CONVERSOR.vi"("String"=w1726) -> ("boolean"=w1722:bool)  [unwired: 6 in, 3 out]
                            "Linha de Teste" <- w1722
                            n1093 = call "CONVERSOR.vi"("String"=w1725) -> ("boolean"=w1721:bool)  [unwired: 6 in, 3 out]
                            n1094 = local write "SIK-CV-001"(w1721) -> ()
                            n1095 = call "CONVERSOR.vi"("String"=w1724) -> ("boolean"=w1720:bool)  [unwired: 6 in, 3 out]
                            n1096 = local write "SIW-CV-001"(w1720) -> ()
                            n1097 = call "CONVERSOR.vi"("String"=w1650) -> ("boolean"=w1649:bool)  [unwired: 6 in, 3 out]
                            n1098 = local write "SKS-NC-CV-006"(w1649) -> ()
                            n1099 = call "variação_pressao_adq.vi"("P1(mA)"=w1790, "P2(mA)"=w1789, "P3(mA)"=w1788, "P4(mA)"=w1778, "PFUNDO(mA)"=w1775, "JW(m/s)"=w1654, "JK(m/s)"=w1653, "Valores"=w1652, "SIK-CV-001"=w1721, "SIW-CV-001"=w1720) -> ("P12/L12"=→"P12/L [Pa/m]":dbl, "P34/L34"=→"P34/L [Pa/m]":dbl, "P23/L23"=→"P23/L [Pa/m]":dbl, "P2(kPa)"=w1657:dbl, "VALOR TEORICO"=w1791:dbl, "P3(kPa)"=w1656:dbl, "P1(kPa)"=w1658:dbl, "P4(kPa)"=w1655:dbl, "P1-P2G"=→"P1-P2 VERDE":bool, "P2-P3R"=→"P2-P3 RED":bool, "P2-P3G"=→"P2-P3 VERDE":bool, "P1-P2R"=→"P1-P2 RED":bool, "P3-P4G"=→"P3-P4 VERDE":bool, "P3-P4R"=→"P3-P4 RED":bool, "PFUNDO(kPa)"=w1631:dbl)  [unwired: 3 in]
                            "P4(kPa)" <- w1655
                            "P3(kPa)" <- w1656
                            "P2(kPa)" <- w1657
                            "P1(kPa)" <- w1658
                            "Pfundo(kPa)" <- w1631
                            n1100 = local read "ValoresEnviados"() -> (w1636:cluster{"Pfundo[kPa]":dbl})
                            n1101 = call "check-up_adq.vi"("JK(m/s)"=w1653, "JW(m/s)"=w1654, "P4(kPa)"=w1655, "P3(kPa)"=w1656, "P2(kPa)"=w1657, "P1(kPa)"=w1658) -> ("OK 2 R"=→"OK2 R":bool, "OK 2 G"=→"OK2":bool, "OK RED"=→"Ok R":bool, "OK G"=→"Ok":bool)  [unwired: 2 in]
                            n1102 = Bundle By Name(cluster=w1636, "Pfundo[kPa]"=w1631) -> (w1638:cluster{"Pfundo[kPa]":dbl})
                            n1103 = case shown="False" w1722 {
                              tunnel: w1791 -> [_ w1855]
                              frame False {
                                n1104 = local write "Valor Teórico[Pa/m]"(nan) -> ()
                              }
                              frame True {
                                "Valor Teórico[Pa/m]" <- w1855
                              }
                            }
                            n1105 = invoke class="VI" method="Ctrl Val.Set"(reference=w1637, "Control Name"="ValoresEnviados", "Value"=w1636) -> ()  [unwired: 2 in, 5 out]
                            n1106 = local write "ValoresEnviados"(w1638) -> ()
                            n1107 = case shown="True" TRUE {
                              tunnel: [w1851 w1853] -> w1765
                              tunnel: [w1836 w1852] -> w1764
                              tunnel: w1654 -> [_ w1853]
                              tunnel: w1653 -> [_ w1852]
                              frame False {
                                n1108 = local read "Escala de Calibracao - SKM-FI-WF"() -> (w1845:cluster{"Escala Max":dbl, "Escala Min":dbl})
                                n1109 = local read "Entrada - SKM-FI-WF [CLP]"() -> (w1843:dbl)
                                n1110 = local read "SKM-FIC-KF_CORIOLI [kg/s]"() -> (w1834:dbl)
                                n1111 = local read "SKM-AI-KF_CORIOLI [kg/m³]"() -> (w1833:dbl)
                                n1112 = local read "Escala de Calibracao - SKM-FI-WF"() -> (w1839:cluster{"Escala Max":dbl, "Escala Min":dbl})
                                n1113 = Bundle By Name(cluster=w1839, "Escala Max"=0.001805556, "Escala Min"=0.0 ("Escala Max")) -> (w1840:cluster{"Escala Max":dbl, "Escala Min":dbl})
                                n1114 = local write "Escala de Calibracao - SKM-FI-WF"(w1840) -> ()
                                n1115 = Unbundle By Name(w1845) -> ("Escala Max"=w1846:dbl, "Escala Min"=w1844:dbl)
                                n1116 = Divide(x=w1834, y=w1833) -> (x/y=w1835:dbl)
                                n1117 = Divide(x=w1835, y=0.0005107051557) -> (x/y=w1836:dbl)
                                n1118 = Subtract(x=w1846, y=w1844) -> (x-y=w1847:dbl)
                                n1119 = Divide(x=w1847, y=4096.0) -> (x/y=w1848:dbl)
                                n1120 = Multiply(x=w1848, y=w1843) -> (x*y=w1849:dbl)
                                n1121 = Add(x=w1849, y=w1844) -> (x+y=w1850:dbl)
                                n1122 = Divide(x=w1850, y=0.0005107051557) -> (x/y=w1851:dbl)
                              }
                              frame True {
                                # "devido a mudança do sistema para não ler valores do CLP , e sim de outro PC\nesse CASE deve ser mantido como TRUE até ordens de mudanças"
                              }
                            }
                            n1123 = Index Array(array=w1719, index #1=6 ("index"), index #2=7 ("index"), index #3=8 ("index"), index #4=9 ("index")) -> (element #1=w1715:string, element #2=w1714:string, element #3=w1713:string, element #4=w1703:string)
                            n1124 = call "CONVERSOR.vi"("String"=w1715) -> ("float"=w1635:dbl)  [unwired: 6 in, 3 out]
                            n1125 = call "CONVERSOR.vi"("String"=w1714) -> ("float"=w1634:dbl)  [unwired: 6 in, 3 out]
                            n1126 = call "CONVERSOR.vi"("String"=w1713) -> ("float"=w1633:dbl)  [unwired: 6 in, 3 out]
                            n1127 = call "CONVERSOR.vi"("String"=w1703) -> ("float"=w1702:dbl)  [unwired: 6 in, 3 out]
                            n1128 = local write "JG(m/s)"(w1702) -> ()
                            n1129 = local write "SKM-FIC-KF-COR"(w1634) -> ()
                            n1130 = local write "SKM-AI-KF-COR"(w1633) -> ()
                            n1131 = local write "SKM-FI-WF"(w1635) -> ()
                            n1132 = local write "JW(m/s)"(w1765) -> ()
                            n1133 = local write "JK(m/s)"(w1764) -> ()
                            n1134 = call <vilib>:"DAQmx Start Task.vi"("task/channels in"=w1820, "error in"=w1819) -> ("task out"=w1793:refnum<k21>, "error out"=w1792:errorcluster)  [unwired: 12 in]
                            n1135 = local write "SIW-CV-001"(w1720) -> ()
                            n1136 = local write "SIK-CV-001"(w1721) -> ()
                            n1137 = local read "Aplicação"() -> (w1641:string)
                            n1138 = Build Array(w1720, w1721) -> (w1774:bool[])
                            n1139 = call-poly <vilib>:"DAQmx Read.vi"("task/channels in"=w1793, "number of samples per channel"=3000, "timeout"=10.0, "error in"=w1792) -> ("task out"=w1781:refnum<k21>, "data"=w1777:dbl[][], "error out"=w1779:errorcluster)  [unwired: 9 in]
                            n1140 = Equal?(x=w1641, y="Deslocamento_Retirada_por_Baixo") -> (x = y?=w1645:bool)
                            n1141 = Equal?(x=w1641, y="Deslocamento_Retirada_por_Cima") -> (x = y?=w1644:bool)
                            n1142 = Boolean Array To Number(Boolean array=w1774) -> (number=w1643:u32)
                            n1143 = for {
                              N: 3000 -> [_]
                              tunnel: [w1862] -> w1712 mode=indexing
                              tunnel: w1643 -> [w1863]
                              tunnel: [w1861] -> w1711 mode=indexing
                              tunnel: [w1860] -> w1710 mode=indexing
                              tunnel: [w1859] -> w1709 mode=indexing
                              tunnel: w1635 -> [w1858]
                              tunnel: w1634 -> [w1857]
                              tunnel: w1633 -> [w1856]
                              tunnel: w1632 -> [_]
                              n1144 = case shown="0, Default" w1863 {
                                tunnel: [w1864 w1868 w1872] -> w1862
                                tunnel: [w1864 w1867 w1871] -> w1861
                                tunnel: [w1864 w1866 w1870] -> w1860
                                tunnel: [w1864 w1865 w1869] -> w1859
                                tunnel: w1858 -> [_ w1867 w1871]
                                tunnel: w1857 -> [_ w1866 w1870]
                                tunnel: w1856 -> [_ w1865 w1869]
                                frame 0, Default {
                                w1864 = nan
                                }
                                frame 1 {
                                n1145 = local read "JW(m/s)"() -> (w1868:dbl)
                                }
                                frame 2 {
                                n1146 = local read "JK(m/s)"() -> (w1872:dbl)
                                }
                              }
                            }
                            n1147 = Build Array(w1645, w1644) -> (w1646:bool[])
                            n1148 = Boolean Array To Number(Boolean array=w1646) -> (number=w1642:u32)
                            n1149 = case shown="0, Default" w1642 {
                              tunnel: w1643 -> [_ w1822 w1828]
                              tunnel: ["No Conf." w1823 w1827] -> w1640
                              frame 0, Default {
                              }
                              frame 1 {
                                n1150 = case shown="0, Default" w1822 {
                                tunnel: ["No Conf." "C1" "C2"] -> w1823
                                frame 0, Default {
                                }
                                frame 1 {
                                }
                                frame 2 {
                                }
                                }
                              }
                              frame 2 {
                                n1151 = case shown="0, Default" w1828 {
                                tunnel: ["No Conf." "C3" "C4"] -> w1827
                                frame 0, Default {
                                }
                                frame 1 {
                                }
                                frame 2 {
                                }
                                }
                              }
                            }
                            n1152 = for {
                              tunnel: w1777 -> [w1874] mode=indexing
                              tunnel: [w1873] -> w1763 mode=indexing
                              n1153 = for {
                                tunnel: w1874 -> [w1877] mode=indexing
                                tunnel: [w1875] -> w1873 mode=indexing
                                n1154 = Multiply(x=w1877, y=1000.0) -> (x*y=w1875:dbl)
                              }
                            }
                            n1155 = Index Array(array=w1763, index (row)=12) -> (element=w1806:dbl[])  [unwired: 1 in]
                            n1156 = Index Array(array=w1763, index (row)=0) -> (element=w1812:dbl[])  [unwired: 1 in]
                            n1157 = Index Array(array=w1763, index (row)=1) -> (element=w1818:dbl[])  [unwired: 1 in]
                            n1158 = Index Array(array=w1763, index (row)=2) -> (element=w1817:dbl[])  [unwired: 1 in]
                            n1159 = Index Array(array=w1763, index (row)=3) -> (element=w1816:dbl[])  [unwired: 1 in]
                            n1160 = Index Array(array=w1763, index (row)=4) -> (element=w1815:dbl[])  [unwired: 1 in]
                            n1161 = Index Array(array=w1763, index (row)=5) -> (element=w1814:dbl[])  [unwired: 1 in]
                            n1162 = Index Array(array=w1763, index (row)=6) -> (element=w1813:dbl[])  [unwired: 1 in]
                            n1163 = Index Array(array=w1763, index (row)=7) -> (element=w1811:dbl[])  [unwired: 1 in]
                            n1164 = Index Array(array=w1763, index (row)=8) -> (element=w1810:dbl[])  [unwired: 1 in]
                            n1165 = Index Array(array=w1763, index (row)=9) -> (element=w1809:dbl[])  [unwired: 1 in]
                            n1166 = Index Array(array=w1763, index (row)=10) -> (element=w1808:dbl[])  [unwired: 1 in]
                            n1167 = Index Array(array=w1763, index (row)=11) -> (element=w1807:dbl[])  [unwired: 1 in]
                            n1168 = call-poly <vilib>:"Mean.vi"("X"=w1812) -> ("mean"=w1664:dbl)  [unwired: 1 out]
                            "C1-M corrente" <- w1664
                            n1169 = call-poly <vilib>:"Mean.vi"("X"=w1818) -> ("mean"=w1663:dbl)  [unwired: 1 out]
                            "C1-J corrente" <- w1663
                            n1170 = call-poly <vilib>:"Mean.vi"("X"=w1817) -> ("mean"=w1688:dbl)  [unwired: 1 out]
                            "P1 corrente" <- w1688
                            n1171 = call-poly <vilib>:"Mean.vi"("X"=w1816) -> ("mean"=w1687:dbl)  [unwired: 1 out]
                            "C2-M corrente" <- w1687
                            n1172 = call-poly <vilib>:"Mean.vi"("X"=w1815) -> ("mean"=w1686:dbl)  [unwired: 1 out]
                            "C2-J corrente" <- w1686
                            n1173 = call-poly <vilib>:"Mean.vi"("X"=w1814) -> ("mean"=w1685:dbl)  [unwired: 1 out]
                            "P2 corrente" <- w1685
                            n1174 = call-poly <vilib>:"Mean.vi"("X"=w1813) -> ("mean"=w1684:dbl)  [unwired: 1 out]
                            "Pfundo corrente" <- w1684
                            n1175 = call-poly <vilib>:"Mean.vi"("X"=w1811) -> ("mean"=w1683:dbl)  [unwired: 1 out]
                            "C3-M corrente" <- w1683
                            n1176 = call-poly <vilib>:"Mean.vi"("X"=w1810) -> ("mean"=w1682:dbl)  [unwired: 1 out]
                            "C3-J corrente" <- w1682
                            n1177 = call-poly <vilib>:"Mean.vi"("X"=w1809) -> ("mean"=w1681:dbl)  [unwired: 1 out]
                            "P3 corrente" <- w1681
                            n1178 = call-poly <vilib>:"Mean.vi"("X"=w1808) -> ("mean"=w1680:dbl)  [unwired: 1 out]
                            "C4-M corrente" <- w1680
                            n1179 = call-poly <vilib>:"Mean.vi"("X"=w1807) -> ("mean"=w1679:dbl)  [unwired: 1 out]
                            "C4-J corrente" <- w1679
                            n1180 = call-poly <vilib>:"Mean.vi"("X"=w1806) -> ("mean"=w1678:dbl)  [unwired: 1 out]
                            "P4 corrente" <- w1678
                            n1181 = local write "Configuração"(w1640) -> ()
                            n1182 = Multiply(x=w1684, y=0.25) -> (x*y=→"Pfundo":dbl)
                            n1183 = Multiply(x=w1685, y=0.25) -> (x*y=→"P2":dbl)
                            n1184 = Multiply(x=w1680, y=0.25) -> (x*y=→"C4-M":dbl)
                            n1185 = Multiply(x=w1683, y=0.25) -> (x*y=→"C3-M":dbl)
                            n1186 = Multiply(x=w1682, y=0.25) -> (x*y=→"C3-J":dbl)
                            n1187 = Multiply(x=w1681, y=0.25) -> (x*y=→"P3":dbl)
                            n1188 = Multiply(x=w1679, y=0.25) -> (x*y=→"C4-J":dbl)
                            n1189 = Multiply(x=w1678, y=0.25) -> (x*y=→"P4":dbl)
                            n1190 = Multiply(x=w1687, y=0.25) -> (x*y=→"C2-M":dbl)
                            n1191 = Multiply(x=w1686, y=0.25) -> (x*y=→"C2-J":dbl)
                            n1192 = Multiply(x=w1663, y=0.25) -> (x*y=→"C1-J":dbl)
                            n1193 = Multiply(x=w1688, y=0.25) -> (x*y=→"P1":dbl)
                            n1194 = Multiply(x=w1664, y=0.25) -> (x*y=→"C1-M":dbl)
                            n1195 = call <vilib>:"DAQmx Stop Task.vi"("task/channels in"=w1781, "error in"=w1779) -> ("task out"=w1782:refnum<k21>, "error out"=w1780:errorcluster)  [unwired: 12 in]
                            n1196 = Index Array(array=w1763, index (row) #1=0 ("index (row)"), index (row) #2=1 ("index (row)"), index (row) #3=2 ("index (row)"), index (row) #4=3 ("index (row)"), index (row) #5=4 ("index (row)"), index (row) #6=5 ("index (row)")) -> (element #1=w1755:dbl[], element #2=w1754:dbl[], element #3=w1753:dbl[], element #4=w1752:dbl[], element #5=w1751:dbl[], element #6=w1750:dbl[])  [unwired: 6 in]
                            n1197 = Index Array(array=w1763, index (row) #1=7 ("index (row)"), index (row) #2=8 ("index (row)"), index (row) #3=9 ("index (row)"), index (row) #4=10 ("index (row)"), index (row) #5=11 ("index (row)"), index (row) #6=12 ("index (row)")) -> (element #1=w1743:dbl[], element #2=w1742:dbl[], element #3=w1741:dbl[], element #4=w1740:dbl[], element #5=w1739:dbl[], element #6=w1738:dbl[])  [unwired: 6 in]
                            n1198 = Index Array(array=w1763, index (row)=6) -> (element=w1736:dbl[])  [unwired: 1 in]
                            n1199 = local read "Valvulas"() -> (w1762:T2)
                            n1200 = Build Array(w1755, w1754, w1753, w1752, w1751, w1750, w1743, w1742, w1741, w1740, w1739, w1738, w1736) -> (w1706:dbl[][])
                            n1201 = property on="Pontos No Gráfico" class="Knob (strict)"("DisabledEnum"=T3."Disabled and Grayed Out" ("Disabled")) -> ()  [unwired: 2 in, 2 out]
                            n1202 = local write "led viewing"(TRUE ("visu led")) -> ()
                            n1203 = Build Array (concatenate)(w1706, w1711, w1710, w1709, w1712) -> (w1707:dbl[][])
                            n1204 = call "seletor_adq.vi"("Valvulas"=w1762, "Matriz entrada"=w1707) -> ("matriz saída"=w1708:dbl[][])  [unwired: 3 in]
                            n1205 = local write "Gráfico"(w1706) -> ()
                            n1206 = local write "Matriz"(w1708) -> ()
                          }
                          frame #1 {
                            n1207 = Equal?(x=w1879, y=0.0) -> (x = y?=w1878:bool)
                            n1208 = case shown="True" w1878 {
                              frame False {
                              }
                              frame True {
                                n1209 = local read "Matriz"() -> (w1883:dbl[][])
                                n1210 = local write "Matriz 2"(w1883) -> ()
                              }
                            }
                          }
                          frame #2 {
                            n1211 = local read "Matriz 2"() -> (w1886:dbl[][])
                            n1212 = local read "Matriz"() -> (w1885:dbl[][])
                            n1213 = Build Array (concatenate)(w1886, w1885) -> (w1884:T6)
                            n1214 = local write "Matriz 2"(w1884) -> ()
                          }
                        }
                        n1215 = Or(x="SAIR", y="STOP") -> (x .or. y?=w1603:bool)
                        n1216 = To Double Precision Float(number=w1598) -> (double precision float=w1596:dbl)
                        n1217 = case shown="False" FALSE {
                          tunnel: [w1620 w1630] -> w1604
                          tunnel: [w1615 w1629] -> w1599
                          tunnel: "TempoAquisicao" -> [w1621 w1626]
                          tunnel: w1596 -> [w1617 w1625]
                          frame False {
                            n1218 = Add(x=w1617, y=2.0) -> (x+y=w1618:dbl)
                            n1219 = Greater Or Equal?(x=w1618, y=w1621) -> (x >= y?=w1620:bool)
                            n1220 = Add(x=w1617, y=1.0) -> (x+y=w1615:dbl)
                          }
                          frame True {
                            n1221 = Multiply(x=w1626, y=3.0) -> (x*y=w1624:dbl)
                            n1222 = Divide(x=w1625, y=3.0) -> (x/y=w1629:dbl)
                            n1223 = Subtract(x=w1624, y=2.0) -> (x-y=w1622:dbl)
                            n1224 = Greater Or Equal?(x=w1625, y=w1622) -> (x >= y?=w1630:bool)
                          }
                        }
                        n1225 = local write "Timer"(w1599) -> ()
                        n1226 = Compound Arithmetic op=OR(w1604, w1603) -> (w1605:bool)
                        n1227 = local write "LED adquiri"(TRUE ("adq")) -> ()
                      }
                    }
                  }
                  n1228 = call <vilib>:"DAQmx Clear Task.vi"("task in"=w994, "error in"=w993) -> ("error out"=→"error out":errorcluster)  [unwired: 13 in]
                  "DAQmx Task Name" <- w1000
                }
              }
              n1229 = Compound Arithmetic op=OR(w154, w155) -> (w156:bool)
            }
            n1230 = invoke class="VI" method="Abort VI"(reference=w94) -> ()  [unwired: 2 in, 3 out]
          }
          frame #2 {
            n1231 = local read "SAIR"() -> (w1912:bool)
            n1232 = case shown="False" w1912 {
              frame False {
                # "salva em arquivo TXT tabela de\ndados com o nome ja montado"
                # "adiciona o índice nome do arquivo"
                # "Valores de entrada de velocidades para salvar no nome do arquivo\nVi também recebe o nome da configuração"
                # "Abre o diretório\"DADOS\" para armazenar os dados"
                # "Criação e edição dos nomes dos arquivos"
                n1233 = Current VI's Path() -> (path=w1939:path)
                n1234 = Strip Path(path=w1939) -> (stripped path=w1938:path)  [unwired: 1 out]
                n1235 = Build Path(base path=w1938, name or relative path="dados") -> (appended path=w1924:path)
                n1236 = call <vilib>:"Check if File or Folder Exists.vi"("path"=w1924) -> ("file or folder exists?"=w1926:bool, "dup path"=w1925:path)  [unwired: 8 in, 1 out]
                n1237 = case shown="True" w1926 {
                  tunnel: w1925 -> [w1957 w1958]
                  tunnel: [w1956 w1958] -> w1923
                  frame False {
                    n1238 = Create Folder(path (use dialog)=w1957) -> (created path=w1956:path)  [unwired: 2 in, 2 out]
                  }
                  frame True {
                  }
                }
                n1239 = local read "JW(m/s)"() -> (w1950:dbl)
                n1240 = local read "JG(m/s)"() -> (w1936:dbl)
                n1241 = local read "JK(m/s)"() -> (w1949:dbl)
                n1242 = Build Array("SIW-CV-001", "SIK-CV-001") -> (w1951:bool[])
                n1243 = Number To Fractional String(number=w1950, precision (6)=i16 2) -> (F-format string=w1934:string)  [unwired: 2 in]
                n1244 = Number To Fractional String(number=w1949, precision (6)=i16 2) -> (F-format string=w1933:string)  [unwired: 2 in]
                n1245 = Number To Fractional String(number=w1936, precision (6)=i16 2) -> (F-format string=w1932:string)  [unwired: 2 in]
                n1246 = Boolean Array To Number(Boolean array=w1951) -> (number=w1955:u32)
                n1247 = case shown="0, Default" w1955 {
                  tunnel: ["No-Conf." "C1" "C2"] -> w1935
                  frame 0, Default {
                  }
                  frame 1 {
                  }
                  frame 2 {
                  }
                }
                n1248 = local read "Valvulas"() -> (w1930:T2)
                n1249 = Unbundle By Name(w1930) -> ("JW"=w1929:bool, "JK"=w1928:bool, "JG"=w1927:bool)
                n1250 = call "nome_arquivo_adq.vi"("caminho"=w1923, "Configuração"=w1935, 7:"JW"=w1934, 9:"JK"=w1933, 11:"JG"=w1932, 12:"JW"=w1929, 13:"JK"=w1928, 14:"JG"=w1927) -> ("resulting string"=w1931:string)  [unwired: 7 in]
                n1251 = local read "Quantidade de\narquivos adquiridos"() -> (w1946:i64)
                n1252 = Current VI's Path() -> (path=w1921:path)
                n1253 = Increment(x=w1946) -> (x+1=w1940:i64)
                n1254 = Format Into String(format string="%s%d%s", initial string=w1931, "_" ("input 1"), w1940, ".txt" ("substring (\"\")")) -> (resulting string=w1942:string)  [unwired: 1 in, 1 out]
                n1255 = String To Path(string=w1942) -> (path=w1941:path)
                n1256 = local write "Quantidade de\narquivos adquiridos"(w1940) -> ()
                n1257 = local read "Matriz 2"() -> (w1954:dbl[][])
                n1258 = Strip Path(path=w1921) -> (stripped path=w1922:path)  [unwired: 1 out]
                n1259 = Build Path(base path=w1922, name or relative path="titulo.txt") -> (appended path=w1919:path)
                n1260 = Transpose 2D Array(2D array=w1954) -> (transposed array=w1917:dbl[][])
                n1261 = call-poly <vilib>:"Read Delimited Spreadsheet.vi"("file path (dialog if empty)"=w1919) -> ("first row"=w1916:string[])  [unwired: 9 in, 5 out]
                n1262 = Number To Fractional String(number=w1917, precision (6)=i16 4) -> (F-format string=w1915:string[][])  [unwired: 2 in]
                n1263 = Build Array (concatenate)(w1916, w1915) -> (w1914:string[][])
                n1264 = call-poly <vilib>:"Write Delimited Spreadsheet.vi"("file path (dialog if empty)"=w1941, "2D data"=w1914) -> ()  [unwired: 12 in, 2 out]
              }
              frame True {
                # "Se estiver na posição SAIR, não será gravado arquivo nenhum"
              }
            }
          }
          frame #3 {
            w1962 = FALSE ("Visualisa")
            # "botoões paara posição default"
            n1265 = flat-sequence {
              frame #0 {
                # "para VI de comunicação com outro PC\nessa VI necessita se parada somento dessa meneira, de outro modo, dará erro"
                n1266 = local read "reference out"() -> (w1969:refnum<vi>)
                n1267 = To Variant(anything=TRUE) -> (Variant=w1966:variant)
                n1268 = invoke class="VI" method="Ctrl Val.Set"(reference=w1969, "Control Name"="STOP", "Value"=w1966) -> ()  [unwired: 2 in, 5 out]
                n1269 = Wait (ms)(milliseconds to wait=u32 500) -> ()  [unwired: 1 out]
              }
            }
            n1270 = local write "COMEÇAR"(w1962) -> ()
            n1271 = local write "STOP"(w1962) -> ()
            n1272 = local write "Visualizar"(w1962) -> ()
            n1273 = local write "LED adquiri"(w1962) -> ()
            n1274 = local write "P1-P2 VERDE"(w1962) -> ()
            n1275 = local write "P1-P2 RED"(w1962) -> ()
            n1276 = local write "P2-P3 VERDE"(w1962) -> ()
            n1277 = local write "P2-P3 RED"(w1962) -> ()
            n1278 = local write "P3-P4 VERDE"(w1962) -> ()
            n1279 = local write "P3-P4 RED"(w1962) -> ()
            n1280 = local write "led viewing"(w1962) -> ()
            n1281 = local write "OK2"(w1962) -> ()
            n1282 = local write "OK2 R"(w1962) -> ()
            n1283 = local write "Ok"(w1962) -> ()
            n1284 = local write "Ok R"(w1962) -> ()
            n1285 = local write "Aquisição Automática"(w1962) -> ()
            n1286 = local write "comunica funcionando"(w1962) -> ()
            n1287 = global write "comunicacao.vi" "comunicacao"(TRUE ("comunicacao")) -> ()
            n1288 = local read "SAIR"() -> (w1964:bool)
          }
        }
      }
    }
    frame #1 {
      # "Como a VI \"abre aplicacção\" é a ultima a ser fechada\napós o termino do addquiri, será aberto ela denovo \npara caso o usurário deseje realizar outra aquisição \ncom outra aplicação, ou alterar alguma configuração"
      # "fecha VI"
      n1289 = property class="VI"(error in=w1971, "Front Panel.Open"=FALSE ("Front Panel Window:Open")) -> ()  [unwired: 1 in, 2 out]
      n1290 = Current VI's Path() -> (path=w1978:path)
      n1291 = Strip Path(path=w1978) -> (stripped path=w1972:path)  [unwired: 1 out]
      n1292 = Build Path(base path=w1972, name or relative path="abre_aplicacao_adq.vi") -> (appended path=w1976:path)
      n1293 = Open VI Reference(vi path=w1976) -> (vi reference=w1975:refnum<vi>)  [unwired: 5 in, 1 out]
      n1294 = invoke class="VI" method="Run VI"(reference=w1975, "Wait until done"=FALSE ("Wait Until Done"), "Auto Dispose Ref"=FALSE ("Auto Dispose Reference")) -> ()  [unwired: 2 in, 5 out]
    }
  }
